vi "MainKinetics.vi"() -> ()   [LabVIEW 2017]
uses:
  <vilib>/Utility/miscctls.llb/LVRowAndColumnTypeDef.ctl
  <vilib>/Utility/sysdir.llb/System Directory Type.ctl
  <vilib>/Utility/config.llb/Read Key (String).vi
  <vilib>/Utility/config.llb/Write Key (String).vi
  <vilib>/Utility/cursorutil.llb/Set Cursor (Icon Pict).vi
  PCAN_Driver/ControlCAN.lvlib
  <vilib>/Utility/config.llb/NI_LVConfig.lvlib
panel:
  out "CurrentSens":bool
  out "CurrentOut":dbl
  out "Current":string
  out "VISA Current":refnum<visa-resource-name>
  out "Offset":dbl
  out "Analogtest":bool=TRUE
  out "TestinExecution":string
  out "FullSpeed2 Current":dbl
  out "FullSpeed1 Current":dbl
  out "String":string
  out "ParamVersion":string
  out "DSP Board S/N":string
  out "POWER Board S/N":string caption="DRIVER Board S/N"
  in  "EventTimeout":i32=100
  out "SpeedLimit":dbl[](array[numeric])
  out "TestArray":string[](array[string])
  out "Motor Speed RPM Serial":dbl
  out "DAQmx Device Name":tag
  out "PN":string
  out "FileName":string
  out "VenableSpeed":u16
  out "TesterVersion":string
  out "ClosePanel":bool=TRUE
  out "UUT SN Report":string
  out "Automation":bool
  out "Test Failed":bool
  out "VisualInspectionResult":bool
  out "MotorTempResult":bool
  out "VenableDirectionResult":bool
  out "VenableResult":bool
  out "ComTestResult":bool=TRUE
  out "UUT SoftwareVer":string
  out "Next SN":i32
  in  "SetSN":bool
  out "Current SN":i32
  out "FullSpeed2 Speed":dbl
  out "FullSpeed2 Current":dbl
  out "FullSpeed1 Current":dbl
  out "FullSpeed1 Speed":dbl
  out "UUT":u8
  out "CAN Status":bool
  out "Array":u64[][](array[numeric]) format="%016x"
  out "Motor Phase Current RMS":dbl
  out "Ambient Temperature":dbl
  out "Speed error":bool
  out "Commutation err":bool
  out "Under voltage/Over voltage":bool
  out "Derated drive temp":bool
  out "Motor Over temperature":bool
  out "Motor Sensor temp Fauilre":bool
  out "Drive Over temperature":bool
  out "Drive Sensor temp Failure":bool
  out "Ambient Over temp":bool
  out "Ambient Sensor temp":bool
  out "DC Voltage":dbl
  out "DC Current":dbl
  out "Power transistor Heat sink Temp.":dbl
  out "Motor Stator Temp.":dbl
  out "Motor Speed RPM":dbl
  out "ECS State":u16
  out "UUT":string="EBAY"
  in  "Logger Path":path
  in  "Report":bool
  in  "Start":bool
  in  "ATR":string[][](table)=[["Test Communication", "-", "-", "-", "-", ""], ["Set S/N", "-", "-", "-", "-", ""], ["Set Board Number", "-", "-", "-", "-", ""], [" ", "", "", "", "", ""], ["Test Communication", "-", "-", "-", "-", ""], ["Get S/N", "-", "-", "-", "", ""], ["Get Board Number", "-", "-", "-", "", ""], ["Get FW", "-", "-", "-", "", ""], ["Enable Motor", "", "", "", "", ""], ["Small position command", "", "", "", "", ""], ["Measure delta", "", "", "", "", ""], ["Velocity command", "", "", "", "", ""]]
  in  "Settings":bool
  in  "Refresh Button":bool
  out "Serial Status":bool
  in  "VISA Kinetics":refnum<visa-resource-name>="COM6"
  in  "Serial Com":bool
  in  "Help Button":bool
  out "Pannel User Message":string
  in  "Stop Button":bool
  # "Kinetics"
  # "REDLER TECHNOLOGIES LTD"
  # "ver 1.2p"
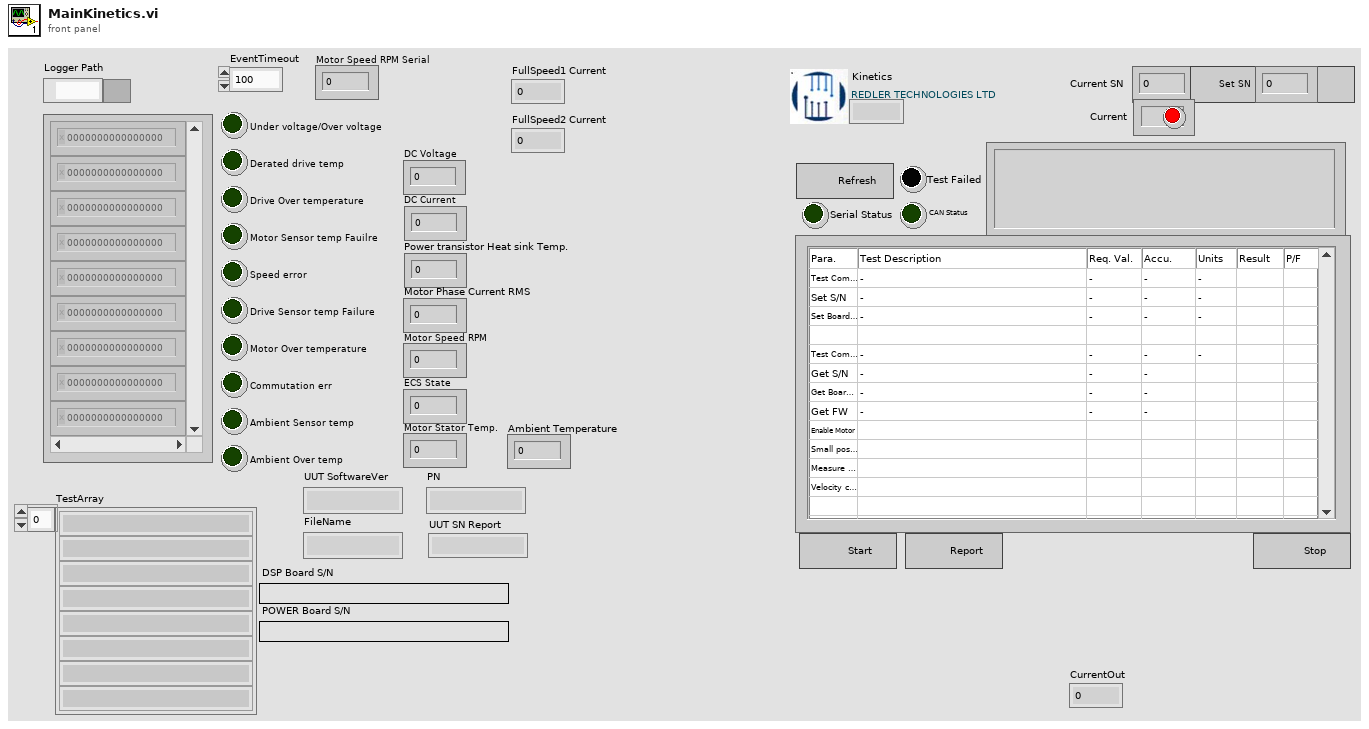
[diagram p1: front panel]
types:
  T1 = cluster{"VISA":refnum<visa-resource-name>, "TestArray":string[]}
  T2 = cluster{"ID":u32, "MSGTYPE":u8, "LEN":u8, "aDATA":u8[]}[]
  T3 = enum16{"Erase ATR Table", "Stop", "MainProgram", "Initialize"}
  T4 = typedef "NI_LVConfig.lvlib/Config Data RefNum.ctl" = refnum<k1>
  T5 = enum16{"Init", "0 ohm", "6 ohm", "13.2 ohm", "15 ohm", "25.9 ohm", "33 ohm", "Down", "Up", "Venable", "Firmware", "PowerSuply"}
  T6 = enum16{"Wait", "Exit", "VC=0", "ReadVC", "VC=1000"}
  T7 = enum16{"Stop", "Result", "FullSpeed2", "MD[1]=1", "FullSpeed1", "MD[1]=0"}
  T8 = enum16{"K15", "K16", "K17", "Venable", "Firmeware", "Fan", "Power", "120C", "110C", "100C", "90C", "80C", "70C", "60C", "50C", "40C", "30C", "25C", "20C", "10C", "0C"}
  T9 = enum8{"Term1", "Term2", "Current", "Fan", "TempCPU"}
  T10 = enum16{"Exit", "AI0/3", "AO0", "Wait", "Read", "Init"}
  T11 = enum16{"Exit", "Wait", "ReadCurrent", "ReadTemp", "Init"}
  T12 = enum16{"Init", "0 ohm", "6 ohm", "13.2 ohm", "15 ohm", "25.9 ohm", "33 ohm", "Down", "Up", "Venable", "Firmware", "PowerSuply"}[]
  T13 = enum8{"Enabled", "Disabled", "Disabled and Grayed Out"}
  T14 = typedef "LVRowAndColumnTypeDef.ctl" = cluster{"Row":i32, "Column":i32}
  T15 = enum32{"Invalid", "Standard", "Closed", "Hidden", "Minimized", "Maximized"}
  T16 = cluster{"ID":u32, "MSGTYPE":u8, "LEN":u8, "aDATA":u8[]}
  T17 = enum16{"open", "replace", "create", "open or create", "replace or create", "replace or create with confirmation"}
  T18 = typedef "ControlCAN.lvlib/DevType.ctl" = u32
  T19 = typedef "ControlCAN.lvlib/CAN Channel.ctl" = u32
  T20 = typedef "ControlCAN.lvlib/VCI_INIT_CONFIG.ctl" = cluster{"AccCode":u32, "AccMask":u32, "InitFlag":T21, "Fliter":T22, "Timing0":u8, "Timing1":u8, "Mode":T23}
  T21 = typedef "ControlCAN.lvlib/InitFlag.ctl" = u32
  T22 = typedef "ControlCAN.lvlib/Fliter.ctl" = u8
  T23 = typedef "ControlCAN.lvlib/Mode.ctl" = u8
  T24 = cluster{"DevType":T18, "DevIndex":u32, "CanIndex":T19, "VCI_INIT_CONFIG":T20}
  T25 = typedef "ControlCAN.lvlib/VCI_CAN_OBJ.ctl" = cluster{"ID":u32, "TimeStamp":u32, "TimeFlag":u8, "SendType":u8, "RemoteFlag":u8, "ExternFlag":u8, "DataLen":u8, "Data":u8[], "Reserved":u8[]}
  T26 = cluster{"Type":enum16{"接收", "发送"}, "Channel":T19, "Time":timestamp, "VCI_CAN_OBJ":T25}[]
  T27 = cluster{"Type":enum16{"接收", "发送"}, "Channel":T19, "Time":timestamp, "VCI_CAN_OBJ":T25}
  T28 = typedef "LVPoint32TypeDef.ctl" = cluster{"Horizontal":i32, "Vertical":i32}
  T29 = typedef "System Directory Type.ctl" = i32
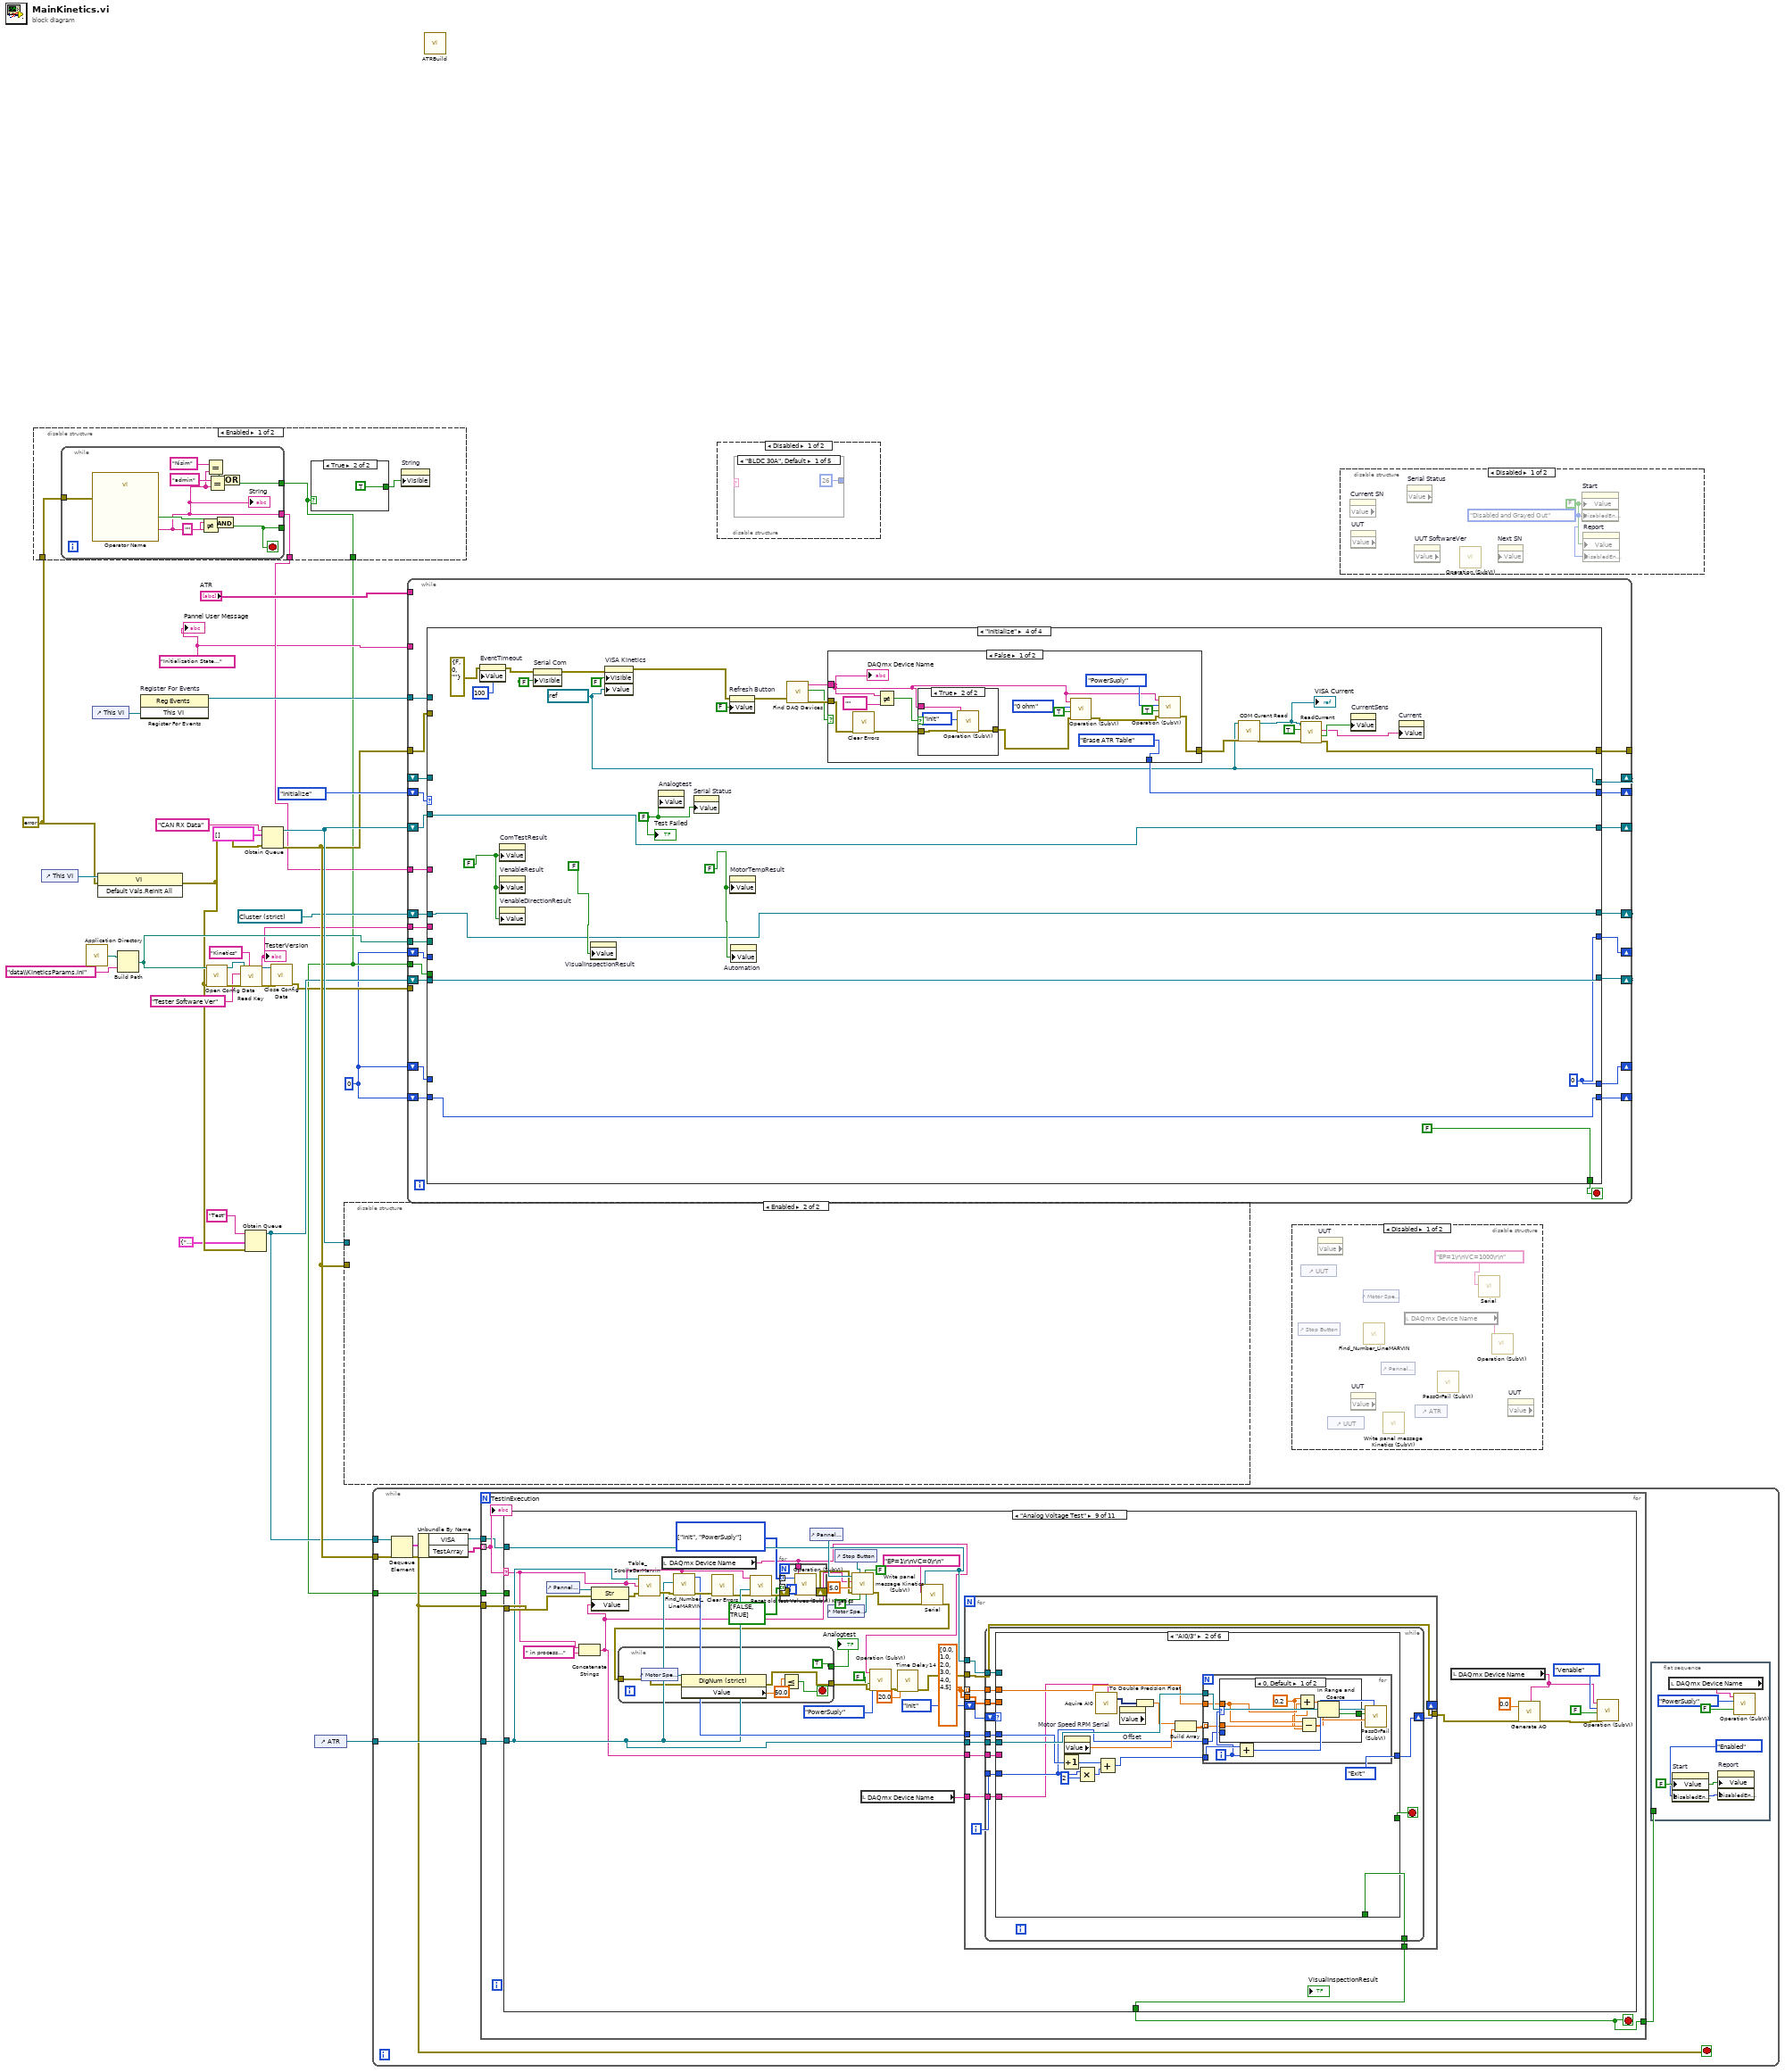
[diagram p0: block diagram]
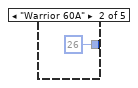
[diagram p2: hidden frame]
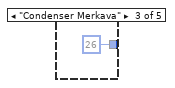
[diagram p3: hidden frame]
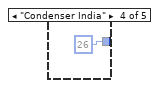
[diagram p4: hidden frame]
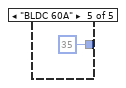
[diagram p5: hidden frame]
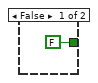
[diagram p7: hidden frame]
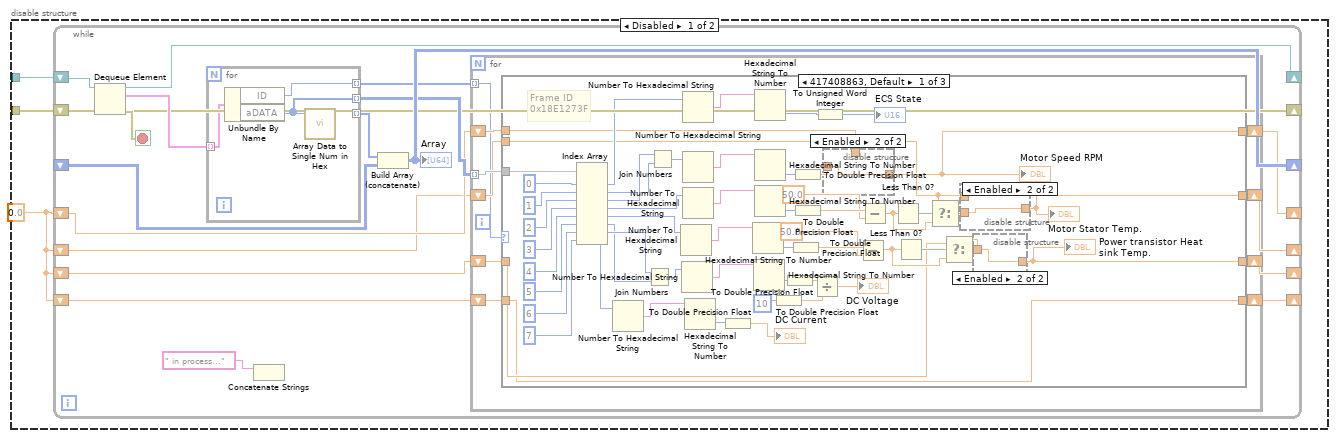
[diagram p9: hidden frame]
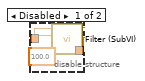
[diagram p10: hidden frame]
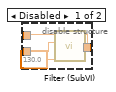
[diagram p11: hidden frame]
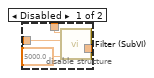
[diagram p12: hidden frame]
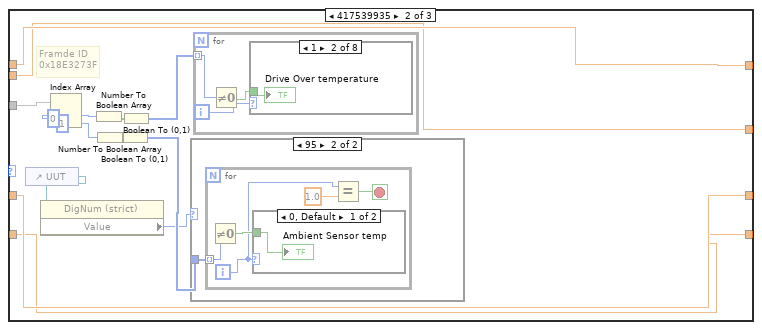
[diagram p13: hidden frame]
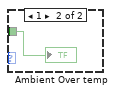
[diagram p15: hidden frame]
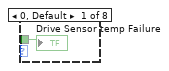
[diagram p16: hidden frame]
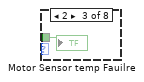
[diagram p17: hidden frame]
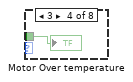
[diagram p18: hidden frame]
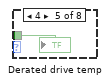
[diagram p19: hidden frame]
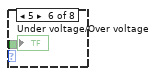
[diagram p20: hidden frame]
diagram:
  w17 = "Initialization State..."
  w2 = 0
  w5 = errorcluster {"status"=FALSE, "code"=0, "source"=""} ("error in (no error)")
  n1 = disable-structure shown="Enabled" {
    disable-tunnel: [w35 _] -> w18
    disable-tunnel: w5 -> [w33 _]
    disable-tunnel: [w32 _] -> w3
    frame Enabled {
      n2 = while {
        tunnel: [w45] -> _
        tunnel: [w38] -> w35
        tunnel: [w42] -> w32
        tunnel: w33 -> [w39]
        stop <- w45 stop-if-true
        n3 = call "Operator Name"("error in (no error)"=w39) -> ("Operator Name"=w38:string, "OK"=w46:bool)  [unwired: 16 in, 1 out]
        "String" <- w38
        n4 = Not Equal?(x=w38, y="") -> (x != y?=w47:bool)
        n5 = Equal?(x="Nisim", y=w38) -> (x = y?=w40:bool)
        n6 = Equal?(x="admin", y=w38) -> (x = y?=w43:bool)
        n7 = And(x=w46, y=w47) -> (x .and. y?=w45:bool)
        n8 = Or(x=w40, y=w43) -> (x .or. y?=w42:bool)
      }
      n9 = case shown="True" w32 {
        tunnel: [FALSE TRUE] -> w34
        frame False {
        }
        frame True {
        }
      }
      n10 = property on="String" class="Str"("Visible"=w34) -> ()  [unwired: 2 in, 2 out]
    }
    frame Disabled {
    }
  }
  n11 = control-ref of="This VI"() -> (w6:refnum<vi>)
  n12 = call <vilib>:"Application Directory.vi"() -> ("Application Directory"=w22:path)
  n13 = control-ref of="This VI"() -> (w20:refnum<vi>)
  n14 = invoke class="VI" method="Default Vals.Reinit All"(reference=w6, error in=w5) -> (error out=w4:errorcluster)  [unwired: 1 in, 2 out]
  n15 = Build Path(base path=w22, name or relative path="data\\KineticsParams.ini") -> (appended path=w9:path)
  n16 = register-events "Register For Events"(w20) -> (reference out=w19:refnum<event-registration>)  [unwired: 2 in, 1 out]
  n17 = call <vilib>:"Open Config Data.vi"("error in (no error)"=w4, "configuration file path"=w9) -> ("error out"=w15:errorcluster, "refnum"=w14:T4)  [unwired: 1 in, 7 out]
  n18 = call-poly <vilib>:"Read Key.vi"("section"="Kinetics", "error in (no error)"=w15, "key"="Tester Software Ver", "refnum"=w14) -> ("error out"=w12:errorcluster, "value"=w7:string, "refnum out"=w11:T4)  [unwired: 2 in, 3 out]
  "TesterVersion" <- w7
  n19 = Obtain Queue(name (unnamed)="Test", element data type=T1 {"VISA"="COM1", "TestArray"=[]}, error in (no error)=w4) -> (queue out=w25:refnum<queue>)  [unwired: 2 in, 2 out]
  n20 = Obtain Queue(name (unnamed)="CAN RX Data", element data type=T2 [], error in (no error)=w4) -> (queue out=w28:refnum<queue>, error out=w26:errorcluster)  [unwired: 2 in, 1 out]
  n21 = call <vilib>:"Close Config Data.vi"("error in (no error)"=w12, "refnum"=w11) -> ("error out"=w10:errorcluster)  [unwired: 8 in, 1 out]
  n22 = control-ref of="ATR"() -> (w16:refnum<vi>)
  n23 = disable-structure shown="Enabled" {
    disable-tunnel: w28 -> [w51 _]
    disable-tunnel: w26 -> [w50 _]
    frame Disabled {
      w49 = 0.0
      n24 = while {
        shift-right: [w68] -> _
        shift-left: w51 -> [w70]
        shift-right: [w66] -> _
        shift-left: _ -> [w67]
        shift-right: [w62] -> _
        shift-left: w50 -> [w62]
        shift-right: [w60] -> _
        shift-left: w49 -> [w61]
        shift-right: [w59] -> _
        shift-left: w49 -> [w58]
        shift-right: [w57] -> _
        shift-left: w49 -> [w56]
        shift-right: [w55] -> _
        shift-left: w49 -> [w54]
        stop <- w69 stop-if-true
        n25 = Dequeue Element(queue=w70, error in (no error)=w62) -> (queue out=w68:refnum<queue>, element=w63:T2, error out=w69:errorcluster)  [unwired: 1 in, 1 out]
        n26 = for {
          tunnel: [w216] -> w65 mode=indexing
          tunnel: w63 -> [w215] mode=indexing
          tunnel: [w214] -> w64 mode=indexing
          tunnel: [w213] -> w53 mode=indexing
          n27 = Unbundle By Name(w215) -> ("ID"=w213:u32, "aDATA"=w214:u8[])
          n28 = call "Array Data to Single Num in Hex.vi"("aDATA"=w214) -> ("Numeric"=w216:u64)  [unwired: 10 in]
        }
        n29 = Concatenate Strings(" in process..." ("Strin")) -> ()  [unwired: 1 in, 1 out]
        n30 = Build Array (concatenate)(w65, w67) -> (w66:u64[][])
        "Array" <- w66
        n31 = for {
          tunnel: w64 -> [w80] mode=indexing
          shift-right: [w78] -> w60
          shift-left: w61 -> [w79]
          shift-right: [w77] -> w59
          shift-left: w58 -> [w76]
          shift-right: [w75] -> w57
          shift-left: w56 -> [w74]
          shift-right: [w73] -> w55
          shift-left: w54 -> [w72]
          tunnel: w53 -> [w71] mode=indexing
          n32 = case shown="417408863, Default" w71 {
            tunnel: w80 -> [w117 w165 w203]
            tunnel: w79 -> [w91 w154 w192]
            tunnel: [w90 w154 w192] -> w78
            tunnel: [w87 w153 w191] -> w77
            tunnel: w76 -> [w86 w153 w191]
            tunnel: [w83 w152 w190] -> w75
            tunnel: w74 -> [w82 w152 w190]
            tunnel: [w81 w151 w186] -> w73
            tunnel: w72 -> [w81 w151 w185]
            frame 417408863, Default {
              # "Frame ID\n0x18E1273F"
              n33 = Index Array(array=w117, index #1=0 ("index"), index #2=1 ("index"), index #3=2 ("index"), index #4=3 ("index"), index #5=4 ("index"), index #6=5 ("index"), index #7=6 ("index"), index #8=7 ("index")) -> (element #1=w101:u8, element #2=w103:u8, element #3=w104:u8, element #4=w108:u8, element #5=w111:u8, element #6=w115:u8, element #7=w116:u8, element #8=w114:u8)
              n34 = Number To Hexadecimal String(2:w114) -> (0:w128:string)  [unwired: 1 in]
              n35 = Join Numbers(hi=w116, lo=w115) -> ((hi.lo)=w135:u16)
              n36 = Join Numbers(hi=w104, lo=w103) -> ((hi.lo)=w105:u16)
              n37 = Number To Hexadecimal String(2:w111) -> (0:w112:string)  [unwired: 1 in]
              n38 = Number To Hexadecimal String(2:w135) -> (0:w134:string)  [unwired: 1 in]
              n39 = Number To Hexadecimal String(2:w101) -> (0:w102:string)  [unwired: 1 in]
              n40 = Number To Hexadecimal String(2:w105) -> (0:w106:string)  [unwired: 1 in]
              n41 = Number To Hexadecimal String(2:w108) -> (0:w109:string)  [unwired: 1 in]
              n42 = Hexadecimal String To Number(string=w128) -> (number=w127:u32)  [unwired: 2 in, 1 out]
              n43 = To Double Precision Float(number=w127) -> (double precision float=→"DC Current":dbl)
              n44 = Hexadecimal String To Number(string=w112) -> (number=w113:u32)  [unwired: 2 in, 1 out]
              n45 = Hexadecimal String To Number(string=w134) -> (number=w133:u32)  [unwired: 2 in, 1 out]
              n46 = Hexadecimal String To Number(string=w102) -> (number=w99:u32)  [unwired: 2 in, 1 out]
              n47 = Hexadecimal String To Number(string=w106) -> (number=w107:u32)  [unwired: 2 in, 1 out]
              n48 = Hexadecimal String To Number(string=w109) -> (number=w110:u32)  [unwired: 2 in, 1 out]
              n49 = To Double Precision Float(number=u32 10 ("y")) -> (double precision float=w131:dbl)
              n50 = To Double Precision Float(number=w133) -> (double precision float=w130:dbl)
              n51 = To Double Precision Float(number=w113) -> (double precision float=w96:dbl)
              n52 = To Double Precision Float(number=w107) -> (double precision float=w92:dbl)
              n53 = To Double Precision Float(number=w110) -> (double precision float=w98:dbl)
              n54 = Divide(x=w130, y=w131) -> (x/y=→"DC Voltage":dbl)
              n55 = To Unsigned Word Integer(number=w99) -> (unsigned 16bit integer=→"ECS State":u16)
              n56 = disable-structure shown="Enabled" {
                disable-tunnel: w92 -> [w149 w150]
                disable-tunnel: w91 -> [w148 _]
                disable-tunnel: [w146 w150] -> w90
                frame Disabled {
                  n57 = call "Filter (SubVI).vi"("Delta"=5000.0, "NewVal"=w149, "OldVal"=w148) -> ("Val"=w146:dbl)  [unwired: 8 in]
                }
                frame Enabled {
                }
              }
              "Motor Speed RPM" <- w90
              n58 = Subtract(x=w96, y=50.0 ("x")) -> (x-y=w85:dbl)
              n59 = Subtract(x=w98, y=50.0 ("x")) -> (x-y=w88:dbl)
              n60 = Less Than 0?(x=w88) -> (x < 0?=w94:bool)
              n61 = Less Than 0?(x=w85) -> (x < 0?=w93:bool)
              n62 = Select(t=w86, s=w94, f=w88) -> (s? t:f=w89:dbl)
              n63 = Select(t=w82, s=w93, f=w85) -> (s? t:f=w84:dbl)
              n64 = disable-structure shown="Enabled" {
                disable-tunnel: w89 -> [w144 w145]
                disable-tunnel: [w143 w145] -> w87
                disable-tunnel: w86 -> [w142 _]
                frame Disabled {
                  n65 = call "Filter (SubVI).vi"("Delta"=130.0, "NewVal"=w144, "OldVal"=w142) -> ("Val"=w143:dbl)  [unwired: 8 in]
                }
                frame Enabled {
                }
              }
              "Motor Stator Temp." <- w87
              n66 = disable-structure shown="Enabled" {
                disable-tunnel: w84 -> [w139 w140]
                disable-tunnel: [w137 w140] -> w83
                disable-tunnel: w82 -> [w136 _]
                frame Disabled {
                  n67 = call "Filter (SubVI).vi"("Delta"=100.0, "NewVal"=w139, "OldVal"=w136) -> ("Val"=w137:dbl)  [unwired: 8 in]
                }
                frame Enabled {
                }
              }
              "Power transistor Heat sink Temp." <- w83
            }
            frame 417539935 {
              # "Framde ID\n0x18E3273F"
              n68 = control-ref of="UUT"() -> (w155:refnum<vi>)
              n69 = property on="Property Node" class="DigNum (strict)"(reference=w155) -> ("Value"=w156:u8)  [unwired: 1 in, 2 out]
              n70 = Index Array(array=w165, index #1=0 ("index"), index #2=1 ("index")) -> (element #1=w163:u8, element #2=w158:u8)
              n71 = Number To Boolean Array(number=w163) -> (Boolean array=w162:bool[])
              n72 = Number To Boolean Array(number=w158) -> (Boolean array=w160:bool[])
              n73 = Boolean To (0,1)(Boolean=w160) -> (0, 1=w157:i16[])
              n74 = Boolean To (0,1)(Boolean=w162) -> (0, 1=w161:i16[])
              n75 = case shown="95" w156 {
                tunnel: w157 -> [_ w166]
                frame 0, Default {
                }
                frame 95 {
                  n76 = for {
                    tunnel: w166 -> [w171] mode=indexing
                    i -> [w167]
                    stop <- w169 stop-if-true
                    n77 = Not Equal To 0?(x=w171) -> (x != 0?=w170:bool)
                    n78 = case shown="0, Default" w167 {
                      tunnel: w170 -> [w172 w173]
                      frame 0, Default {
                        "Ambient Sensor temp" <- w172
                      }
                      frame 1 {
                        "Ambient Over temp" <- w173
                      }
                    }
                    n79 = Equal?(x=w167, y=1.0) -> (x = y?=w169:bool)
                  }
                }
              }
              n80 = for {
                tunnel: w161 -> [w175] mode=indexing
                i -> [w176]
                n81 = Not Equal To 0?(x=w175) -> (x != 0?=w174:bool)
                n82 = case shown="1" w176 {
                  tunnel: w174 -> [w177 w178 w179 w180 w181 w182 w183 w184]
                  frame 0, Default {
                    "Drive Sensor temp Failure" <- w177
                  }
                  frame 1 {
                    "Drive Over temperature" <- w178
                  }
                  frame 2 {
                    "Motor Sensor temp Fauilre" <- w179
                  }
                  frame 3 {
                    "Motor Over temperature" <- w180
                  }
                  frame 4 {
                    "Derated drive temp" <- w181
                  }
                  frame 5 {
                    "Under voltage/Over voltage" <- w182
                  }
                  frame 6 {
                    "Commutation err" <- w183
                  }
                  frame 7 {
                    "Speed error" <- w184
                  }
                }
              }
            }
            frame 417474399 {
              # "Frame ID\n0x18E2273F"
              n83 = Index Array(array=w203, index #1=0 ("index"), index #2=1 ("index")) -> (element #1=w200:u8, element #2=w197:u8)
              n84 = disable-structure shown="Enabled" {
                disable-tunnel: [w211 w212] -> w201
                disable-tunnel: w200 -> [w210 w212]
                frame Disabled {
                  n85 = Number To Hexadecimal String(2:w210) -> (0:w209:string)  [unwired: 1 in]
                  n86 = Hexadecimal String To Number(string=w209) -> (number=w211:u32)  [unwired: 2 in, 1 out]
                }
                frame Enabled {
                }
              }
              n87 = Number To Hexadecimal String(2:w197) -> (0:w195:string)  [unwired: 1 in]
              n88 = Hexadecimal String To Number(string=w195) -> (number=w196:u32)  [unwired: 2 in, 1 out]
              n89 = To Double Precision Float(number=w196) -> (double precision float=w194:dbl)
              n90 = To Double Precision Float(number=w201) -> (double precision float=→"Motor Phase Current RMS":dbl)
              n91 = Subtract(x=w194, y=50.0) -> (x-y=w188:dbl)
              n92 = Less Than 0?(x=w188) -> (x < 0?=w189:bool)
              n93 = Select(t=w185, s=w189, f=w188) -> (s? t:f=w187:dbl)
              n94 = disable-structure shown="Disabled" {
                disable-tunnel: w187 -> [w207 w208]
                disable-tunnel: [w205 w208] -> w186
                disable-tunnel: w185 -> [w204 _]
                frame Disabled {
                  n95 = call "Filter (SubVI).vi"("Delta"=65.0, "NewVal"=w207, "OldVal"=w204) -> ("Val"=w205:dbl)  [unwired: 8 in]
                }
                frame Enabled {
                }
              }
              "Ambient Temperature" <- w186
            }
          }
        }
      }
    }
    frame Enabled {
    }
  }
  n96 = while {
    tunnel: w16 -> [w225]
    tunnel: w26 -> [w223]
    tunnel: w25 -> [w224]
    tunnel: w3 -> [w218]
    stop <- w220 stop-if-true
    n97 = Dequeue Element(queue=w224, error in (no error)=w223) -> (element=w222:T1, error out=w220:errorcluster)  [unwired: 1 in, 2 out]
    n98 = Unbundle By Name(w222) -> ("VISA"=w221:refnum<visa-resource-name>, "TestArray"=w217:string[])
    n99 = for {
      tunnel: w217 -> [w235] mode=indexing
      tunnel: w221 -> [w233]
      tunnel: w225 -> [w232]
      tunnel: w220 -> [w236]
      tunnel: [w231] -> w219
      tunnel: w218 -> [w234]
      stop <- w231 stop-if-true
      n100 = case shown="\"Analog Voltage Test\"" w235 {
        selector: w235 -> [_ w254 w671 w1132 w1271 w1418 w1503 w1587 w1678 w1839 w1969]
        tunnel: w232 -> [_ w247 _ _ w1265 w1412 w1497 w1581 w1679 w1847 w1967]
        tunnel: w236 -> [_ w257 _ _ w1278 w1417 w1502 w1586 w1680 w1854 w1971]
        tunnel: w234 -> [_ _ _ _ _ _ _ _ _ _ _]
        tunnel: w233 -> [_ w250 w670 w1131 w1268 w1406 w1494 w1572 w1656 w1840 w1968]
        tunnel: [TRUE ("Stopped") w242 w669 w1121 w1261 w1401 w1487 w1574 w1670 w1838 FALSE ("Stopped")] -> w231
        frame "", Default {
        }
        frame "Comm. & Motor Test" {
          n101 = control-ref of="Pannel User Message"() -> (w258:refnum<vi>)
          n102 = Concatenate Strings(w254, " in process..." ("string")) -> (w249:string)
          n103 = property class="Str"(reference=w258, error in=w257, "Value"=w249) -> (error out=w256:errorcluster)  [unwired: 1 out]
          n104 = call "Table_ScrollaBarMarvin.vi"("error in"=w256, "Line to focus"=w254, "reference in"=w247) -> ("error out"=w253:errorcluster)  [unwired: 2 out]
          n105 = call "Find_Number_LineMARVIN.vi"("Test Paragraph"=w254, "error in"=w253, "TableIn"=w247) -> ("error out"=w259:errorcluster, "Line number"=w238:i32)  [unwired: 2 in, 2 out]
          n106 = property on="UUT" class="Str"() -> ("Value"=w246:string)  [unwired: 2 in, 2 out]
          n107 = Concatenate Strings("- Set the FIREWERE switch to OFF position." ("Screen Line"), "- Set the VENABLE switch to ON position." ("Screen Line")) -> (w243:string)
          n108 = call <vilib>:"Clear Errors.vi"("error in (no error)"=w259) -> ("error out"=w252:errorcluster)  [unwired: 5 in, 1 out]
          n109 = Add(x=3, y=w238) -> (x+y=w248:i32)
          n110 = call "Reset old test Values (SubVI) Kinetics.vi"("error in"=w252, "Atr in"=w247, "Test Paragraph"=w254) -> ("error out"=w241:errorcluster)  [unwired: 6 in, 2 out]
          n111 = case shown="\"Condenser India\", \"Condenser Merkava\"" w246 {
            tunnel: w243 -> [_ w668]
            tunnel: w241 -> [w666 w667]
            tunnel: [w666 w667] -> w240
            frame "False", Default {
            }
            frame "Condenser India", "Condenser Merkava" {
              n112 = One Button Dialog(message=w668) -> ()  [unwired: 1 in, 1 out]
            }
          }
          n113 = for {
            N: 2 -> [_]
            tunnel: w250 -> [w267]
            tunnel: w249 -> [w266]
            tunnel: w248 -> [w265]
            tunnel: w247 -> [w264]
            tunnel: [w263] -> w242
            tunnel: w240 -> [w262]
            tunnel: w238 -> [w260]
            i -> [w261]
            n114 = case shown="1" w261 {
              tunnel: w267 -> [w285 w376]
              tunnel: w266 -> [w284 w375]
              tunnel: w265 -> [w282 _]
              tunnel: w264 -> [w275 w373]
              tunnel: [w280 w377] -> w263
              tunnel: w262 -> [w271 _]
              tunnel: w260 -> [w277 _]
              frame 0, Default {
                n115 = Increment(x=w277) -> (x+1=w270:i32)
                n116 = property on="Serial Status" class="Bool (strict)"() -> ("Value"=w279:bool)  [unwired: 2 in, 2 out]
                n117 = property on="UUT SoftwareVer" class="Str"() -> ("Value"=w268:string)  [unwired: 2 in, 2 out]
                n118 = call "PassOrFail (SubVI).vi"("String Res"=w268, "index (row)"=w270, "error in (no error)"=w271, "Data in"=-3.0, "Pass?Fail"=w279, "Table in"=w275) -> ("error out"=w273:errorcluster)  [unwired: 5 in]
                n119 = Increment(x=w270) -> (x+1=w269:i32)
                n120 = property on="CAN Status" class="Bool (strict)"() -> ("Value"=w274:bool)  [unwired: 2 in, 2 out]
                n121 = call "PassOrFail (SubVI).vi"("String Res"=w268, "index (row)"=w269, "error in (no error)"=w273, "Data in"=-3.0, "Pass?Fail"=w274, "Table in"=w275) -> ("error out"=w272:errorcluster)  [unwired: 5 in]
                n122 = while {
                  shift-right: [w296] -> _
                  shift-left: T6."VC=1000" -> [w299]
                  tunnel: w272 -> [w298]
                  tunnel: w285 -> [w297]
                  tunnel: w284 -> [w295]
                  shift-right: [w292] -> w281
                  shift-left: bool[] [FALSE, FALSE] -> [w293]
                  tunnel: w282 -> [w291]
                  tunnel: w275 -> [w290]
                  tunnel: [w288] -> w280
                  i -> [w294]
                  stop <- w289 stop-if-true
                  n123 = case shown="\"VC=0\"" w299 {
                    tunnel: w298 -> [_ w322 _ w353 _]
                    tunnel: w297 -> [w302 w320 w329 w357 _]
                    tunnel: [T6."Exit" T6."Wait" w326 T6."Wait" T6."ReadVC"] -> w296
                    tunnel: w295 -> [_ _ _ _ w365]
                    tunnel: [TRUE FALSE FALSE FALSE FALSE] -> w289
                    tunnel: w294 -> [_ _ w327 _ w360]
                    tunnel: w293 -> [w301 w317 w325 w355 w362]
                    tunnel: [w301 w317 w324 w355 w362] -> w292
                    tunnel: w291 -> [w310 _ _ _ _]
                    tunnel: w290 -> [w312 _ _ _ _]
                    tunnel: [_ _ _ _ w359] -> w288
                    frame "Exit", Default {
                      n124 = And Array Elements(Boolean array=w301) -> (logical AND=w305:bool)
                      n125 = local read "DAQmx Device Name"() -> (w309:tag)
                      n126 = Select(t="OK", s=w305, f="Failed") -> (s? t:f=w311:string)
                      n127 = call "PassOrFail (SubVI).vi"("String Res"=w311, "index (row)"=w310, "Data in"=-3.0, "Pass?Fail"=w305, "Table in"=w312) -> ("error out"=w300:errorcluster)  [unwired: 6 in]
                      n128 = call "Serial.vi"("error in (no error)"=w300, "write buffer"="EP=1\r\nVC=0\r\n", "VISA resource name"=w302) -> ("error out"=w303:errorcluster)  [unwired: 7 in, 1 out]
                      n129 = call "Operation (SubVI).vi"("error in (no error)"=w303, "On/Off"=FALSE, "Operation"=T5."Venable", "DAQmx Device Name"=w309) -> ()  [unwired: 7 in, 1 out]
                    }
                    frame "VC=0" {
                      n130 = call "Serial.vi"("error in (no error)"=w322, "write buffer"="EP=1\r\nVC=0\r\n", "VISA resource name"=w320) -> ()  [unwired: 7 in, 2 out]
                    }
                    frame "ReadVC" {
                      n131 = call "Serial.vi"("write buffer"="VC\r\n", "VISA resource name"=w329) -> ("read buffer"=w328:string)  [unwired: 8 in, 1 out]
                      n132 = case shown="5, Default" w327 {
                        tunnel: w328 -> [w338 w344]
                        tunnel: [T6."VC=0" T6."Exit"] -> w326
                        tunnel: w325 -> [w333 w343]
                        tunnel: [w331 w340] -> w324
                        frame 2 {
                          n133 = Decimal String To Number(string=w338) -> (number=w337:i32)  [unwired: 2 in, 1 out]
                          n134 = In Range and Coerce(upper limit=1100, x=w337, lower limit=900) -> (In Range?=w332:bool)  [unwired: 1 out]
                          n135 = Replace Array Subset(array=w333, new element=w332, index=0) -> (w331:bool[])
                        }
                        frame 5, Default {
                          n136 = Decimal String To Number(string=w344) -> (number=w347:i32)  [unwired: 2 in, 1 out]
                          n137 = In Range and Coerce(upper limit=100, x=w347, lower limit=0) -> (In Range?=w341:bool)  [unwired: 1 out]
                          n138 = Replace Array Subset(array=w343, new element=w341, index=1) -> (w340:bool[])
                        }
                      }
                    }
                    frame "VC=1000" {
                      n139 = local read "DAQmx Device Name"() -> (w354:tag)
                      n140 = call "Operation (SubVI).vi"("error in (no error)"=w353, "On/Off"=TRUE, "Operation"=T5."Venable", "DAQmx Device Name"=w354) -> ("error out"=w352:errorcluster)  [unwired: 7 in]
                      n141 = call "Serial.vi"("error in (no error)"=w352, "write buffer"="EP=1\r\nVC=1000\r\n", "VISA resource name"=w357) -> ()  [unwired: 7 in, 2 out]
                    }
                    frame "Wait" {
                      n142 = case shown="4" w360 {
                        tunnel: [25.0 ("Time to wait") 15.0 ("Time to wait")] -> w366
                        frame 4 {
                        }
                        frame 1, Default {
                        }
                      }
                      n143 = control-ref of="Motor Speed RPM Serial"() -> (w370:refnum<vi>)
                      n144 = control-ref of="Pannel User Message"() -> (w369:refnum<vi>)
                      n145 = control-ref of="Stop Button"() -> (w364:refnum<vi>)
                      n146 = call "Write panel message Kinetics (SubVI).vi"(4:"rpm"=w370, 5:"rpm"=TRUE ("rpm"), "PrintTime"=TRUE, "Stop"=w364, "Time to wait"=w366, "Strin"=w365, "String in"=w369) -> ("Stopped"=w359:bool)  [unwired: 3 in, 1 out]
                    }
                  }
                }
                n147 = And Array Elements(Boolean array=w281) -> (logical AND=→"ComTestResult":bool)
              }
              frame 1 {
                n148 = case shown="True" TRUE {
                  tunnel: [_ w399] -> w377
                  tunnel: w376 -> [w378 w398]
                  tunnel: w375 -> [_ w396]
                  tunnel: w373 -> [w384 _]
                  frame False {
                    n149 = Two Button Dialog(message="Is the motor run in he right direction?", 1:"No" ("F button name (\"Cancel\")"), 2:"Yes" ("T button name (\"OK\")")) -> (T button?=w380:bool)
                    n150 = call "Find_Number_LineMARVIN.vi"("Test Paragraph"="Motor Direction", "TableIn"=w384) -> ("Line number"=w395:i32)  [unwired: 3 in, 3 out]
                    n151 = Select(t="OK", s=w380, f="Failed") -> (s? t:f=w394:string)
                    n152 = call "PassOrFail (SubVI).vi"("String Res"=w394, "index (row)"=w395, "Data in"=-3.0, "Pass?Fail"=w380, "Table in"=w384) -> ("error out"=w392:errorcluster)  [unwired: 6 in]
                    n153 = call "Serial.vi"("error in (no error)"=w392, "write buffer"="EP=1\r\nVC=0\r\n", "VISA resource name"=w378) -> ("error out"=w393:errorcluster)  [unwired: 7 in, 1 out]
                    n154 = local read "DAQmx Device Name"() -> (w379:tag)
                    n155 = call "Operation (SubVI).vi"("error in (no error)"=w393, "On/Off"=FALSE, "Operation"=T5."Venable", "DAQmx Device Name"=w379) -> ()  [unwired: 7 in, 1 out]
                  }
                  frame True {
                    n156 = property on="UUT" class="Str"() -> ("Value"=w401:string)  [unwired: 2 in, 2 out]
                    n157 = case shown="\"BLDC 60A\"" w401 {
                      tunnel: [26 26 26 26 40] -> w402
                      tunnel: [_ _ _ _ 56] -> w403
                      tunnel: [_ _ _ _ "10800"] -> w397
                      frame "BLDC 30A", Default {
                      }
                      frame "Warrior 60A" {
                      }
                      frame "Condenser Merkava" {
                      }
                      frame "Condenser India" {
                      }
                      frame "BLDC 60A" {
                      }
                    }
                    n158 = local read "DAQmx Device Name"() -> (w407:tag)
                    n159 = control-ref of="Stop Button"() -> (w404:refnum<vi>)
                    n160 = control-ref of="ATR"() -> (w408:refnum<vi>)
                    n161 = control-ref of="Pannel User Message"() -> (w405:refnum<vi>)
                    n162 = control-ref of="Motor Speed RPM Serial"() -> (w406:refnum<vi>)
                    n163 = while {
                      shift-right: [w421] -> _
                      shift-left: T7."MD[1]=0" -> [w422]
                      tunnel: w404 -> [w420]
                      tunnel: w405 -> [w419]
                      tunnel: w406 -> [w418]
                      tunnel: w407 -> [w417]
                      tunnel: w402 -> [w416]
                      tunnel: w403 -> [w415]
                      tunnel: w408 -> [w414]
                      tunnel: [w409] -> w399
                      tunnel: w398 -> [w412]
                      tunnel: w397 -> [w411]
                      tunnel: w396 -> [w410]
                      stop <- w413 stop-if-true
                      n164 = case shown="\"FullSpeed2\"" w422 {
                        tunnel: [T7."Stop" T7."Stop" w488 w561 w585 w658] -> w421
                        tunnel: [TRUE w438 FALSE FALSE FALSE FALSE] -> w413
                        tunnel: w420 -> [_ w428 w473 w538 w571 w635]
                        tunnel: w419 -> [_ w427 w474 w539 w572 w636]
                        tunnel: w418 -> [_ w426 w475 w533 w574 w630]
                        tunnel: w417 -> [_ w430 w478 w525 _ w622]
                        tunnel: w416 -> [_ _ _ _ w573 _]
                        tunnel: w415 -> [_ _ w472 _ _ _]
                        tunnel: w414 -> [_ w440 _ _ _ _]
                        tunnel: w412 -> [_ w433 w468 w520 w569 w627]
                        tunnel: w411 -> [_ _ w467 _ w566 _]
                        tunnel: w410 -> [_ _ w465 w530 w564 w626]
                        tunnel: [_ _ w464 w521 w563 w617] -> w409
                        frame "Stop", Default {
                        }
                        frame "Result" {
                          n165 = property on="FullSpeed2 Current" class="DigNum (strict)"() -> ("Value"=w445:dbl)  [unwired: 2 in, 2 out]
                          n166 = property on="FullSpeed1 Current" class="DigNum (strict)"() -> ("Value"=w444:dbl)  [unwired: 2 in, 2 out]
                          n167 = Subtract(x=w445, y=w444) -> (x-y=w452:dbl)
                          n168 = call "Find_Number_LineMARVIN.vi"("Test Paragraph"="Motor Direction", "TableIn"=w440) -> ("Line number"=w449:i32)  [unwired: 3 in, 3 out]
                          n169 = Absolute Value(x=w452) -> (abs(x)=w447:dbl)
                          n170 = Greater Or Equal?(x=w447, y=u32 5) -> (x >= y?=w439:bool)
                          n171 = Select(t="OK", s=w439, f="Failed") -> (s? t:f=w441:string)
                          n172 = call "PassOrFail (SubVI).vi"("String Res"=w441, "index (row)"=w449, "Data in"=-3.0, "Pass?Fail"=w439, "Table in"=w440) -> ("error out"=w432:errorcluster)  [unwired: 6 in]
                          n173 = call "Serial.vi"("error in (no error)"=w432, "write buffer"="EP=1\r\nVC=0\r\n", "VISA resource name"=w433) -> ("error out"=w437:errorcluster)  [unwired: 7 in, 1 out]
                          n174 = call "Operation (SubVI).vi"("error in (no error)"=w437, "On/Off"=FALSE, "Operation"=T5."Venable", "DAQmx Device Name"=w430) -> ("error out"=w429:errorcluster)  [unwired: 7 in]
                          n175 = while {
                            tunnel: w429 -> [w460]
                            tunnel: w428 -> [w459]
                            tunnel: w427 -> [w458]
                            tunnel: w426 -> [w456]
                            tunnel: "Please wait untill RPM = 0." -> [w457]
                            stop <- w453 stop-if-true
                            n176 = property class="DigNum (strict)"(reference=w456) -> ("Value"=w455:dbl)  [unwired: 1 in, 2 out]
                            n177 = call "Write panel message Kinetics (SubVI).vi"(4:"rpm"=w456, 5:"rpm"=TRUE ("rpm"), "PrintTime"=FALSE, "Stop"=w459, "error in (no error)"=w460, "Time to wait"=0.2, "Strin"=w457, "String in"=w458) -> ()  [unwired: 2 in, 2 out]
                            n178 = Less Or Equal?(x=w455, y=50.0) -> (x <= y?=w453:bool)
                          }
                          n179 = Not(x=TRUE) -> (.not. x?=w438:bool)
                        }
                        frame "FullSpeed2" {
                          n180 = Search and Replace String(input string="EP=1\r\nVC=0\r\n" ("write buffer"), search string="0", replace string=w467) -> (result string=w471:string)  [unwired: 5 in, 3 out]
                          n181 = call "Serial.vi"("write buffer"=w471, "VISA resource name"=w468) -> ("error out"=w466:errorcluster)  [unwired: 8 in, 1 out]
                          n182 = Concatenate Strings(w465, "\nFull speed operation " ("string")) -> (w482:string)
                          n183 = call "Write panel message Kinetics (SubVI).vi"(4:"rpm"=w475, 5:"rpm"=TRUE ("rpm"), "PrintTime"=TRUE, "Stop"=w473, "error in (no error)"=w466, "Time to wait"=45.0, "Strin"=w482, "String in"=w474) -> ("error out"=w485:errorcluster, "Stopped"=w477:bool)  [unwired: 2 in]
                          n184 = flat-sequence {
                            tunnel: w485 -> [w492]
                            tunnel: [w492] -> w484
                            tunnel: [w491] -> w483
                            frame #0 {
                              n185 = call <vilib>:"High Resolution Relative Seconds.vi"() -> ("relative seconds"=w491:dbl)
                            }
                          }
                          n186 = while {
                            tunnel: w484 -> [_]
                            tunnel: [w514] -> _
                            tunnel: w472 -> [w518]
                            tunnel: w483 -> [w516]
                            tunnel: w482 -> [w512]
                            tunnel: w475 -> [w505]
                            tunnel: w478 -> [_]
                            tunnel: w477 -> [w509]
                            tunnel: [w497] -> w476
                            tunnel: w474 -> [w508]
                            tunnel: w473 -> [w507]
                            tunnel: [w500] -> w464
                            stop <- w519 stop-if-true
                            n187 = call <vilib>:"High Resolution Relative Seconds.vi"() -> ("relative seconds"=w517:dbl)
                            n188 = local read "CurrentOut"() -> (w499:dbl)
                            n189 = property class="DigNum (strict)"(reference=w505) -> ("Value"=w504:dbl)  [unwired: 1 in, 2 out]
                            n190 = Subtract(x=w517, y=w516) -> (x-y=w495:dbl)
                            n191 = Greater Or Equal?(x=w495, y=60.0) -> (x >= y?=w496:bool)
                            n192 = To Double Precision Float(number=w499) -> (double precision float=w498:dbl)
                            "FullSpeed2 Current" <- w498
                            n193 = Greater Or Equal?(x=w498, y=w518) -> (x >= y?=w506:bool)
                            n194 = Greater Or Equal?(x=w495, y=15.0) -> (x >= y?=w493:bool)
                            n195 = Greater Or Equal?(x=w504, y=10600.0) -> (x >= y?=w501:bool)
                            n196 = And(x=w506, y=w501) -> (x .and. y?=w502:bool)
                            n197 = call "Write panel message Kinetics (SubVI).vi"(4:"rpm"=w505, 5:"rpm"=TRUE ("rpm"), "PrintTime"=FALSE, "Stop"=w507, "Time to wait"=0.2, "Strin"=w512, "String in"=w508) -> ("error out"=w514:errorcluster, "Stopped"=w500:bool)  [unwired: 3 in]
                            n198 = Compound Arithmetic op=OR(w493, w500, w496) -> (w497:bool)
                            n199 = call "Display Message to User4"("Enable"=w493) -> ()  [unwired: 9 in, 2 out]
                            n200 = Compound Arithmetic op=OR(w493, w500, w509, w496, w502) -> (w519:bool)
                          }
                          n201 = Select(t=T7."Stop", s=w476, f=T7."Result") -> (s? t:f=w488:T7)
                        }
                        frame "MD[1]=1" {
                          n202 = call "Operation (SubVI).vi"("On/Off"=FALSE, "Operation"=T5."Venable", "DAQmx Device Name"=w525) -> ("error out"=w548:errorcluster)  [unwired: 8 in]
                          n203 = Concatenate Strings(w530, "\nSet Parameters MD[1]=1" ("Strin")) -> (w540:string)
                          n204 = call "Write panel message Kinetics (SubVI).vi"(4:"rpm"=w533, 5:"rpm"=FALSE ("rpm"), "PrintTime"=FALSE, "Stop"=w538, "error in (no error)"=w548, "Time to wait"=30.0, "Strin"=w540, "String in"=w539) -> ("error out"=w547:errorcluster, "Stopped"=w522:bool)  [unwired: 2 in]
                          n205 = call "Serial.vi"("error in (no error)"=w547, "write buffer"="EP=1\r\nVC=0\r\nMD[1]=1\r\n", "VISA resource name"=w520) -> ("error out"=w544:errorcluster)  [unwired: 7 in, 1 out]
                          n206 = call "Operation (SubVI).vi"("error in (no error)"=w544, "On/Off"=FALSE, "Operation"=T5."PowerSuply", "DAQmx Device Name"=w525) -> ("error out"=w543:errorcluster)  [unwired: 7 in]
                          n207 = call "Write panel message Kinetics (SubVI).vi"(4:"rpm"=w533, 5:"rpm"=FALSE ("rpm"), "PrintTime"=TRUE, "Stop"=w538, "error in (no error)"=w543, "Time to wait"=25.0, "Strin"=w540, "String in"=w539) -> ("error out"=w526:errorcluster, "Stopped"=w523:bool)  [unwired: 2 in]
                          n208 = call "Operation (SubVI).vi"("error in (no error)"=w526, "On/Off"=TRUE, "Operation"=T5."PowerSuply", "DAQmx Device Name"=w525) -> ("error out"=w527:errorcluster)  [unwired: 7 in]
                          n209 = call "Operation (SubVI).vi"("error in (no error)"=w527, "On/Off"=TRUE, "Operation"=T5."Venable", "DAQmx Device Name"=w525) -> ("error out"=w535:errorcluster)  [unwired: 7 in]
                          n210 = call "Write panel message Kinetics (SubVI).vi"(4:"rpm"=w533, 5:"rpm"=FALSE ("rpm"), "PrintTime"=TRUE, "Stop"=w538, "error in (no error)"=w535, "Time to wait"=3.0, "Strin"=w540, "String in"=w539) -> ("Stopped"=w524:bool)  [unwired: 2 in, 1 out]
                          n211 = Compound Arithmetic op=OR(w524, w523, w522) -> (w521:bool)
                          n212 = Compound Arithmetic op=OR(w524, w523, w522) -> (w532:bool)
                          n213 = Select(t=T7."Stop", s=w532, f=T7."FullSpeed2") -> (s? t:f=w561:T7)
                        }
                        frame "FullSpeed1" {
                          n214 = Search and Replace String(input string="EP=1\r\nVC=0\r\n" ("write buffer"), search string="0", replace string=w566) -> (result string=w565:string)  [unwired: 5 in, 3 out]
                          n215 = call "Serial.vi"("write buffer"=w565, "VISA resource name"=w569) -> ("error out"=w570:errorcluster)  [unwired: 8 in, 1 out]
                          n216 = Concatenate Strings(w564, "\nFull speed operation " ("string")) -> (w579:string)
                          n217 = call "Write panel message Kinetics (SubVI).vi"(4:"rpm"=w574, 5:"rpm"=TRUE ("rpm"), "PrintTime"=TRUE, "Stop"=w571, "error in (no error)"=w570, "Time to wait"=45.0, "Strin"=w579, "String in"=w572) -> ("error out"=w582:errorcluster, "Stopped"=w575:bool)  [unwired: 2 in]
                          n218 = flat-sequence {
                            tunnel: w582 -> [w589]
                            tunnel: [w589] -> w581
                            tunnel: [w588] -> w580
                            frame #0 {
                              n219 = call <vilib>:"High Resolution Relative Seconds.vi"() -> ("relative seconds"=w588:dbl)
                            }
                          }
                          n220 = while {
                            tunnel: w581 -> [_]
                            tunnel: [w611] -> _
                            tunnel: w573 -> [w615]
                            tunnel: w580 -> [w613]
                            tunnel: w579 -> [w609]
                            tunnel: w574 -> [w600]
                            tunnel: w575 -> [w605]
                            tunnel: [w594] -> w562
                            tunnel: w572 -> [w604]
                            tunnel: w571 -> [w603]
                            tunnel: [w596] -> w563
                            stop <- w616 stop-if-true
                            n221 = call <vilib>:"High Resolution Relative Seconds.vi"() -> ("relative seconds"=w614:dbl)
                            n222 = local read "CurrentOut"() -> (w595:dbl)
                            n223 = property class="DigNum (strict)"(reference=w600) -> ("Value"=w599:dbl)  [unwired: 1 in, 2 out]
                            n224 = Subtract(x=w614, y=w613) -> (x-y=w592:dbl)
                            n225 = Greater Or Equal?(x=w592, y=60.0) -> (x >= y?=w593:bool)
                            n226 = To Double Precision Float(number=w595) -> (double precision float=→"FullSpeed1 Current":dbl)
                            n227 = Greater Or Equal?(x=w595, y=w615) -> (x >= y?=w602:bool)
                            n228 = Greater Or Equal?(x=w592, y=15.0) -> (x >= y?=w590:bool)
                            n229 = Greater Or Equal?(x=w599, y=10600.0) -> (x >= y?=w597:bool)
                            n230 = And(x=w597, y=w602) -> (x .and. y?=w601:bool)
                            n231 = call "Write panel message Kinetics (SubVI).vi"(4:"rpm"=w600, 5:"rpm"=TRUE ("rpm"), "PrintTime"=FALSE, "Stop"=w603, "Time to wait"=0.2, "Strin"=w609, "String in"=w604) -> ("error out"=w611:errorcluster, "Stopped"=w596:bool)  [unwired: 3 in]
                            n232 = call "Display Message to User6"("Enable"=w590) -> ()  [unwired: 9 in, 2 out]
                            n233 = Compound Arithmetic op=OR(w590, w596, w593) -> (w594:bool)
                            n234 = Compound Arithmetic op=OR(w590, w596, w605, w593, w601) -> (w616:bool)
                          }
                          n235 = Select(t=T7."Stop", s=w562, f=T7."MD[1]=1") -> (s? t:f=w585:T7)
                        }
                        frame "MD[1]=0" {
                          n236 = call "Operation (SubVI).vi"("On/Off"=FALSE, "Operation"=T5."Venable", "DAQmx Device Name"=w622) -> ("error out"=w645:errorcluster)  [unwired: 8 in]
                          n237 = Concatenate Strings(w626, "\nSet Parameters MD[1]=0" ("Strin")) -> (w637:string)
                          n238 = call "Write panel message Kinetics (SubVI).vi"(4:"rpm"=w630, 5:"rpm"=FALSE ("rpm"), "PrintTime"=FALSE, "Stop"=w635, "error in (no error)"=w645, "Time to wait"=0.2, "Strin"=w637, "String in"=w636) -> ("error out"=w644:errorcluster, "Stopped"=w618:bool)  [unwired: 2 in]
                          n239 = call "Serial.vi"("error in (no error)"=w644, "write buffer"="EP=1\r\nVC=0\r\nMD[1]=0\r\n", "VISA resource name"=w627) -> ("error out"=w641:errorcluster)  [unwired: 7 in, 1 out]
                          n240 = call "Operation (SubVI).vi"("error in (no error)"=w641, "On/Off"=FALSE, "Operation"=T5."PowerSuply", "DAQmx Device Name"=w622) -> ("error out"=w640:errorcluster)  [unwired: 7 in]
                          n241 = call "Write panel message Kinetics (SubVI).vi"(4:"rpm"=w630, 5:"rpm"=FALSE ("rpm"), "PrintTime"=TRUE, "Stop"=w635, "error in (no error)"=w640, "Time to wait"=25.0, "Strin"=w637, "String in"=w636) -> ("error out"=w625:errorcluster, "Stopped"=w619:bool)  [unwired: 2 in]
                          n242 = call "Operation (SubVI).vi"("error in (no error)"=w625, "On/Off"=TRUE, "Operation"=T5."PowerSuply", "DAQmx Device Name"=w622) -> ("error out"=w624:errorcluster)  [unwired: 7 in]
                          n243 = call "Operation (SubVI).vi"("error in (no error)"=w624, "On/Off"=TRUE, "Operation"=T5."Venable", "DAQmx Device Name"=w622) -> ("error out"=w632:errorcluster)  [unwired: 7 in]
                          n244 = call "Write panel message Kinetics (SubVI).vi"(4:"rpm"=w630, 5:"rpm"=FALSE ("rpm"), "PrintTime"=TRUE, "Stop"=w635, "error in (no error)"=w632, "Time to wait"=3.0, "Strin"=w637, "String in"=w636) -> ("Stopped"=w620:bool)  [unwired: 2 in, 1 out]
                          n245 = Compound Arithmetic op=OR(w620, w619, w618) -> (w617:bool)
                          n246 = Compound Arithmetic op=OR(w620, w619, w618) -> (w629:bool)
                          n247 = Select(t=T7."Stop", s=w629, f=T7."FullSpeed1") -> (s? t:f=w658:T7)
                        }
                      }
                    }
                  }
                }
              }
            }
          }
        }
        frame "Venable Test" {
          n248 = control-ref of="Stop Button"() -> (w675:refnum<vi>)
          n249 = control-ref of="ATR"() -> (w676:refnum<vi>)
          n250 = control-ref of="Pannel User Message"() -> (w677:refnum<vi>)
          n251 = control-ref of="Motor Speed RPM Serial"() -> (w678:refnum<vi>)
          n252 = control-ref of="UUT"() -> (w679:refnum<vi>)
          n253 = Concatenate Strings(w671, " in process..." ("Strin")) -> (w672:string)
          n254 = while {
            shift-right: [w686] -> _
            shift-left: enum16{"Stop", "Direction", "Venable", "Start"}."Start" -> [w691]
            tunnel: w675 -> [w690]
            tunnel: w676 -> [w689]
            tunnel: w677 -> [w688]
            tunnel: w678 -> [w687]
            tunnel: w679 -> [w684]
            tunnel: w672 -> [w685]
            tunnel: w671 -> [w683]
            tunnel: w670 -> [w682]
            tunnel: [w680] -> w669
            stop <- w681 stop-if-true
            n255 = case shown="\"Start\"" w691 {
              tunnel: w690 -> [_ w721 w970 w1018]
              tunnel: w689 -> [_ w717 w968 w1011]
              tunnel: w688 -> [_ w720 w971 w1024]
              tunnel: w687 -> [_ w719 w972 _]
              tunnel: w684 -> [w692 w713 w973 _]
              tunnel: [w694 FALSE FALSE FALSE] -> w681
              tunnel: [w693 w716 w969 w1022] -> w686
              tunnel: w685 -> [_ w718 w967 w1017]
              tunnel: w683 -> [_ _ _ w1010]
              tunnel: w682 -> [_ _ _ w1013]
              tunnel: [_ _ _ w1005] -> w680
              frame "Stop", Default {
                n256 = disable-structure shown="Enabled" {
                  disable-tunnel: [w697 TRUE] -> w694
                  disable-tunnel: [w696 enum16{"Stop", "Direction", "Venable", "Start"}."Stop"] -> w693
                  disable-tunnel: w692 -> [w695 _]
                  frame Disabled {
                    n257 = flat-sequence {
                      tunnel: w695 -> [_]
                      tunnel: [TRUE] -> w697
                      tunnel: [enum16{"Stop", "Direction", "Venable", "Start"}."Stop"] -> w696
                      frame #0 {
                        (unwired) u16 0 ("Motor Speed RPM")
                        (unwired) TRUE ("Remote")
                        n258 = property on="VISA Kinetics" class="VISAName"() -> (error out=w701:errorcluster, "Value"=w702:refnum<visa-resource-name>)  [unwired: 2 in, 1 out]
                        n259 = call "Serial.vi"("error in (no error)"=w701, "Clear Log"=FALSE, "write buffer"="EP=1\r\nMD[1]=1\r\n", "VISA resource name"=w702) -> ("error out"=w698:errorcluster)  [unwired: 6 in, 1 out]
                        n260 = call "CANSendMessage.vi"("error in (no error)"=w698) -> ("error out"=w707:errorcluster)  [unwired: 10 in]
                        n261 = call "TesterOption (SubVI).vi"("2 Options"=FALSE, "error in (no error)"=w707, "On/Off"=FALSE, "Tester Option"=T8."Venable") -> ("error out"=w703:errorcluster)  [unwired: 6 in, 1 out]
                        n262 = call "Time Delay9"("error in (no error)"=w703) -> ()  [unwired: 10 in, 1 out]
                      }
                      frame #1 {
                      }
                    }
                  }
                  frame Enabled {
                  }
                }
              }
              frame "Direction" {
                n263 = property on="UUT" class="DigNum (strict)"() -> ("Value"=w712:u8)  [unwired: 2 in, 2 out]
                n264 = while {
                  shift-right: [w732] -> w715
                  shift-left: T7."MD[1]=0" -> [w733]
                  tunnel: w713 -> [w730]
                  tunnel: w721 -> [w729]
                  tunnel: w720 -> [w728]
                  tunnel: w719 -> [w727]
                  tunnel: w718 -> [w726]
                  tunnel: w717 -> [w725]
                  tunnel: w712 -> [w724]
                  stop <- w731 stop-if-true
                  n265 = case shown="\"FullSpeed2\"" w733 {
                    tunnel: [T7."Stop" w757 w794 w864 w892 w962] -> w732
                    tunnel: [TRUE FALSE FALSE FALSE FALSE FALSE] -> w731
                    tunnel: w730 -> [_ _ _ _ _ _]
                    tunnel: w729 -> [_ w744 w771 w834 w872 w930]
                    tunnel: w728 -> [_ _ w770 w843 w871 w940]
                    tunnel: w727 -> [_ _ w787 w832 w886 w936]
                    tunnel: w726 -> [_ _ w782 w851 w884 w948]
                    tunnel: w725 -> [_ w748 _ _ _ _]
                    tunnel: w724 -> [_ w736 w768 _ w866 _]
                    frame "Stop", Default {
                    }
                    frame "Result" {
                      n266 = property on="FullSpeed1 Current" class="DigNum (strict)"() -> ("Value"=w752:dbl)  [unwired: 2 in, 2 out]
                      n267 = property on="FullSpeed2 Current" class="DigNum (strict)"() -> ("Value"=w753:dbl)  [unwired: 2 in, 2 out]
                      n268 = property on="FullSpeed2 Speed" class="DigNum (strict)"() -> ("Value"=w755:dbl)  [unwired: 2 in, 2 out]
                      n269 = property on="FullSpeed1 Speed" class="DigNum (strict)"() -> ("Value"=w754:dbl)  [unwired: 2 in, 2 out]
                      n270 = Subtract(x=w753, y=w752) -> (x-y=w751:dbl)
                      n271 = Absolute Value(x=w751) -> (abs(x)=w740:dbl)
                      n272 = Greater Or Equal?(x=w740, y=u32 5) -> (x >= y?=w746:bool)
                      n273 = Equal?(x=w736, y=u8 95) -> (x = y?=w738:bool)
                      n274 = case shown="True" w738 {
                        tunnel: w755 -> [_ w766]
                        tunnel: w754 -> [_ w765]
                        tunnel: [TRUE w762] -> w747
                        frame False {
                        }
                        frame True {
                          n275 = Subtract(x=w766, y=w765) -> (x-y=w767:dbl)
                          n276 = Absolute Value(x=w767) -> (abs(x)=w764:dbl)
                          n277 = Greater Or Equal?(x=w764, y=500.0) -> (x >= y?=w762:bool)
                        }
                      }
                      n278 = call "Find_Number_LineMARVIN.vi"("Test Paragraph"="Motor Rotation Direction", "TableIn"=w748) -> ("Line number"=w745:i32)  [unwired: 3 in, 3 out]
                      n279 = And(x=w747, y=w746) -> (x .and. y?=w737:bool)
                      "VenableDirectionResult" <- w737
                      n280 = call "PassOrFail (SubVI).vi"("String Res"="", "index (row)"=w745, "Data in"=-3.0, "Pass?Fail"=w737, "Table in"=w748) -> ("error out"=w743:errorcluster)  [unwired: 6 in]
                      n281 = property class="Bool (strict)"(reference=w744, error in=w743) -> ("Value"=w760:bool)  [unwired: 2 out]
                      n282 = Select(t=T7."Stop", s=w760, f=T7."Stop") -> (s? t:f=w757:T7)
                    }
                    frame "FullSpeed2" {
                      (unwired) TRUE ("Remote")
                      n283 = Concatenate Strings(w782, "\nFull speed operation " ("string")) -> (w769:string)
                      n284 = call "CANSendMessage.vi"() -> ("error out"=w789:errorcluster)  [unwired: 11 in]
                      n285 = call "Write panel message Kinetics (SubVI).vi"(4:"rpm"=w787, 5:"rpm"=TRUE ("rpm"), "PrintTime"=FALSE, "Stop"=w771, "error in (no error)"=w789, "Time to wait"=0.2, "Strin"=w769, "String in"=w770) -> ("error out"=w774:errorcluster)  [unwired: 2 in, 1 out]
                      n286 = Equal?(x=w768, y=u8 95) -> (x = y?=w777:bool)
                      n287 = Select(t=u16 15100, s=w777, f=u16 12100 ("y")) -> ()  [unwired: 1 out]
                      n288 = flat-sequence {
                        tunnel: w774 -> [w799]
                        tunnel: [w799] -> w773
                        tunnel: [w798] -> w772
                        frame #0 {
                          n289 = call <vilib>:"High Resolution Relative Seconds.vi"() -> ("relative seconds"=w798:dbl)
                        }
                      }
                      n290 = Select(t=14500.0, s=w777, f=11500.0) -> (s? t:f=w776:dbl)
                      n291 = Select(t=47.0, s=w777, f=24.0) -> (s? t:f=w775:dbl)
                      n292 = while {
                        tunnel: w787 -> [w801]
                        tunnel: w773 -> [w825]
                        tunnel: [w808] -> w784
                        tunnel: w776 -> [w821]
                        tunnel: w775 -> [w820]
                        tunnel: w772 -> [w816]
                        tunnel: w771 -> [w806]
                        tunnel: w770 -> [w807]
                        tunnel: w769 -> [w804]
                        stop <- w818 stop-if-true
                        n293 = call <vilib>:"High Resolution Relative Seconds.vi"() -> ("relative seconds"=w817:dbl)
                        n294 = Subtract(x=w817, y=w816) -> (x-y=w815:dbl)
                        n295 = property class="DigNum (strict)"(reference=w801, error in=w825) -> ("Value"=w822:dbl)  [unwired: 2 out]
                        "FullSpeed2 Speed" <- w822
                        n296 = Greater Or Equal?(x=w815, y=120.0) -> (x >= y?=w813:bool)
                        n297 = Greater Or Equal?(x=w822, y=w821) -> (x >= y?=w812:bool)
                        n298 = property class="Bool (strict)"(reference=w806) -> ("Value"=w811:bool)  [unwired: 1 in, 2 out]
                        n299 = call "GetADCTester (SubVI).vi"("GetADCTester"=T9."Current", "TimeToGet"=5) -> ("error out"=w823:errorcluster, "ADCValOutput Single"=w819:dbl)  [unwired: 7 in, 1 out]
                        "FullSpeed2 Current" <- w819
                        n300 = Greater Or Equal?(x=w819, y=w820) -> (x >= y?=w809:bool)
                        n301 = And(x=w812, y=w809) -> (x .and. y?=w810:bool)
                        n302 = Compound Arithmetic op=OR(w811, w813, w810) -> (w818:bool)
                        n303 = call "Write panel message Kinetics (SubVI).vi"(4:"rpm"=w801, 5:"rpm"=TRUE ("rpm"), "PrintTime"=FALSE, "Stop"=w806, "error in (no error)"=w823, "Time to wait"=0.2, "Strin"=w804, "String in"=w807) -> ("error out"=w808:errorcluster)  [unwired: 2 in, 1 out]
                      }
                      n304 = property class="Bool (strict)"(reference=w771, error in=w784) -> ("Value"=w797:bool)  [unwired: 2 out]
                      n305 = Select(t=T7."Stop", s=w797, f=T7."Result") -> (s? t:f=w794:T7)
                    }
                    frame "MD[1]=1" {
                      (unwired) TRUE ("Remote")
                      (unwired) u16 0 ("Motor Speed RPM")
                      n306 = Concatenate Strings(w851, "\nSet Parameters MD[1]=1" ("Strin")) -> (w842:string)
                      n307 = call "TesterOption (SubVI).vi"("2 Options"=FALSE, "On/Off"=FALSE, "Tester Option"=T8."Venable") -> ("error out"=w856:errorcluster, "VISA Refnum out"=w847:refnum<visa-resource-name>)  [unwired: 7 in]
                      n308 = call "CANSendMessage.vi"("error in (no error)"=w856) -> ("error out"=w858:errorcluster)  [unwired: 10 in]
                      n309 = call "Write panel message Kinetics (SubVI).vi"(4:"rpm"=w832, 5:"rpm"=FALSE ("rpm"), "PrintTime"=TRUE, "Stop"=w834, "error in (no error)"=w858, "Time to wait"=20.0, "Strin"=w842, "String in"=w843) -> ("error out"=w831:errorcluster)  [unwired: 2 in, 1 out]
                      n310 = property on="VISA Kinetics" class="VISAName"(error in=w831) -> (error out=w857:errorcluster, "Value"=w860:refnum<visa-resource-name>)  [unwired: 1 in, 1 out]
                      n311 = call "Serial.vi"("error in (no error)"=w857, "Clear Log"=FALSE, "write buffer"="EP=1\r\nMD[1]=1\r\n", "VISA resource name"=w860) -> ("error out"=w846:errorcluster)  [unwired: 6 in, 1 out]
                      n312 = call "TesterOption (SubVI).vi"("2 Options"=FALSE, "error in (no error)"=w846, "On/Off"=FALSE, "Tester Option"=T8."Power", "VISA Refnum in"=w847) -> ("error out"=w844:errorcluster, "VISA Refnum out"=w835:refnum<visa-resource-name>)  [unwired: 5 in]
                      n313 = call "Write panel message Kinetics (SubVI).vi"(4:"rpm"=w832, 5:"rpm"=FALSE ("rpm"), "PrintTime"=TRUE, "Stop"=w834, "error in (no error)"=w844, "Time to wait"=25.0, "Strin"=w842, "String in"=w843) -> ("error out"=w836:errorcluster)  [unwired: 2 in, 1 out]
                      n314 = call "TesterOption (SubVI).vi"("2 Options"=FALSE, "error in (no error)"=w836, "On/Off"=TRUE, "Tester Option"=T8."Venable", "VISA Refnum in"=w835) -> ("error out"=w833:errorcluster)  [unwired: 5 in, 1 out]
                      n315 = call "Time Delay8"("error in (no error)"=w833) -> ("error out"=w829:errorcluster)  [unwired: 10 in]
                      n316 = property class="Bool (strict)"(reference=w834, error in=w829) -> ("Value"=w865:bool)  [unwired: 2 out]
                      n317 = Select(t=T7."Stop", s=w865, f=T7."FullSpeed2") -> (s? t:f=w864:T7)
                    }
                    frame "FullSpeed1" {
                      (unwired) TRUE ("Remote")
                      n318 = call "CANSendMessage.vi"() -> ("error out"=w887:errorcluster)  [unwired: 11 in]
                      n319 = Concatenate Strings(w884, "\nFull speed operation " ("string")) -> (w870:string)
                      n320 = call "Write panel message Kinetics (SubVI).vi"(4:"rpm"=w886, 5:"rpm"=TRUE ("rpm"), "PrintTime"=FALSE, "Stop"=w872, "error in (no error)"=w887, "Time to wait"=0.2, "Strin"=w870, "String in"=w871) -> ("error out"=w875:errorcluster)  [unwired: 2 in, 1 out]
                      n321 = Equal?(x=w866, y=u8 95) -> (x = y?=w882:bool)
                      n322 = flat-sequence {
                        tunnel: w875 -> [w897]
                        tunnel: [w897] -> w874
                        tunnel: [w896] -> w873
                        frame #0 {
                          n323 = call <vilib>:"High Resolution Relative Seconds.vi"() -> ("relative seconds"=w896:dbl)
                        }
                      }
                      n324 = Select(t=u16 15100, s=w882, f=u16 12100 ("y")) -> ()  [unwired: 1 out]
                      n325 = Select(t=13700.0, s=w882, f=11500.0) -> (s? t:f=w877:dbl)
                      n326 = Select(t=56.0, s=w882, f=33.0) -> (s? t:f=w876:dbl)
                      n327 = while {
                        tunnel: w886 -> [w899]
                        tunnel: w874 -> [w923]
                        tunnel: [w906] -> w885
                        tunnel: w877 -> [w918]
                        tunnel: w876 -> [w915]
                        tunnel: w873 -> [w913]
                        tunnel: w872 -> [w904]
                        tunnel: w871 -> [w905]
                        tunnel: w870 -> [w902]
                        stop <- w920 stop-if-true
                        n328 = property class="DigNum (strict)"(reference=w899, error in=w923) -> ("Value"=w919:dbl)  [unwired: 2 out]
                        "FullSpeed1 Speed" <- w919
                        n329 = call <vilib>:"High Resolution Relative Seconds.vi"() -> ("relative seconds"=w914:dbl)
                        n330 = Subtract(x=w914, y=w913) -> (x-y=w912:dbl)
                        n331 = Greater Or Equal?(x=w912, y=120.0) -> (x >= y?=w910:bool)
                        n332 = Greater Or Equal?(x=w919, y=w918) -> (x >= y?=w917:bool)
                        n333 = call "GetADCTester (SubVI).vi"("GetADCTester"=T9."Current", "TimeToGet"=5) -> ("error out"=w921:errorcluster, "ADCValOutput Single"=w916:dbl)  [unwired: 7 in, 1 out]
                        "FullSpeed1 Current" <- w916
                        n334 = Greater Or Equal?(x=w916, y=w915) -> (x >= y?=w907:bool)
                        n335 = And(x=w907, y=w917) -> (x .and. y?=w908:bool)
                        n336 = property class="Bool (strict)"(reference=w904) -> ("Value"=w909:bool)  [unwired: 1 in, 2 out]
                        n337 = call "Write panel message Kinetics (SubVI).vi"(4:"rpm"=w899, 5:"rpm"=TRUE ("rpm"), "PrintTime"=FALSE, "Stop"=w904, "error in (no error)"=w921, "Time to wait"=0.2, "Strin"=w902, "String in"=w905) -> ("error out"=w906:errorcluster)  [unwired: 2 in, 1 out]
                        n338 = Compound Arithmetic op=OR(w909, w908, w910) -> (w920:bool)
                      }
                      n339 = property class="Bool (strict)"(reference=w872, error in=w885) -> ("Value"=w895:bool)  [unwired: 2 out]
                      n340 = Select(t=T7."Stop", s=w895, f=T7."MD[1]=1") -> (s? t:f=w892:T7)
                    }
                    frame "MD[1]=0" {
                      (unwired) TRUE ("Remote")
                      (unwired) u16 0 ("Motor Speed RPM")
                      n341 = Concatenate Strings(w948, "\nSet Parameters MD[1]=0" ("Strin")) -> (w939:string)
                      n342 = call "TesterOption (SubVI).vi"("2 Options"=FALSE, "On/Off"=FALSE, "Tester Option"=T8."Venable") -> ("error out"=w954:errorcluster, "VISA Refnum out"=w944:refnum<visa-resource-name>)  [unwired: 7 in]
                      n343 = call "CANSendMessage.vi"("error in (no error)"=w954) -> ("error out"=w956:errorcluster)  [unwired: 10 in]
                      n344 = call "Write panel message Kinetics (SubVI).vi"(4:"rpm"=w936, 5:"rpm"=FALSE ("rpm"), "PrintTime"=FALSE, "Stop"=w930, "error in (no error)"=w956, "Time to wait"=0.2, "Strin"=w939, "String in"=w940) -> ("error out"=w951:errorcluster)  [unwired: 2 in, 1 out]
                      n345 = property on="VISA Kinetics" class="VISAName"(error in=w951) -> (error out=w955:errorcluster, "Value"=w958:refnum<visa-resource-name>)  [unwired: 1 in, 1 out]
                      n346 = call "Serial.vi"("error in (no error)"=w955, "Clear Log"=FALSE, "write buffer"="EP=1\r\nMD[1]=0\r\n", "VISA resource name"=w958) -> ("error out"=w943:errorcluster)  [unwired: 6 in, 1 out]
                      n347 = call "TesterOption (SubVI).vi"("2 Options"=FALSE, "error in (no error)"=w943, "On/Off"=FALSE, "Tester Option"=T8."Power", "VISA Refnum in"=w944) -> ("error out"=w941:errorcluster, "VISA Refnum out"=w931:refnum<visa-resource-name>)  [unwired: 5 in]
                      n348 = call "Write panel message Kinetics (SubVI).vi"(4:"rpm"=w936, 5:"rpm"=FALSE ("rpm"), "PrintTime"=TRUE, "Stop"=w930, "error in (no error)"=w941, "Time to wait"=25.0, "Strin"=w939, "String in"=w940) -> ("error out"=w932:errorcluster)  [unwired: 2 in, 1 out]
                      n349 = call "TesterOption (SubVI).vi"("2 Options"=FALSE, "error in (no error)"=w932, "On/Off"=TRUE, "Tester Option"=T8."Venable", "VISA Refnum in"=w931) -> ("error out"=w929:errorcluster)  [unwired: 5 in, 1 out]
                      n350 = call "Time Delay4"("error in (no error)"=w929) -> ("error out"=w925:errorcluster)  [unwired: 10 in]
                      n351 = property class="Bool (strict)"(reference=w930, error in=w925) -> ("Value"=w963:bool)  [unwired: 2 out]
                      n352 = Select(t=T7."Stop", s=w963, f=T7."FullSpeed1") -> (s? t:f=w962:T7)
                    }
                  }
                }
                n353 = flat-sequence {
                  tunnel: [enum16{"Stop", "Direction", "Venable", "Start"}."Stop"] -> w716
                  tunnel: w715 -> [_]
                  frame #0 {
                  }
                }
              }
              frame "Venable" {
                n354 = call "Find_Number_LineMARVIN.vi"("Test Paragraph"="Enable Test", "TableIn"=w968) -> ("Line number"=w974:i32)  [unwired: 3 in, 3 out]
                n355 = Increment(x=w974) -> (x+1=w964:i32)
                n356 = for {
                  tunnel: u16[] [5000, 0, 5000] -> [w999] mode=indexing
                  tunnel: bool[] [TRUE, FALSE, TRUE] -> [w997] mode=indexing
                  tunnel: w964 -> [w1000]
                  tunnel: w973 -> [_]
                  tunnel: w972 -> [w990]
                  tunnel: w971 -> [w993]
                  tunnel: w970 -> [w992]
                  tunnel: w968 -> [w986]
                  tunnel: w967 -> [w984]
                  tunnel: [w983] -> w966 mode=indexing
                  i -> [w1001]
                  (unwired) u16 5000 ("Motor Speed RPM")
                  (unwired) TRUE ("Remote")
                  w1002 = 200.0 ("y")
                  n357 = call "CANSendMessage.vi"() -> ("error out"=w996:errorcluster)  [unwired: 11 in]
                  n358 = Add(x=w1000, y=w1001) -> (x+y=w987:i32)
                  n359 = call "TesterOption (SubVI).vi"("2 Options"=FALSE, "error in (no error)"=w996, "On/Off"=w997, "Tester Option"=T8."Venable") -> ("error out"=w995:errorcluster)  [unwired: 6 in, 1 out]
                  n360 = call "Write panel message Kinetics (SubVI).vi"(4:"rpm"=w990, 5:"rpm"=TRUE ("rpm"), "PrintTime"=TRUE, "Stop"=w992, "error in (no error)"=w995, "Time to wait"=15.0, "Strin"=w984, "String in"=w993) -> ("error out"=w994:errorcluster)  [unwired: 2 in, 1 out]
                  n361 = property class="DigNum (strict)"(reference=w990, error in=w994) -> ("Value"=w985:dbl)  [unwired: 2 out]
                  n362 = Add(x=w999, y=w1002) -> (x+y=w1004:dbl)
                  n363 = Subtract(x=w999, y=w1002) -> (x-y=w1003:dbl)
                  n364 = In Range and Coerce(upper limit=w1004, x=w985, lower limit=w1003) -> (In Range?=w983:bool)  [unwired: 1 out]
                  n365 = call "PassOrFail (SubVI).vi"("index (row)"=w987, "Data in"=w985, "Pass?Fail"=w983, "Table in"=w986) -> ()  [unwired: 7 in, 1 out]
                }
                n366 = property class="Bool (strict)"(reference=w970) -> ("Value"=w981:bool)  [unwired: 1 in, 2 out]
                n367 = And Array Elements(Boolean array=w966) -> (logical AND=→"VenableResult":bool)
                n368 = Select(t=enum16{"Stop", "Direction", "Venable", "Start"}."Stop", s=w981, f=enum16{"Stop", "Direction", "Venable", "Start"}."Direction") -> (s? t:f=w969:enum16{"Stop", "Direction", "Venable", "Start"})
              }
              frame "Start" {
                n369 = property class="Str"(reference=w1024, "Value"=w1017) -> (error out=w1021:errorcluster)  [unwired: 1 in, 1 out]
                n370 = call "Find_Number_LineMARVIN.vi"("Test Paragraph"=w1010, "error in"=w1021, "TableIn"=w1011) -> ("error out"=w1012:errorcluster, "Line number"=w1009:i32)  [unwired: 2 in, 2 out]
                n371 = call "Table_ScrollaBarMarvin.vi"("error in"=w1012, "Line to focus"=w1010, "reference in"=w1011) -> ("error out"=w1025:errorcluster)  [unwired: 2 out]
                n372 = call "Reset old test Values (SubVI) Kinetics.vi"("error in"=w1025, "Atr in"=w1011, "Test Paragraph"=w1010) -> ("error out"=w1006:errorcluster)  [unwired: 6 in, 2 out]
                n373 = Increment(x=w1009) -> (x+1=w1008:i32)
                n374 = while {
                  shift-right: [w1037] -> _
                  shift-left: T6."VC=1000" -> [w1040]
                  tunnel: w1006 -> [w1039]
                  tunnel: w1013 -> [w1038]
                  tunnel: w1010 -> [w1036]
                  shift-right: [w1033] -> w1016
                  shift-left: bool[] [FALSE, FALSE] -> [w1034]
                  tunnel: w1008 -> [w1032]
                  tunnel: w1011 -> [w1031]
                  shift-right: [w1029] -> _
                  shift-left: dbl[] [0.0, 0.0] -> [w1030]
                  tunnel: [w1027] -> w1005
                  i -> [w1035]
                  stop <- w1028 stop-if-true
                  n375 = case shown="\"VC=1000\"" w1040 {
                    tunnel: w1039 -> [_ w1058 _ w1104 _]
                    tunnel: w1038 -> [_ w1057 w1073 w1108 _]
                    tunnel: [T6."Exit" T6."Wait" w1070 T6."Wait" T6."ReadVC"] -> w1037
                    tunnel: w1036 -> [_ _ _ _ w1115]
                    tunnel: [TRUE FALSE FALSE FALSE w1110] -> w1028
                    tunnel: w1035 -> [_ _ w1071 _ _]
                    tunnel: w1034 -> [w1042 w1055 w1069 w1106 w1112]
                    tunnel: [w1042 w1055 w1068 w1106 w1112] -> w1033
                    tunnel: w1032 -> [w1043 _ _ _ _]
                    tunnel: w1031 -> [w1044 _ _ _ _]
                    tunnel: w1030 -> [w1041 w1053 w1066 w1099 w1111]
                    tunnel: [w1041 w1053 w1065 w1099 w1111] -> w1029
                    tunnel: [_ _ _ _ w1110] -> w1027
                    frame "Exit", Default {
                      n376 = for {
                        tunnel: w1044 -> [w1052]
                        tunnel: w1043 -> [w1051]
                        tunnel: w1042 -> [w1050] mode=indexing
                        tunnel: w1041 -> [w1047] mode=indexing
                        i -> [w1048]
                        n377 = Add(x=w1048, y=w1051) -> (x+y=w1049:i32)
                        n378 = call "PassOrFail (SubVI).vi"("index (row)"=w1049, "Data in"=w1047, "Pass?Fail"=w1050, "Table in"=w1052) -> ()  [unwired: 7 in, 1 out]
                      }
                    }
                    frame "VC=0" {
                      n379 = disable-structure shown="Enabled" {
                        disable-tunnel: w1058 -> [w1061 _]
                        disable-tunnel: w1057 -> [w1059 _]
                        frame Disabled {
                          n380 = call "Serial.vi"("error in (no error)"=w1061, "write buffer"="EP=1\r\nVC=0\r\n", "VISA resource name"=w1059) -> ()  [unwired: 7 in, 2 out]
                        }
                        frame Enabled {
                          n381 = local read "DAQmx Device Name"() -> (w1064:tag)
                          n382 = call "Operation (SubVI).vi"("On/Off"=FALSE, "Operation"=T5."Venable", "DAQmx Device Name"=w1064) -> ()  [unwired: 8 in, 1 out]
                        }
                      }
                    }
                    frame "ReadVC" {
                      n383 = call "Serial.vi"("write buffer"="VC\r\n", "VISA resource name"=w1073) -> ("read buffer"=w1072:string)  [unwired: 8 in, 1 out]
                      n384 = case shown="2" w1071 {
                        tunnel: w1072 -> [w1085 w1095]
                        tunnel: [T6."VC=0" T6."Exit"] -> w1070
                        tunnel: w1069 -> [w1081 w1094]
                        tunnel: [w1079 w1091] -> w1068
                        tunnel: w1066 -> [w1078 w1090]
                        tunnel: [w1075 w1087] -> w1065
                        frame 2 {
                          n385 = Decimal String To Number(string=w1085) -> (number=w1076:i32)  [unwired: 2 in, 1 out]
                          n386 = In Range and Coerce(upper limit=1100, x=w1076, lower limit=900) -> (In Range?=w1080:bool)  [unwired: 1 out]
                          n387 = Replace Array Subset(array=w1078, new element=w1076, index=0) -> (w1075:dbl[])
                          n388 = Replace Array Subset(array=w1081, new element=w1080, index=0) -> (w1079:bool[])
                        }
                        frame 5, Default {
                          n389 = Decimal String To Number(string=w1095) -> (number=w1088:i32)  [unwired: 2 in, 1 out]
                          n390 = In Range and Coerce(upper limit=100, x=w1088, lower limit=0) -> (In Range?=w1092:bool)  [unwired: 1 out]
                          n391 = Replace Array Subset(array=w1090, new element=w1088, index=1) -> (w1087:dbl[])
                          n392 = Replace Array Subset(array=w1094, new element=w1092, index=1) -> (w1091:bool[])
                        }
                      }
                    }
                    frame "VC=1000" {
                      n393 = local read "DAQmx Device Name"() -> (w1105:tag)
                      n394 = call "Operation (SubVI).vi"("error in (no error)"=w1104, "On/Off"=TRUE, "Operation"=T5."Venable", "DAQmx Device Name"=w1105) -> ("error out"=w1103:errorcluster)  [unwired: 7 in]
                      n395 = call "Serial.vi"("error in (no error)"=w1103, "write buffer"="EP=1\r\nVC=1000\r\n", "VISA resource name"=w1108) -> ()  [unwired: 7 in, 2 out]
                    }
                    frame "Wait" {
                      n396 = control-ref of="Motor Speed RPM Serial"() -> (w1120:refnum<vi>)
                      n397 = control-ref of="Pannel User Message"() -> (w1119:refnum<vi>)
                      n398 = control-ref of="Stop Button"() -> (w1114:refnum<vi>)
                      n399 = call "Write panel message Kinetics (SubVI).vi"(4:"rpm"=w1120, 5:"rpm"=TRUE ("rpm"), "PrintTime"=TRUE, "Stop"=w1114, "Time to wait"=20.0, "Strin"=w1115, "String in"=w1119) -> ("Stopped"=w1110:bool)  [unwired: 3 in, 1 out]
                    }
                  }
                }
                n400 = And Array Elements(Boolean array=w1016) -> ()  [unwired: 1 out]
                n401 = property class="Bool (strict)"(reference=w1018) -> ("Value"=w1026:bool)  [unwired: 1 in, 2 out]
                n402 = Select(t=enum16{"Stop", "Direction", "Venable", "Start"}."Stop", s=w1026, f=enum16{"Stop", "Direction", "Venable", "Start"}."Stop") -> (s? t:f=w1022:enum16{"Stop", "Direction", "Venable", "Start"})
              }
            }
          }
        }
        frame "Motor Thermistor Test" {
          n403 = Concatenate Strings(w1132, " in process..." ("Strin")) -> (w1133:string)
          n404 = control-ref of="ATR"() -> (w1135:refnum<vi>)
          n405 = control-ref of="Pannel User Message"() -> (w1136:refnum<vi>)
          n406 = property class="Str"(reference=w1136, "Value"=w1133) -> (error out=w1129:errorcluster)  [unwired: 1 in, 1 out]
          n407 = call "Find_Number_LineMARVIN.vi"("Test Paragraph"=w1132, "error in"=w1129, "TableIn"=w1135) -> ("error out"=w1126:errorcluster, "Line number"=w1125:i32)  [unwired: 2 in, 2 out]
          n408 = call "Table_ScrollaBarMarvin.vi"("error in"=w1126, "Line to focus"=w1132, "reference in"=w1135) -> ("error out"=w1130:errorcluster)  [unwired: 2 out]
          n409 = call "Reset old test Values (SubVI) Kinetics.vi"("error in"=w1130, "Atr in"=w1135, "Test Paragraph"=w1132) -> ("error out"=w1122:errorcluster)  [unwired: 6 in, 2 out]
          n410 = Increment(x=w1125) -> (x+1=w1124:i32)
          n411 = while {
            shift-right: [w1147] -> _
            shift-left: T6."VC=1000" -> [w1150]
            tunnel: w1122 -> [w1149]
            tunnel: w1131 -> [w1148]
            tunnel: w1132 -> [w1146]
            shift-right: [w1142] -> _
            shift-left: bool[] [FALSE, FALSE] -> [w1143]
            tunnel: w1124 -> [w1141]
            tunnel: w1135 -> [w1140]
            shift-right: [w1138] -> _
            shift-left: dbl[] [0.0, 0.0] -> [w1139]
            tunnel: [w1137] -> w1121
            i -> [w1144]
            stop <- w1145 stop-if-true
            n412 = case shown="\"Wait\"" w1150 {
              tunnel: w1149 -> [_ w1174 _ w1231 _]
              tunnel: w1148 -> [w1151 w1173 w1190 w1235 _]
              tunnel: [T6."Exit" T6."Wait" w1187 T6."Wait" T6."ReadVC"] -> w1147
              tunnel: w1146 -> [_ _ _ _ w1242]
              tunnel: [TRUE FALSE FALSE FALSE w1237] -> w1145
              tunnel: w1144 -> [_ w1168 w1188 _ _]
              tunnel: w1143 -> [w1157 w1171 w1186 w1233 w1239]
              tunnel: [w1157 w1171 w1185 w1233 w1239] -> w1142
              tunnel: w1141 -> [w1158 _ _ _ _]
              tunnel: w1140 -> [w1159 _ _ _ _]
              tunnel: w1139 -> [w1156 w1169 w1183 w1226 w1238]
              tunnel: [w1156 w1169 w1182 w1226 w1238] -> w1138
              tunnel: [_ _ _ _ w1237] -> w1137
              frame "Exit", Default {
                n413 = for {
                  tunnel: w1159 -> [w1167]
                  tunnel: w1158 -> [w1166]
                  tunnel: w1157 -> [w1165] mode=indexing
                  tunnel: w1156 -> [w1162] mode=indexing
                  i -> [w1163]
                  n414 = Add(x=w1163, y=w1166) -> (x+y=w1164:i32)
                  n415 = call "PassOrFail (SubVI).vi"("index (row)"=w1164, "Data in"=w1162, "Pass?Fail"=w1165, "Table in"=w1167) -> ()  [unwired: 7 in, 1 out]
                }
                n416 = local read "DAQmx Device Name"() -> (w1155:tag)
                n417 = call "Serial.vi"("write buffer"="EP=1\r\nVC=0\r\n", "VISA resource name"=w1151) -> ()  [unwired: 8 in, 2 out]
                n418 = call "Operation (SubVI).vi"("On/Off"=FALSE, "Operation"=T5."Venable", "DAQmx Device Name"=w1155) -> ()  [unwired: 8 in, 1 out]
              }
              frame "VC=0" {
                n419 = disable-structure shown="Enabled" {
                  disable-tunnel: w1174 -> [w1177 _]
                  disable-tunnel: w1173 -> [w1175 _]
                  disable-tunnel: w1168 -> [_ w1178]
                  frame Disabled {
                    n420 = call "Serial.vi"("error in (no error)"=w1177, "write buffer"="EP=1\r\nVC=0\r\n", "VISA resource name"=w1175) -> ()  [unwired: 7 in, 2 out]
                  }
                  frame Enabled {
                    n421 = case shown="6, Default" w1178 {
                      tunnel: ["Connect wires of the thermistor" ("message") "Disconnect wires of the thermistor" ("message")] -> w1179
                      frame 6, Default {
                      }
                      frame 3 {
                      }
                    }
                    n422 = One Button Dialog(message=w1179) -> ()  [unwired: 1 in, 1 out]
                  }
                }
              }
              frame "ReadVC" {
                n423 = call "Serial.vi"("write buffer"="VC\r\n", "VISA resource name"=w1190) -> ("read buffer"=w1189:string)  [unwired: 8 in, 1 out]
                n424 = case shown="2" w1188 {
                  tunnel: w1189 -> [w1201 w1210 w1222]
                  tunnel: [w1195 T6."VC=0" T6."Exit"] -> w1187
                  tunnel: w1186 -> [w1192 w1209 w1221]
                  tunnel: [w1192 w1206 w1218] -> w1185
                  tunnel: w1183 -> [w1193 w1205 w1217]
                  tunnel: [w1193 w1202 w1214] -> w1182
                  frame 2 {
                    n425 = Decimal String To Number(string=w1201) -> (number=w1198:i32)  [unwired: 2 in, 1 out]
                    n426 = In Range and Coerce(upper limit=1100, x=w1198, lower limit=900) -> (In Range?=w1197:bool)  [unwired: 1 out]
                    n427 = Select(t=T6."VC=0", s=w1197, f=T6."Exit") -> (s? t:f=w1195:T6)
                  }
                  frame 5, Default {
                    n428 = Decimal String To Number(string=w1210) -> (number=w1203:i32)  [unwired: 2 in, 1 out]
                    n429 = In Range and Coerce(upper limit=100, x=w1203, lower limit=0) -> (In Range?=w1207:bool)  [unwired: 1 out]
                    n430 = Replace Array Subset(array=w1205, new element=w1203, index=0) -> (w1202:dbl[])
                    n431 = Replace Array Subset(array=w1209, new element=w1207, index=0) -> (w1206:bool[])
                  }
                  frame 8 {
                    n432 = Decimal String To Number(string=w1222) -> (number=w1215:i32)  [unwired: 2 in, 1 out]
                    n433 = In Range and Coerce(upper limit=1100, x=w1215, lower limit=900) -> (In Range?=w1219:bool)  [unwired: 1 out]
                    n434 = Replace Array Subset(array=w1217, new element=w1215, index=1) -> (w1214:dbl[])
                    n435 = Replace Array Subset(array=w1221, new element=w1219, index=1) -> (w1218:bool[])
                  }
                }
              }
              frame "VC=1000" {
                n436 = local read "DAQmx Device Name"() -> (w1232:tag)
                n437 = call "Operation (SubVI).vi"("error in (no error)"=w1231, "On/Off"=TRUE, "Operation"=T5."Venable", "DAQmx Device Name"=w1232) -> ("error out"=w1230:errorcluster)  [unwired: 7 in]
                n438 = call "Serial.vi"("error in (no error)"=w1230, "write buffer"="EP=1\r\nVC=1000\r\n", "VISA resource name"=w1235) -> ()  [unwired: 7 in, 2 out]
              }
              frame "Wait" {
                n439 = control-ref of="Motor Speed RPM Serial"() -> (w1247:refnum<vi>)
                n440 = control-ref of="Pannel User Message"() -> (w1246:refnum<vi>)
                n441 = control-ref of="Stop Button"() -> (w1241:refnum<vi>)
                n442 = call "Write panel message Kinetics (SubVI).vi"(4:"rpm"=w1247, 5:"rpm"=TRUE ("rpm"), "PrintTime"=TRUE, "Stop"=w1241, "Time to wait"=20.0, "Strin"=w1242, "String in"=w1246) -> ("Stopped"=w1237:bool)  [unwired: 3 in, 1 out]
              }
            }
          }
        }
        frame "Up/Down Blower Test" {
          n443 = control-ref of="Pannel User Message"() -> (w1279:refnum<vi>)
          n444 = Concatenate Strings(w1271, " in process..." ("Strin")) -> (w1250:string)
          n445 = property class="Str"(reference=w1279, error in=w1278, "Value"=w1250) -> (error out=w1277:errorcluster)  [unwired: 1 out]
          n446 = call "Table_ScrollaBarMarvin.vi"("error in"=w1277, "Line to focus"=w1271, "reference in"=w1265) -> ()  [unwired: 3 out]
          n447 = call "Reset old test Values (SubVI) Kinetics.vi"("Atr in"=w1265, "Test Paragraph"=w1271) -> ("error out"=w1272:errorcluster)  [unwired: 7 in, 2 out]
          n448 = call "Find_Number_LineMARVIN.vi"("Test Paragraph"=w1271, "error in"=w1272, "TableIn"=w1265) -> ("error out"=w1257:errorcluster, "Line number"=w1270:i32)  [unwired: 2 in, 2 out]
          n449 = control-ref of="Motor Speed RPM Serial"() -> (w1251:refnum<vi>)
          n450 = local read "DAQmx Device Name"() -> (w1258:tag)
          n451 = call "Operation (SubVI).vi"("error in (no error)"=w1257, "On/Off"=TRUE, "Operation"=T5."PowerSuply", "DAQmx Device Name"=w1258) -> ("error out"=w1249:errorcluster)  [unwired: 7 in]
          n452 = control-ref of="Pannel User Message"() -> (w1252:refnum<vi>)
          n453 = control-ref of="Stop Button"() -> (w1256:refnum<vi>)
          n454 = call "Write panel message Kinetics (SubVI).vi"(4:"rpm"=w1251, 5:"rpm"=FALSE ("rpm"), "PrintTime"=FALSE, "Stop"=w1256, "error in (no error)"=w1249, "Time to wait"=3.0, "Strin"=w1250, "String in"=w1252) -> ("error out"=w1248:errorcluster)  [unwired: 2 in, 1 out]
          n455 = Increment(x=w1270) -> (x+1=w1264:i32)
          n456 = call "Serial.vi"("error in (no error)"=w1248, "write buffer"="VM[1]\r\n", "VISA resource name"=w1268) -> ("error out"=w1267:errorcluster, "read buffer"=w1262:string)  [unwired: 7 in]
          n457 = call "InsertSingleData.vi"("String In"=w1262, "error in (no error)"=w1267, "Col"=2, "Row"=w1264, "Table in"=w1265) -> ("error out"=w1266:errorcluster)  [unwired: 6 in]
          n458 = while {
            shift-right: [w1291] -> _
            shift-left: T6."VC=1000" -> [w1294]
            tunnel: w1266 -> [w1293]
            tunnel: w1268 -> [w1292]
            tunnel: w1250 -> [w1290]
            shift-right: [w1287] -> _
            shift-left: bool[] [FALSE, FALSE] -> [w1288]
            tunnel: w1264 -> [w1286]
            tunnel: w1265 -> [w1285]
            shift-right: [w1283] -> _
            shift-left: dbl[] [0.0, 0.0] -> [w1284]
            tunnel: w1262 -> [w1282]
            tunnel: [w1280] -> w1261
            i -> [w1289]
            stop <- w1281 stop-if-true
            n459 = case shown="\"Wait\"" w1294 {
              tunnel: w1293 -> [_ w1315 _ w1375 _]
              tunnel: w1292 -> [_ w1314 w1331 w1378 _]
              tunnel: [T6."Exit" T6."Wait" w1328 T6."Wait" T6."ReadVC"] -> w1291
              tunnel: w1290 -> [_ _ _ _ w1385]
              tunnel: [TRUE FALSE FALSE FALSE w1380] -> w1281
              tunnel: w1289 -> [_ _ w1329 _ _]
              tunnel: w1288 -> [w1299 w1312 w1327 w1376 w1382]
              tunnel: [w1299 w1312 w1326 w1376 w1382] -> w1287
              tunnel: w1286 -> [w1300 _ _ _ _]
              tunnel: w1285 -> [w1301 _ _ _ _]
              tunnel: w1284 -> [w1298 w1310 w1324 w1370 w1381]
              tunnel: [w1298 w1310 w1323 w1370 w1381] -> w1283
              tunnel: w1282 -> [_ _ w1322 _ _]
              tunnel: [_ _ _ _ w1380] -> w1280
              frame "Exit", Default {
                n460 = for {
                  tunnel: w1301 -> [w1309]
                  tunnel: w1300 -> [w1308]
                  tunnel: w1299 -> [w1307] mode=indexing
                  tunnel: w1298 -> [w1304] mode=indexing
                  i -> [w1305]
                  n461 = Add(x=w1305, y=w1308) -> (x+y=w1306:i32)
                  n462 = call "PassOrFail (SubVI).vi"("index (row)"=w1306, "Data in"=w1304, "Pass?Fail"=w1307, "Table in"=w1309) -> ()  [unwired: 7 in, 1 out]
                }
                n463 = local read "DAQmx Device Name"() -> (w1297:tag)
                n464 = call "Operation (SubVI).vi"("On/Off"=FALSE, "Operation"=T5."Venable", "DAQmx Device Name"=w1297) -> ()  [unwired: 8 in, 1 out]
              }
              frame "VC=0" {
                n465 = disable-structure shown="Enabled" {
                  disable-tunnel: w1315 -> [w1318 _]
                  disable-tunnel: w1314 -> [w1316 _]
                  frame Disabled {
                    n466 = call "Serial.vi"("error in (no error)"=w1318, "write buffer"="EP=1\r\nVC=0\r\n", "VISA resource name"=w1316) -> ()  [unwired: 7 in, 2 out]
                  }
                  frame Enabled {
                    n467 = local read "DAQmx Device Name"() -> (w1321:tag)
                    n468 = call "Operation (SubVI).vi"("On/Off"=TRUE, "Operation"=T5."Down", "DAQmx Device Name"=w1321) -> ()  [unwired: 8 in, 1 out]
                  }
                }
              }
              frame "ReadVC" {
                n469 = call "Serial.vi"("write buffer"="VC\r\n", "VISA resource name"=w1331) -> ("read buffer"=w1330:string)  [unwired: 8 in, 1 out]
                n470 = case shown="5, Default" w1329 {
                  tunnel: w1330 -> [w1349 w1362]
                  tunnel: [T6."VC=0" T6."Exit"] -> w1328
                  tunnel: w1327 -> [w1347 w1361]
                  tunnel: [w1345 w1358] -> w1326
                  tunnel: w1324 -> [w1344 w1357]
                  tunnel: [w1342 w1354] -> w1323
                  tunnel: w1322 -> [w1336 _]
                  frame 2 {
                    w1337 = 100
                    n471 = Decimal String To Number(string=w1349) -> (number=w1338:i32)  [unwired: 2 in, 1 out]
                    n472 = Decimal String To Number(string=w1336) -> (number=w1333:i32)  [unwired: 2 in, 1 out]
                    n473 = Add(x=w1333, y=w1337) -> (x+y=w1335:i32)
                    n474 = Subtract(x=w1333, y=w1337) -> (x-y=w1334:i32)
                    n475 = In Range and Coerce(upper limit=w1335, x=w1338, lower limit=w1334) -> (In Range?=w1346:bool)  [unwired: 1 out]
                    n476 = Replace Array Subset(array=w1344, new element=w1338, index=0) -> (w1342:dbl[])
                    n477 = Replace Array Subset(array=w1347, new element=w1346, index=0) -> (w1345:bool[])
                    n478 = local read "DAQmx Device Name"() -> (w1341:tag)
                    n479 = call "Operation (SubVI).vi"("On/Off"=FALSE, "Operation"=T5."Up", "DAQmx Device Name"=w1341) -> ()  [unwired: 8 in, 1 out]
                  }
                  frame 5, Default {
                    n480 = Decimal String To Number(string=w1362) -> (number=w1355:i32)  [unwired: 2 in, 1 out]
                    n481 = In Range and Coerce(upper limit=100, x=w1355, lower limit=0) -> (In Range?=w1359:bool)  [unwired: 1 out]
                    n482 = Replace Array Subset(array=w1357, new element=w1355, index=1) -> (w1354:dbl[])
                    n483 = Replace Array Subset(array=w1361, new element=w1359, index=1) -> (w1358:bool[])
                    n484 = local read "DAQmx Device Name"() -> (w1353:tag)
                    n485 = call "Operation (SubVI).vi"("On/Off"=FALSE, "Operation"=T5."Down", "DAQmx Device Name"=w1353) -> ()  [unwired: 8 in, 1 out]
                  }
                }
              }
              frame "VC=1000" {
                n486 = local read "DAQmx Device Name"() -> (w1369:tag)
                n487 = call "Operation (SubVI).vi"("error in (no error)"=w1375, "On/Off"=TRUE, "Operation"=T5."Venable", "DAQmx Device Name"=w1369) -> ("error out"=w1374:errorcluster)  [unwired: 7 in]
                n488 = call "Serial.vi"("error in (no error)"=w1374, "write buffer"="EP=1\r\nVC=0\r\n", "VISA resource name"=w1378) -> ("error out"=w1366:errorcluster)  [unwired: 7 in, 1 out]
                n489 = call "Operation (SubVI).vi"("error in (no error)"=w1366, "On/Off"=TRUE, "Operation"=T5."Up", "DAQmx Device Name"=w1369) -> ()  [unwired: 7 in, 1 out]
              }
              frame "Wait" {
                n490 = control-ref of="Motor Speed RPM Serial"() -> (w1390:refnum<vi>)
                n491 = control-ref of="Pannel User Message"() -> (w1389:refnum<vi>)
                n492 = control-ref of="Stop Button"() -> (w1384:refnum<vi>)
                n493 = call "Write panel message Kinetics (SubVI).vi"(4:"rpm"=w1390, 5:"rpm"=TRUE ("rpm"), "PrintTime"=TRUE, "Stop"=w1384, "Time to wait"=30.0, "Strin"=w1385, "String in"=w1389) -> ("Stopped"=w1380:bool)  [unwired: 3 in, 1 out]
              }
            }
          }
        }
        frame "Resistance Merkava 4 Test" {
          w1399 = T12 [enum."0 ohm", enum."6 ohm", enum."15 ohm"] items=["Init", "0 ohm", "6 ohm", "13.2 ohm", "15 ohm", "25.9 ohm", "33 ohm", "Down", "Up", "Venable", "Firmware", "PowerSuply"]
          w1403 = T12 [enum."6 ohm", enum."15 ohm", enum."15 ohm"] items=["Init", "0 ohm", "6 ohm", "13.2 ohm", "15 ohm", "25.9 ohm", "33 ohm", "Down", "Up", "Venable", "Firmware", "PowerSuply"]
          w1408 = T12 [enum."PowerSuply", enum."Down"] items=["Init", "0 ohm", "6 ohm", "13.2 ohm", "15 ohm", "25.9 ohm", "33 ohm", "Down", "Up", "Venable", "Firmware", "PowerSuply"]
          w1409 = T12 [enum."PowerSuply", enum."Venable", enum."Down", enum."0 ohm", enum."PowerSuply"] items=["Init", "0 ohm", "6 ohm", "13.2 ohm", "15 ohm", "25.9 ohm", "33 ohm", "Down", "Up", "Venable", "Firmware", "PowerSuply"]
          w1416 = T12 [enum."0 ohm", enum."6 ohm", enum."15 ohm"] items=["Init", "0 ohm", "6 ohm", "13.2 ohm", "15 ohm", "25.9 ohm", "33 ohm", "Down", "Up", "Venable", "Firmware", "PowerSuply"]
          # "1.65"
          n494 = control-ref of="Pannel User Message"() -> (w1422:refnum<vi>)
          n495 = Concatenate Strings(w1418, " in process..." ("Strin")) -> (w1410:string)
          n496 = property class="Str"(reference=w1422, error in=w1417, "Value"=w1410) -> (error out=w1421:errorcluster)  [unwired: 1 out]
          n497 = call "Table_ScrollaBarMarvin.vi"("error in"=w1421, "Line to focus"=w1418, "reference in"=w1412) -> ()  [unwired: 3 out]
          n498 = call "Reset old test Values (SubVI) Kinetics.vi"("Atr in"=w1412, "Test Paragraph"=w1418) -> ("error out"=w1420:errorcluster)  [unwired: 7 in, 2 out]
          n499 = call "Find_Number_LineMARVIN.vi"("Test Paragraph"=w1418, "error in"=w1420, "TableIn"=w1412) -> ("error out"=w1393:errorcluster, "Line number"=w1414:i32)  [unwired: 2 in, 2 out]
          n500 = disable-structure shown="Enabled" {
            disable-tunnel: [w1425 "CF[0]=4.5"] -> w1395
            disable-tunnel: w1393 -> [w1424 w1427]
            disable-tunnel: [w1423 w1427] -> w1392
            frame Disabled {
              n501 = call "Cable Length Param.vi"("error constant"=w1424) -> ("error out"=w1423:errorcluster, "Cable Length Param"=w1425:string)  [unwired: 9 in]
            }
            frame Enabled {
            }
          }
          n502 = for {
            tunnel: w1409 -> [w1438] mode=indexing
            tunnel: [w1436] -> w1411
            tunnel: w1392 -> [w1437]
            tunnel: [w1433] -> w1391
            tunnel: bool[] [FALSE, TRUE, TRUE, TRUE, TRUE] -> [w1435] mode=indexing
            tunnel: dbl[] [5.0, 0.2, 0.2, 0.2, 3.0] -> [w1432] mode=indexing
            n503 = local read "DAQmx Device Name"() -> (w1436:tag)
            n504 = call "Operation (SubVI).vi"("error in (no error)"=w1437, "On/Off"=w1435, "Operation"=w1438, "DAQmx Device Name"=w1436) -> ("error out"=w1434:errorcluster)  [unwired: 7 in]
            n505 = call "Time Delay6"("error in (no error)"=w1434, "Delay Time (s)"=w1432) -> ("error out"=w1433:errorcluster)  [unwired: 9 in]
          }
          n506 = Concatenate Strings("EP=1\r\n" ("write buffer"), w1395, "\r\n" ("string")) -> (w1394:string)
          n507 = call "Serial.vi"("error in (no error)"=w1391, "write buffer"=w1394, "VISA resource name"=w1406) -> ("error out"=w1407:errorcluster)  [unwired: 7 in, 1 out]
          n508 = Increment(x=w1414) -> (x+1=w1413:i32)
          n509 = for {
            tunnel: w1416 -> [w1445] mode=indexing
            tunnel: i32[] [6850, 8300, 9200] -> [w1461] mode=indexing
            tunnel: w1413 -> [w1456]
            tunnel: w1412 -> [w1451]
            tunnel: w1407 -> [w1450]
            tunnel: w1411 -> [w1449]
            tunnel: w1410 -> [w1448]
            tunnel: bool[] [TRUE, TRUE, TRUE] -> [w1447] mode=indexing
            tunnel: w1403 -> [w1442] mode=indexing
            tunnel: [w1446] -> w1401
            tunnel: bool[] [TRUE, FALSE] -> [w1444]
            tunnel: w1399 -> [w1441] mode=indexing
            tunnel: [w1440] -> w1398
            i -> [w1457]
            stop <- w1446 stop-if-true
            w1460 = 100 ("x")
            n510 = Add(x=w1456, y=w1457) -> (x+y=w1455:i32)
            n511 = call "Operation (SubVI).vi"("error in (no error)"=w1450, "On/Off"=w1447, "Operation"=w1445, "DAQmx Device Name"=w1449) -> ("error out"=w1463:errorcluster)  [unwired: 7 in]
            n512 = control-ref of="Motor Speed RPM Serial"() -> (w1464:refnum<vi>)
            n513 = control-ref of="Pannel User Message"() -> (w1466:refnum<vi>)
            n514 = control-ref of="Stop Button"() -> (w1469:refnum<vi>)
            n515 = call "Write panel message Kinetics (SubVI).vi"(4:"rpm"=w1464, 5:"rpm"=TRUE ("rpm"), "PrintTime"=TRUE, "Stop"=w1469, "error in (no error)"=w1463, "Time to wait"=30.0, "Strin"=w1448, "String in"=w1466) -> ("error out"=w1462:errorcluster, "Stopped"=w1446:bool)  [unwired: 2 in]
            n516 = property on="Motor Speed RPM Serial" class="DigNum (strict)"(error in=w1462) -> (error out=w1454:errorcluster, "Value"=w1453:dbl)  [unwired: 1 in, 1 out]
            n517 = Subtract(x=w1461, y=w1460) -> (x-y=w1458:i32)
            n518 = Add(x=w1460, y=w1461) -> (x+y=w1459:i32)
            n519 = In Range and Coerce(upper limit=w1459, x=w1453, lower limit=w1458) -> (In Range?=w1452:bool)  [unwired: 1 out]
            n520 = call "PassOrFail (SubVI).vi"("index (row)"=w1455, "error in (no error)"=w1454, "Data in"=w1453, "Pass?Fail"=w1452, "Table in"=w1451) -> ("error out"=w1439:errorcluster)  [unwired: 6 in]
            n521 = Build Array(w1442, w1441) -> (w1443:T12)
            n522 = for {
              tunnel: w1449 -> [w1475]
              tunnel: w1444 -> [w1474] mode=indexing
              tunnel: w1443 -> [w1473] mode=indexing
              tunnel: [w1471] -> w1440
              tunnel: w1439 -> [w1470]
              n523 = call "Operation (SubVI).vi"("error in (no error)"=w1470, "On/Off"=w1474, "Operation"=w1473, "DAQmx Device Name"=w1475) -> ("error out"=w1472:errorcluster)  [unwired: 7 in]
              n524 = call "Time Delay5"("error in (no error)"=w1472) -> ("error out"=w1471:errorcluster)  [unwired: 10 in]
            }
          }
          n525 = for {
            tunnel: w1398 -> [w1429]
            tunnel: w1408 -> [w1428] mode=indexing
            n526 = local read "DAQmx Device Name"() -> (w1430:tag)
            n527 = call "Operation (SubVI).vi"("error in (no error)"=w1429, "On/Off"=FALSE, "Operation"=w1428, "DAQmx Device Name"=w1430) -> ()  [unwired: 7 in, 1 out]
          }
        }
        frame "Resistance Merkava 3 Test" {
          w1485 = T12 [enum."0 ohm", enum."13.2 ohm", enum."33 ohm"] items=["Init", "0 ohm", "6 ohm", "13.2 ohm", "15 ohm", "25.9 ohm", "33 ohm", "Down", "Up", "Venable", "Firmware", "PowerSuply"]
          w1489 = T12 [enum."13.2 ohm", enum."33 ohm", enum."33 ohm"] items=["Init", "0 ohm", "6 ohm", "13.2 ohm", "15 ohm", "25.9 ohm", "33 ohm", "Down", "Up", "Venable", "Firmware", "PowerSuply"]
          w1492 = T12 [enum."PowerSuply", enum."Venable", enum."Up", enum."0 ohm", enum."PowerSuply"] items=["Init", "0 ohm", "6 ohm", "13.2 ohm", "15 ohm", "25.9 ohm", "33 ohm", "Down", "Up", "Venable", "Firmware", "PowerSuply"]
          (unwired) "EP=1\r\nCF[0]=4.5\r\n" ("write buffer")
          w1495 = T12 [enum."PowerSuply", enum."Up"] items=["Init", "0 ohm", "6 ohm", "13.2 ohm", "15 ohm", "25.9 ohm", "33 ohm", "Down", "Up", "Venable", "Firmware", "PowerSuply"]
          w1501 = T12 [enum."0 ohm", enum."13.2 ohm", enum."33 ohm"] items=["Init", "0 ohm", "6 ohm", "13.2 ohm", "15 ohm", "25.9 ohm", "33 ohm", "Down", "Up", "Venable", "Firmware", "PowerSuply"]
          # "6.5"
          n528 = control-ref of="Pannel User Message"() -> (w1507:refnum<vi>)
          n529 = Concatenate Strings(w1503, " in process..." ("Strin")) -> (w1476:string)
          n530 = property class="Str"(reference=w1507, error in=w1502, "Value"=w1476) -> (error out=w1506:errorcluster)  [unwired: 1 out]
          n531 = call "Table_ScrollaBarMarvin.vi"("error in"=w1506, "Line to focus"=w1503, "reference in"=w1497) -> ()  [unwired: 3 out]
          n532 = call "Reset old test Values (SubVI) Kinetics.vi"("Atr in"=w1497, "Test Paragraph"=w1503) -> ("error out"=w1505:errorcluster)  [unwired: 7 in, 2 out]
          n533 = call "Find_Number_LineMARVIN.vi"("Test Paragraph"=w1503, "error in"=w1505, "TableIn"=w1497) -> ("error out"=w1478:errorcluster, "Line number"=w1499:i32)  [unwired: 2 in, 2 out]
          n534 = disable-structure shown="Enabled" {
            disable-tunnel: [w1510 "CF[0]=4.5"] -> w1482
            disable-tunnel: w1478 -> [w1509 w1512]
            disable-tunnel: [w1508 w1512] -> w1477
            frame Disabled {
              n535 = call "Cable Length Param.vi"("error constant"=w1509) -> ("error out"=w1508:errorcluster, "Cable Length Param"=w1510:string)  [unwired: 9 in]
            }
            frame Enabled {
            }
          }
          n536 = for {
            tunnel: [w1522] -> w1496
            tunnel: w1477 -> [w1523]
            tunnel: [w1518] -> w1479
            tunnel: w1492 -> [w1521] mode=indexing
            tunnel: bool[] [FALSE, TRUE, TRUE, TRUE, TRUE] -> [w1520] mode=indexing
            tunnel: dbl[] [10.0, 0.2, 0.2, 0.2, 3.0] -> [w1517] mode=indexing
            n537 = local read "DAQmx Device Name"() -> (w1522:tag)
            n538 = call "Operation (SubVI).vi"("error in (no error)"=w1523, "On/Off"=w1520, "Operation"=w1521, "DAQmx Device Name"=w1522) -> ("error out"=w1519:errorcluster)  [unwired: 7 in]
            n539 = call "Time Delay7"("error in (no error)"=w1519, "Delay Time (s)"=w1517) -> ("error out"=w1518:errorcluster)  [unwired: 9 in]
          }
          n540 = Concatenate Strings("EP=1\r\n" ("write buffer"), w1482, "\r\n" ("string")) -> (w1480:string)
          n541 = Increment(x=w1499) -> (x+1=w1498:i32)
          n542 = call "Serial.vi"("error in (no error)"=w1479, "write buffer"=w1480, "VISA resource name"=w1494) -> ("error out"=w1493:errorcluster)  [unwired: 7 in, 1 out]
          n543 = for {
            tunnel: w1501 -> [w1535] mode=indexing
            tunnel: i32[] [6850, 9000, 9980] -> [w1546] mode=indexing
            tunnel: w1498 -> [w1541]
            tunnel: w1497 -> [w1536]
            tunnel: w1493 -> [w1534]
            tunnel: w1496 -> [w1533]
            tunnel: w1476 -> [w1532]
            tunnel: bool[] [TRUE, TRUE, TRUE] -> [w1531] mode=indexing
            tunnel: w1489 -> [w1528] mode=indexing
            tunnel: [w1530] -> w1487
            tunnel: bool[] [TRUE, FALSE] -> [w1529]
            tunnel: w1485 -> [w1527] mode=indexing
            tunnel: [w1525] -> w1484
            i -> [w1542]
            stop <- w1530 stop-if-true
            w1545 = 100 ("x")
            n544 = Add(x=w1541, y=w1542) -> (x+y=w1540:i32)
            n545 = call "Operation (SubVI).vi"("error in (no error)"=w1534, "On/Off"=w1531, "Operation"=w1535, "DAQmx Device Name"=w1533) -> ("error out"=w1548:errorcluster)  [unwired: 7 in]
            n546 = control-ref of="Motor Speed RPM Serial"() -> (w1549:refnum<vi>)
            n547 = control-ref of="Pannel User Message"() -> (w1551:refnum<vi>)
            n548 = control-ref of="Stop Button"() -> (w1554:refnum<vi>)
            n549 = call "Write panel message Kinetics (SubVI).vi"(4:"rpm"=w1549, 5:"rpm"=TRUE ("rpm"), "PrintTime"=TRUE, "Stop"=w1554, "error in (no error)"=w1548, "Time to wait"=30.0, "Strin"=w1532, "String in"=w1551) -> ("error out"=w1547:errorcluster, "Stopped"=w1530:bool)  [unwired: 2 in]
            n550 = property on="Motor Speed RPM Serial" class="DigNum (strict)"(error in=w1547) -> (error out=w1539:errorcluster, "Value"=w1538:dbl)  [unwired: 1 in, 1 out]
            n551 = Subtract(x=w1546, y=w1545) -> (x-y=w1543:i32)
            n552 = Add(x=w1545, y=w1546) -> (x+y=w1544:i32)
            n553 = In Range and Coerce(upper limit=w1544, x=w1538, lower limit=w1543) -> (In Range?=w1537:bool)  [unwired: 1 out]
            n554 = Build Array(w1528, w1527) -> (w1526:T12)
            n555 = call "PassOrFail (SubVI).vi"("index (row)"=w1540, "error in (no error)"=w1539, "Data in"=w1538, "Pass?Fail"=w1537, "Table in"=w1536) -> ("error out"=w1524:errorcluster)  [unwired: 6 in]
            n556 = for {
              tunnel: w1533 -> [w1560]
              tunnel: w1529 -> [w1559] mode=indexing
              tunnel: w1526 -> [w1558] mode=indexing
              tunnel: [w1556] -> w1525
              tunnel: w1524 -> [w1555]
              n557 = call "Operation (SubVI).vi"("error in (no error)"=w1555, "On/Off"=w1559, "Operation"=w1558, "DAQmx Device Name"=w1560) -> ("error out"=w1557:errorcluster)  [unwired: 7 in]
              n558 = call "Time Delay2"("error in (no error)"=w1557) -> ("error out"=w1556:errorcluster)  [unwired: 10 in]
            }
          }
          n559 = for {
            tunnel: w1484 -> [w1514]
            tunnel: w1495 -> [w1513] mode=indexing
            n560 = local read "DAQmx Device Name"() -> (w1515:tag)
            n561 = call "Operation (SubVI).vi"("error in (no error)"=w1514, "On/Off"=FALSE, "Operation"=w1513, "DAQmx Device Name"=w1515) -> ()  [unwired: 7 in, 1 out]
          }
        }
        frame "Resistance Namer Test" {
          w1569 = T12 [enum."13.2 ohm", enum."25.9 ohm", enum."33 ohm"] items=["Init", "0 ohm", "6 ohm", "13.2 ohm", "15 ohm", "25.9 ohm", "33 ohm", "Down", "Up", "Venable", "Firmware", "PowerSuply"]
          w1570 = T12 [enum."25.9 ohm", enum."33 ohm", enum."33 ohm"] items=["Init", "0 ohm", "6 ohm", "13.2 ohm", "15 ohm", "25.9 ohm", "33 ohm", "Down", "Up", "Venable", "Firmware", "PowerSuply"]
          w1576 = T12 [enum."Init", enum."PowerSuply", enum."Venable", enum."Down", enum."Up", enum."13.2 ohm", enum."PowerSuply", enum."Down", enum."Up"] items=["Init", "0 ohm", "6 ohm", "13.2 ohm", "15 ohm", "25.9 ohm", "33 ohm", "Down", "Up", "Venable", "Firmware", "PowerSuply"]
          (unwired) "EP=1\r\nCF[0]=4.5\r\n" ("write buffer")
          w1579 = T12 [enum."Init", enum."Down", enum."Up"] items=["Init", "0 ohm", "6 ohm", "13.2 ohm", "15 ohm", "25.9 ohm", "33 ohm", "Down", "Up", "Venable", "Firmware", "PowerSuply"]
          w1585 = T12 [enum."13.2 ohm", enum."25.9 ohm", enum."33 ohm"] items=["Init", "0 ohm", "6 ohm", "13.2 ohm", "15 ohm", "25.9 ohm", "33 ohm", "Down", "Up", "Venable", "Firmware", "PowerSuply"]
          n562 = control-ref of="Pannel User Message"() -> (w1591:refnum<vi>)
          n563 = Concatenate Strings(w1587, " in process..." ("Strin")) -> (w1580:string)
          n564 = property class="Str"(reference=w1591, error in=w1586, "Value"=w1580) -> (error out=w1590:errorcluster)  [unwired: 1 out]
          n565 = call "Table_ScrollaBarMarvin.vi"("error in"=w1590, "Line to focus"=w1587, "reference in"=w1581) -> ()  [unwired: 3 out]
          n566 = call "Reset old test Values (SubVI) Kinetics.vi"("Atr in"=w1581, "Test Paragraph"=w1587) -> ("error out"=w1589:errorcluster)  [unwired: 7 in, 2 out]
          n567 = call "Find_Number_LineMARVIN.vi"("Test Paragraph"=w1587, "error in"=w1589, "TableIn"=w1581) -> ("error out"=w1562:errorcluster, "Line number"=w1583:i32)  [unwired: 2 in, 2 out]
          n568 = disable-structure shown="Enabled" {
            disable-tunnel: [w1594 "CF[0]=4.5"] -> w1567
            disable-tunnel: w1562 -> [w1593 w1596]
            disable-tunnel: [w1592 w1596] -> w1561
            frame Disabled {
              n569 = call "Cable Length Param.vi"("error constant"=w1593) -> ("error out"=w1592:errorcluster, "Cable Length Param"=w1594:string)  [unwired: 9 in]
            }
            frame Enabled {
            }
          }
          n570 = for {
            tunnel: [w1606] -> w1573
            tunnel: w1561 -> [w1607]
            tunnel: [w1603] -> w1563
            tunnel: w1576 -> [w1605] mode=indexing
            tunnel: dbl[] [1.0, 10.0, 0.2, 0.2, 0.2, 0.2, 5.0, 0.2, 0.2] -> [w1602] mode=indexing
            tunnel: bool[] [FALSE, FALSE, TRUE, TRUE, TRUE, TRUE, TRUE, TRUE, TRUE] -> [w1601] mode=indexing
            n571 = local read "DAQmx Device Name"() -> (w1606:tag)
            n572 = call "Operation (SubVI).vi"("error in (no error)"=w1607, "On/Off"=w1601, "Operation"=w1605, "DAQmx Device Name"=w1606) -> ("error out"=w1604:errorcluster)  [unwired: 7 in]
            n573 = call "Time Delay10"("error in (no error)"=w1604, "Delay Time (s)"=w1602) -> ("error out"=w1603:errorcluster)  [unwired: 9 in]
          }
          n574 = Concatenate Strings("EP=1\r\n" ("write buffer"), w1567, "\r\n" ("string")) -> (w1564:string)
          n575 = call "Serial.vi"("error in (no error)"=w1563, "write buffer"=w1564, "VISA resource name"=w1572) -> ("error out"=w1578:errorcluster)  [unwired: 7 in, 1 out]
          n576 = Increment(x=w1583) -> (x+1=w1582:i32)
          n577 = for {
            tunnel: w1585 -> [w1614] mode=indexing
            tunnel: i32[] [8350, 8900, 9450] -> [w1629] mode=indexing
            tunnel: w1582 -> [w1624]
            tunnel: w1581 -> [w1619]
            tunnel: w1578 -> [w1618]
            tunnel: w1573 -> [w1617]
            tunnel: w1580 -> [w1616]
            tunnel: [w1615] -> w1574
            tunnel: bool[] [TRUE, FALSE] -> [w1613]
            tunnel: w1570 -> [w1612] mode=indexing
            tunnel: w1569 -> [w1611] mode=indexing
            tunnel: [w1609] -> w1568
            i -> [w1625]
            stop <- w1615 stop-if-true
            w1628 = 100 ("x")
            n578 = Add(x=w1624, y=w1625) -> (x+y=w1623:i32)
            n579 = call "Operation (SubVI).vi"("error in (no error)"=w1618, "On/Off"=TRUE, "Operation"=w1614, "DAQmx Device Name"=w1617) -> ("error out"=w1631:errorcluster)  [unwired: 7 in]
            n580 = control-ref of="Motor Speed RPM Serial"() -> (w1632:refnum<vi>)
            n581 = control-ref of="Pannel User Message"() -> (w1634:refnum<vi>)
            n582 = control-ref of="Stop Button"() -> (w1637:refnum<vi>)
            n583 = call "Write panel message Kinetics (SubVI).vi"(4:"rpm"=w1632, 5:"rpm"=TRUE ("rpm"), "PrintTime"=TRUE, "Stop"=w1637, "error in (no error)"=w1631, "Time to wait"=30.0, "Strin"=w1616, "String in"=w1634) -> ("error out"=w1630:errorcluster, "Stopped"=w1615:bool)  [unwired: 2 in]
            n584 = property on="Motor Speed RPM Serial" class="DigNum (strict)"(error in=w1630) -> (error out=w1622:errorcluster, "Value"=w1621:dbl)  [unwired: 1 in, 1 out]
            n585 = Subtract(x=w1629, y=w1628) -> (x-y=w1626:i32)
            n586 = Add(x=w1628, y=w1629) -> (x+y=w1627:i32)
            n587 = In Range and Coerce(upper limit=w1627, x=w1621, lower limit=w1626) -> (In Range?=w1620:bool)  [unwired: 1 out]
            n588 = Build Array(w1612, w1611) -> (w1610:T12)
            n589 = call "PassOrFail (SubVI).vi"("index (row)"=w1623, "error in (no error)"=w1622, "Data in"=w1621, "Pass?Fail"=w1620, "Table in"=w1619) -> ("error out"=w1608:errorcluster)  [unwired: 6 in]
            n590 = for {
              tunnel: w1617 -> [w1644]
              tunnel: w1613 -> [w1643] mode=indexing
              tunnel: w1610 -> [w1642] mode=indexing
              tunnel: [w1640] -> w1609
              tunnel: w1608 -> [w1639]
              n591 = call "Operation (SubVI).vi"("error in (no error)"=w1639, "On/Off"=w1643, "Operation"=w1642, "DAQmx Device Name"=w1644) -> ("error out"=w1641:errorcluster)  [unwired: 7 in]
              n592 = call "Time Delay13"("error in (no error)"=w1641) -> ("error out"=w1640:errorcluster)  [unwired: 10 in]
            }
          }
          n593 = for {
            tunnel: w1568 -> [w1598]
            tunnel: w1579 -> [w1597] mode=indexing
            n594 = local read "DAQmx Device Name"() -> (w1599:tag)
            n595 = call "Operation (SubVI).vi"("error in (no error)"=w1598, "On/Off"=FALSE, "Operation"=w1597, "DAQmx Device Name"=w1599) -> ()  [unwired: 7 in, 1 out]
          }
        }
        frame "Analog Voltage Test" {
          w1652 = T12 [enum."Init", enum."PowerSuply"] items=["Init", "0 ohm", "6 ohm", "13.2 ohm", "15 ohm", "25.9 ohm", "33 ohm", "Down", "Up", "Venable", "Firmware", "PowerSuply"]
          w1676 = dbl[] [0.0, 1.0, 2.0, 3.0, 4.0, 4.5]
          n596 = control-ref of="Pannel User Message"() -> (w1684:refnum<vi>)
          n597 = Concatenate Strings(w1678, " in process..." ("string")) -> (w1658:string)
          n598 = property class="Str"(reference=w1684, error in=w1680, "Value"=w1658) -> (error out=w1683:errorcluster)  [unwired: 1 out]
          n599 = call "Table_ScrollaBarMarvin.vi"("error in"=w1683, "Line to focus"=w1678, "reference in"=w1679) -> ("error out"=w1682:errorcluster)  [unwired: 2 out]
          n600 = local read "DAQmx Device Name"() -> (w1650:tag)
          n601 = call "Find_Number_LineMARVIN.vi"("Test Paragraph"=w1678, "error in"=w1682, "TableIn"=w1679) -> ("error out"=w1686:errorcluster, "Line number"=w1685:i32)  [unwired: 2 in, 2 out]
          n602 = call <vilib>:"Clear Errors.vi"("error in (no error)"=w1686) -> ("error out"=w1677:errorcluster)  [unwired: 5 in, 1 out]
          n603 = call "Reset old test Values (SubVI) Kinetics.vi"("error in"=w1677, "Atr in"=w1679, "Test Paragraph"=w1678) -> ("error out"=w1666:errorcluster)  [unwired: 6 in, 2 out]
          n604 = for {
            tunnel: w1650 -> [w1691]
            tunnel: w1652 -> [w1690] mode=indexing
            tunnel: bool[] [FALSE, TRUE] -> [w1689] mode=indexing
            shift-right: [w1688] -> w1663
            shift-left: w1666 -> [w1692]
            n605 = call "Operation (SubVI).vi"("error in (no error)"=w1692, "On/Off"=w1689, "Operation"=w1690, "DAQmx Device Name"=w1691) -> ("error out"=w1688:errorcluster)  [unwired: 7 in]
          }
          n606 = control-ref of="Pannel User Message"() -> (w1665:refnum<vi>)
          n607 = control-ref of="Motor Speed RPM Serial"() -> (w1661:refnum<vi>)
          n608 = control-ref of="Stop Button"() -> (w1659:refnum<vi>)
          n609 = call "Write panel message Kinetics (SubVI).vi"(4:"rpm"=w1661, 5:"rpm"=FALSE ("rpm"), "PrintTime"=FALSE, "Stop"=w1659, "error in (no error)"=w1663, "Time to wait"=5.0, "Strin"=w1658, "String in"=w1665) -> ("error out"=w1657:errorcluster)  [unwired: 2 in, 1 out]
          n610 = local read "DAQmx Device Name"() -> (w1669:tag)
          n611 = call "Serial.vi"("error in (no error)"=w1657, "write buffer"="EP=1\r\nVC=0\r\n", "VISA resource name"=w1656) -> ("error out"=w1654:errorcluster)  [unwired: 7 in, 1 out]
          n612 = while {
            tunnel: [w1695] -> w1651
            tunnel: [TRUE] -> w1655
            tunnel: w1654 -> [w1693]
            stop <- w1697 stop-if-true
            n613 = control-ref of="Motor Speed RPM Serial"() -> (w1699:refnum<vi>)
            n614 = property class="DigNum (strict)"(reference=w1699, error in=w1693) -> (error out=w1695:errorcluster, "Value"=w1698:dbl)  [unwired: 1 out]
            n615 = Less Or Equal?(x=w1698, y=50.0) -> (x <= y?=w1697:bool)
          }
          "Analogtest" <- w1655
          n616 = call "Operation (SubVI).vi"("error in (no error)"=w1651, "On/Off"=FALSE, "Operation"=T5."PowerSuply", "DAQmx Device Name"=w1650) -> ("error out"=w1647:errorcluster)  [unwired: 7 in]
          n617 = call "Time Delay14"("error in (no error)"=w1647, "Delay Time (s)"=20.0) -> ("error out"=w1646:errorcluster)  [unwired: 9 in]
          n618 = for {
            tunnel: w1676 -> [w1710] mode=indexing
            tunnel: w1656 -> [w1709]
            tunnel: w1679 -> [w1708]
            tunnel: w1646 -> [w1703]
            tunnel: w1685 -> [w1707]
            tunnel: w1676 -> [w1706]
            tunnel: w1658 -> [w1705]
            tunnel: [w1703] -> w1675
            shift-right: [w1702] -> _
            shift-left: T10."Init" -> [w1711]
            tunnel: [w1701] -> w1670
            tunnel: w1669 -> [w1700]
            i -> [w1704]
            n619 = while {
              shift-right: [w1717] -> w1702
              shift-left: w1711 -> [w1723]
              tunnel: w1710 -> [w1722]
              tunnel: w1709 -> [w1721]
              tunnel: w1708 -> [w1720]
              tunnel: w1707 -> [w1719]
              tunnel: w1706 -> [w1718]
              tunnel: w1705 -> [w1716]
              tunnel: w1704 -> [w1715]
              tunnel: [w1713] -> w1701
              tunnel: w1700 -> [w1712]
              stop <- w1714 stop-if-true
              n620 = case shown="\"AI0/3\"" w1723 {
                tunnel: w1722 -> [_ w1728 w1763 w1769 _ _]
                tunnel: w1721 -> [_ _ _ _ _ w1790]
                tunnel: w1720 -> [_ w1735 _ _ _ w1812]
                tunnel: w1719 -> [_ w1734 _ _ _ w1811]
                tunnel: w1718 -> [_ _ _ _ _ w1810]
                tunnel: [T10."AO0" T10."Exit" T10."Wait" T10."AI0/3" T10."Read" w1794] -> w1717
                tunnel: [TRUE _ _ w1765 TRUE _] -> w1714
                tunnel: w1716 -> [_ _ _ w1773 _ _]
                tunnel: w1715 -> [_ w1729 _ _ _ _]
                tunnel: [_ _ _ w1765 _ _] -> w1713
                tunnel: w1712 -> [_ w1727 w1762 _ _ w1797]
                frame "Exit", Default {
                }
                frame "AI0/3" {
                  n621 = Increment(x=w1734) -> (x+1=w1733:i32)
                  n622 = property on="Motor Speed RPM Serial" class="DigNum (strict)"() -> ("Value"=w1737:dbl)  [unwired: 2 in, 2 out]
                  n623 = Multiply(x=w1729, y=2) -> (x*y=w1731:i32)
                  n624 = call "Aquire AI0"("device name"=w1727) -> ("data"=w1738:dynamicdata)  [unwired: 16 in, 2 out]
                  n625 = Add(x=w1733, y=w1731) -> (x+y=w1732:i32)
                  n626 = property on="Offset" class="DigNum (strict)" props=["Value"]() -> ()  [unwired: 2 in, 3 out]
                  n627 = To Double Precision Float(number=w1738) -> (double precision float=w1726:dbl)
                  n628 = Build Array(w1726, w1737) -> (w1736:dbl[])
                  n629 = for {
                    tunnel: w1736 -> [w1740] mode=indexing
                    tunnel: w1735 -> [w1745]
                    tunnel: w1732 -> [w1747]
                    tunnel: w1729 -> [w1743]
                    tunnel: w1728 -> [w1741]
                    i -> [w1744]
                    n630 = case shown="0, Default" w1744 {
                      tunnel: w1743 -> [_ w1755]
                      tunnel: [w1749 w1758] -> w1742
                      tunnel: w1741 -> [w1751 _]
                      tunnel: w1740 -> [w1748 w1757]
                      frame 0, Default {
                        w1750 = 0.2 ("y")
                        n631 = Add(x=w1750, y=w1751) -> (x+y=w1752:dbl)
                        n632 = Subtract(x=w1751, y=w1750) -> (x-y=w1753:dbl)
                        n633 = In Range and Coerce(upper limit=w1752, x=w1748, lower limit=w1753) -> (In Range?=w1749:bool)  [unwired: 1 out]
                      }
                      frame 1 {
                        w1759 = 200.0 ("y")
                        n634 = property on="SpeedLimit" class="Arr (strict)"() -> ("Value"=w1756:dbl[])  [unwired: 2 in, 2 out]
                        n635 = Index Array(array=w1756, index=w1755) -> (element=w1754:dbl)
                        n636 = Add(x=w1759, y=w1754) -> (x+y=w1760:dbl)
                        n637 = Subtract(x=w1754, y=w1759) -> (x-y=w1761:dbl)
                        n638 = In Range and Coerce(upper limit=w1760, x=w1757, lower limit=w1761) -> (In Range?=w1758:bool)  [unwired: 1 out]
                      }
                    }
                    n639 = Add(x=w1747, y=w1744) -> (x+y=w1746:i32)
                    n640 = call "PassOrFail (SubVI).vi"("index (row)"=w1746, "Data in"=w1740, "Pass?Fail"=w1742, "Table in"=w1745) -> ()  [unwired: 7 in, 1 out]
                  }
                }
                frame "AO0" {
                  n641 = call "Generate AO0"("data"=w1763, "device name"=w1762) -> ()  [unwired: 16 in, 2 out]
                }
                frame "Wait" {
                  n642 = Number To Fractional String(number=w1769, precision (6)=i16 1) -> (F-format string=w1767:string)  [unwired: 2 in]
                  n643 = Concatenate Strings(w1773, "\r\n", "Analog Output: ", w1767, "V." ("string")) -> (w1766:string)
                  n644 = control-ref of="Pannel User Message"() -> (w1775:refnum<vi>)
                  n645 = control-ref of="Motor Speed RPM Serial"() -> (w1774:refnum<vi>)
                  n646 = control-ref of="Stop Button"() -> (w1779:refnum<vi>)
                  n647 = call "Write panel message Kinetics (SubVI).vi"(4:"rpm"=w1774, 5:"rpm"=TRUE ("rpm"), "PrintTime"=TRUE, "Stop"=w1779, "Time to wait"=20.0, "Strin"=w1766, "String in"=w1775) -> ("Stopped"=w1765:bool)  [unwired: 3 in, 1 out]
                }
                frame "Read" {
                  n648 = One Button Dialog(message="No connection.") -> ()  [unwired: 1 in, 1 out]
                }
                frame "Init" {
                  w1804 = T12 [enum."PowerSuply", enum."Venable"] items=["Init", "0 ohm", "6 ohm", "13.2 ohm", "15 ohm", "25.9 ohm", "33 ohm", "Down", "Up", "Venable", "Firmware", "PowerSuply"]
                  n649 = for {
                    tunnel: w1804 -> [w1819] mode=indexing
                    tunnel: bool[] [TRUE, TRUE] -> [w1818] mode=indexing
                    tunnel: [w1817] -> w1784
                    tunnel: dbl[] [10.0, 2.0] -> [w1815] mode=indexing
                    tunnel: w1797 -> [w1814]
                    n650 = call "Operation (SubVI).vi"("On/Off"=w1818, "Operation"=w1819, "DAQmx Device Name"=w1814) -> ("error out"=w1816:errorcluster)  [unwired: 8 in]
                    n651 = call "Time Delay11"("error in (no error)"=w1816, "Delay Time (s)"=w1815) -> ("error out"=w1817:errorcluster)  [unwired: 9 in]
                  }
                  n652 = call "Aquire AI4"("error in"=w1784, "device name"=w1797) -> ("data"=w1798:dynamicdata, "error out"=w1786:errorcluster)  [unwired: 15 in, 1 out]
                  n653 = call "Serial.vi"("error in (no error)"=w1786, "write buffer"="AG[1]\r\n", "VISA resource name"=w1790) -> ("error out"=w1785:errorcluster, "read buffer"=w1789:string)  [unwired: 7 in]
                  n654 = Fract/Exp String To Number(string=w1789, default (0 dbl)=0.0 ("default (0 DBL)")) -> (number=w1787:dbl)  [unwired: 2 in, 1 out]
                  n655 = Equal To 0?(x=w1787) -> (x = 0?=w1796:bool)
                  n656 = for {
                    tunnel: w1790 -> [w1824]
                    tunnel: [w1820] -> w1806
                    tunnel: string[] ["EP=1\r\n", "VC=0\r\n", "CS[0]=0\r\n", "AG[1]\r\n"] -> [w1823] mode=indexing
                    tunnel: w1785 -> [w1821]
                    n657 = call "Time Delay3"("error in (no error)"=w1821) -> ("error out"=w1822:errorcluster)  [unwired: 10 in]
                    n658 = call "Serial.vi"("error in (no error)"=w1822, "write buffer"=w1823, "VISA resource name"=w1824) -> ("read buffer"=w1820:string)  [unwired: 7 in, 1 out]
                  }
                  n659 = Select(t=T10."Read", s=w1796, f=T10."AO0") -> (s? t:f=w1794:T10)
                  n660 = Fract/Exp String To Number(string=w1806, default (0 dbl)=sgl 0.0 ("default (0 DBL)")) -> (number=w1792:sgl)  [unwired: 2 in, 1 out]
                  n661 = To Double Precision Float(number=w1798) -> (double precision float=→"Offset":dbl)
                  n662 = Add(x=w1811, y=2) -> (x+y=w1809:i32)
                  n663 = for {
                    tunnel: w1812 -> [w1836]
                    tunnel: w1809 -> [w1835]
                    tunnel: w1810 -> [w1831] mode=indexing
                    tunnel: w1792 -> [w1832]
                    tunnel: [w1829] -> w1801
                    tunnel: [w1825] -> w1807 mode=indexing
                    i -> [w1827]
                    n664 = Multiply(x=w1827, y=2) -> (x*y=w1828:i32)
                    n665 = Multiply(x=w1832, y=w1831) -> (x*y=w1825:dbl)
                    n666 = Add(x=w1835, y=w1828) -> (x+y=w1834:i32)
                    n667 = Number To Fractional String(number=w1825, precision (6)=i16 1) -> (F-format string=w1830:string)  [unwired: 2 in]
                    n668 = call "InsertSingleData.vi"("String In"=w1830, "Col"=2, "Row"=w1834, "Table in"=w1836) -> ("error out"=w1829:errorcluster)  [unwired: 7 in]
                  }
                  "SpeedLimit" <- w1807
                  n669 = property on="Analogtest" class="Bool (strict)"(error in=w1801, "Value"=FALSE ("Analogtest")) -> ()  [unwired: 1 in, 2 out]
                }
              }
            }
          }
          n670 = local read "DAQmx Device Name"() -> (w1668:tag)
          n671 = call "Generate AO"("data"=0.0, "error in"=w1675, "device name"=w1668) -> ("error out"=w1671:errorcluster)  [unwired: 15 in, 1 out]
          n672 = call "Operation (SubVI).vi"("error in (no error)"=w1671, "On/Off"=FALSE, "Operation"=T5."Venable", "DAQmx Device Name"=w1668) -> ()  [unwired: 7 in, 1 out]
        }
        frame "Motor Run Test" {
          n673 = control-ref of="Pannel User Message"() -> (w1857:refnum<vi>)
          n674 = Concatenate Strings(w1839, " in process..." ("Strin")) -> (w1844:string)
          n675 = property class="Str"(reference=w1857, error in=w1854, "Value"=w1844) -> (error out=w1856:errorcluster)  [unwired: 1 out]
          n676 = call "Table_ScrollaBarMarvin.vi"("error in"=w1856, "Line to focus"=w1839, "reference in"=w1847) -> ()  [unwired: 3 out]
          n677 = call "Reset old test Values (SubVI) Kinetics.vi"("Atr in"=w1847, "Test Paragraph"=w1839) -> ("error out"=w1855:errorcluster)  [unwired: 7 in, 2 out]
          n678 = call "Find_Number_LineMARVIN.vi"("Test Paragraph"=w1839, "error in"=w1855, "TableIn"=w1847) -> ("error out"=w1852:errorcluster, "Line number"=w1846:i32)  [unwired: 2 in, 2 out]
          n679 = Increment(x=w1846) -> (x+1=w1845:i32)
          n680 = while {
            tunnel: w1852 -> [w1860]
            tunnel: w1840 -> [w1867]
            shift-right: [w1865] -> _
            shift-left: T11."Init" -> [w1866]
            tunnel: w1847 -> [w1864]
            tunnel: w1845 -> [w1863]
            tunnel: w1844 -> [w1861]
            tunnel: [w1860] -> w1841
            tunnel: [w1858] -> w1838
            i -> [w1862]
            stop <- w1859 stop-if-true
            n681 = case shown="\"ReadCurrent\"" w1866 {
              tunnel: w1860 -> [_ w1873 w1894 w1931 w1940]
              tunnel: w1867 -> [_ _ _ w1932 w1950]
              tunnel: [T11."Exit" T11."ReadTemp" w1891 T11."ReadCurrent" T11."ReadTemp"] -> w1865
              tunnel: w1864 -> [_ _ w1905 w1926 _]
              tunnel: w1863 -> [_ _ w1907 w1928 _]
              tunnel: w1862 -> [_ _ w1908 w1929 _]
              tunnel: w1861 -> [_ w1874 w1893 _ _]
              tunnel: [TRUE ("Stopped") w1871 w1887 _ _] -> w1859
              tunnel: [_ w1871 _ _ _] -> w1858
              frame "Exit", Default {
              }
              frame "Wait" {
                n682 = control-ref of="Motor Speed RPM Serial"() -> (w1879:refnum<vi>)
                n683 = control-ref of="Pannel User Message"() -> (w1878:refnum<vi>)
                n684 = control-ref of="Stop Button"() -> (w1877:refnum<vi>)
                n685 = call "Write panel message Kinetics (SubVI).vi"(4:"rpm"=w1879, 5:"rpm"=TRUE ("rpm"), "PrintTime"=TRUE, "Stop"=w1877, "error in (no error)"=w1873, "Time to wait"=1140.0, "Strin"=w1874, "String in"=w1878) -> ("Stopped"=w1871:bool)  [unwired: 2 in, 1 out]
              }
              frame "ReadCurrent" {
                w1903 = 3.0 ("x")
                n686 = control-ref of="Motor Speed RPM Serial"() -> (w1900:refnum<vi>)
                n687 = control-ref of="Pannel User Message"() -> (w1899:refnum<vi>)
                n688 = control-ref of="Stop Button"() -> (w1898:refnum<vi>)
                n689 = call "Write panel message Kinetics (SubVI).vi"(4:"rpm"=w1900, 5:"rpm"=TRUE ("rpm"), "PrintTime"=TRUE, "Stop"=w1898, "error in (no error)"=w1894, "Time to wait"=59.0, "Strin"=w1893, "String in"=w1899) -> ("error out"=w1890:errorcluster, "Stopped"=w1892:bool)  [unwired: 2 in]
                n690 = property on="UUT" class="Str"() -> ("Value"=w1889:string)  [unwired: 2 in, 2 out]
                n691 = case shown="\"True\", Default" w1889 {
                  tunnel: [w1909 w1911] -> w1888
                  tunnel: w1890 -> [_ _]
                  frame "Condenser India", "Condenser Merkava" {
                    n692 = call "Current prob"() -> ("Current"=w1909:dbl)  [unwired: 17 in, 2 out]
                  }
                  frame "True", Default {
                    n693 = local read "CurrentOut"() -> (w1910:dbl)
                    n694 = To Double Precision Float(number=w1910) -> (double precision float=w1911:dbl)
                  }
                }
                n695 = case shown="2, Default" w1908 {
                  tunnel: w1907 -> [w1914 w1917]
                  tunnel: [w1913 w1918] -> w1906
                  tunnel: [T11."Wait" T11."Exit"] -> w1891
                  frame 2, Default {
                    n696 = Increment(x=w1914) -> (x+1=w1913:i32)
                  }
                  frame 5 {
                    n697 = Add(x=w1917, y=3) -> (x+y=w1918:i32)
                  }
                }
                n698 = call "ValFromATR(SubVI).vi"("Row"=w1906, "Table in"=w1905) -> ("Val"=w1904:dbl)  [unwired: 8 in, 1 out]
                n699 = Add(x=w1903, y=w1904) -> (x+y=w1902:dbl)
                n700 = Subtract(x=w1904, y=w1903) -> (x-y=w1901:dbl)
                n701 = local read "DAQmx Device Name"() -> (w1884:tag)
                n702 = In Range and Coerce(upper limit=w1902, x=w1888, lower limit=w1901) -> (In Range?=w1882:bool)  [unwired: 1 out]
                n703 = Not(x=w1882) -> (.not. x?=w1886:bool)
                n704 = Compound Arithmetic op=OR(w1892, w1886) -> (w1887:bool)
                n705 = Not(x=w1882) -> (.not. x?=w1885:bool)
                n706 = call "PassOrFail (SubVI).vi"("index (row)"=w1906, "Data in"=w1888, "Pass?Fail"=w1882, "Table in"=w1905) -> ("error out"=w1880:errorcluster)  [unwired: 7 in]
                n707 = call "Operation (SubVI).vi"("error in (no error)"=w1880, "On/Off"=w1882, "Operation"=T5."PowerSuply", "DAQmx Device Name"=w1884) -> ("error out"=w1881:errorcluster)  [unwired: 7 in]
                n708 = call "Display Message to User7"("error in (no error)"=w1881, "Enable"=w1885) -> ()  [unwired: 8 in, 2 out]
              }
              frame "ReadTemp" {
                w1924 = 15.0 ("x")
                n709 = case shown="4" w1929 {
                  tunnel: w1928 -> [w1934 w1936]
                  tunnel: [w1934 w1937] -> w1927
                  frame 1, Default {
                  }
                  frame 4 {
                    n710 = Add(x=w1936, y=2) -> (x+y=w1937:i32)
                  }
                }
                n711 = call "Serial.vi"("error in (no error)"=w1931, "write buffer"="TA[1]\r\n", "VISA resource name"=w1932) -> ("read buffer"=w1930:string)  [unwired: 7 in, 1 out]
                n712 = call "ValFromATR(SubVI).vi"("Row"=w1927, "Table in"=w1926) -> ("Val"=w1925:dbl)  [unwired: 8 in, 1 out]
                n713 = Fract/Exp String To Number(string=w1930) -> (number=w1920:dbl)  [unwired: 3 in, 1 out]
                n714 = Add(x=w1924, y=w1925) -> (x+y=w1923:dbl)
                n715 = Subtract(x=w1925, y=w1924) -> (x-y=w1922:dbl)
                n716 = In Range and Coerce(upper limit=w1923, x=w1920, lower limit=w1922) -> (In Range?=w1921:bool)  [unwired: 1 out]
                n717 = call "PassOrFail (SubVI).vi"("index (row)"=w1927, "Data in"=w1920, "Pass?Fail"=w1921, "Table in"=w1926) -> ()  [unwired: 7 in, 1 out]
              }
              frame "Init" {
                n718 = local read "DAQmx Device Name"() -> (w1941:tag)
                n719 = call "Operation (SubVI).vi"("error in (no error)"=w1940, "On/Off"=TRUE, "Operation"=T5."PowerSuply", "DAQmx Device Name"=w1941) -> ("error out"=w1939:errorcluster)  [unwired: 7 in]
                n720 = call "Time Delay15"("error in (no error)"=w1939) -> ("error out"=w1938:errorcluster)  [unwired: 10 in]
                n721 = property on="UUT" class="Str"(error in=w1938) -> (error out=w1949:errorcluster, "Value"=w1952:string)  [unwired: 1 in, 1 out]
                n722 = case shown="\"BLDC 60A\"" w1952 {
                  tunnel: ["EP=1\r\nVC=3700\r\n" ("write buffer") "EP=1\r\nVC=9980\r\n" ("write buffer") "EP=1\r\nCL[0]=55\r\nVC=11300\r\n" ("write buffer") "EP=1\r\n" ("write buffer")] -> w1951
                  frame "BLDC 30A", Default {
                  }
                  frame "BLDC 60A" {
                  }
                  frame "Warrior 60A" {
                  }
                  frame "Condenser India", "Condenser Merkava" {
                  }
                }
                n723 = call "Serial.vi"("error in (no error)"=w1949, "write buffer"=w1951, "VISA resource name"=w1950) -> ("error out"=w1944:errorcluster)  [unwired: 7 in, 1 out]
                n724 = local read "DAQmx Device Name"() -> (w1947:tag)
                n725 = call "Operation (SubVI).vi"("error in (no error)"=w1944, "On/Off"=TRUE, "Operation"=T5."Venable", "DAQmx Device Name"=w1947) -> ()  [unwired: 7 in, 1 out]
              }
            }
          }
          n726 = call "Serial.vi"("error in (no error)"=w1841, "write buffer"="EP=1\r\nVC=0\r\n", "VISA resource name"=w1840) -> ("error out"=w1842:errorcluster)  [unwired: 7 in, 1 out]
          n727 = local read "DAQmx Device Name"() -> (w1848:tag)
          n728 = call "Operation (SubVI).vi"("error in (no error)"=w1842, "On/Off"=FALSE, "Operation"=T5."Venable", "DAQmx Device Name"=w1848) -> ()  [unwired: 7 in, 1 out]
        }
        frame "Set Production Parameters" {
          n729 = control-ref of="Pannel User Message"() -> (w1976:refnum<vi>)
          n730 = Concatenate Strings(w1969, " in process..." ("Strin")) -> (w1973:string)
          n731 = property class="Str"(reference=w1976, error in=w1971, "Value"=w1973) -> (error out=w1975:errorcluster)  [unwired: 1 out]
          n732 = call "Table_ScrollaBarMarvin.vi"("error in"=w1975, "Line to focus"=w1969, "reference in"=w1967) -> ("error out"=w1970:errorcluster)  [unwired: 2 out]
          n733 = call "Reset old test Values (SubVI) Kinetics.vi"("error in"=w1970, "Atr in"=w1967, "Test Paragraph"=w1969) -> ("error out"=w1974:errorcluster)  [unwired: 6 in, 2 out]
          n734 = call "Find_Number_LineMARVIN.vi"("Test Paragraph"=w1969, "error in"=w1974, "TableIn"=w1967) -> ("error out"=w1959:errorcluster, "Line number"=w1965:i32)  [unwired: 2 in, 2 out]
          n735 = local read "DAQmx Device Name"() -> (w1962:tag)
          n736 = call "Operation (SubVI).vi"("error in (no error)"=w1959, "On/Off"=TRUE, "Operation"=T5."PowerSuply", "DAQmx Device Name"=w1962) -> ("error out"=w1961:errorcluster)  [unwired: 7 in]
          n737 = call "Time Delay16"("error in (no error)"=w1961) -> ("error out"=w1957:errorcluster)  [unwired: 10 in]
          n738 = Increment(x=w1965) -> (x+1=w1964:i32)
          n739 = for {
            tunnel: w1968 -> [w1985]
            tunnel: w1967 -> [w1984]
            tunnel: w1957 -> [w1983]
            tunnel: string[] ["SN\r\n", "PN\r\n"] -> [w1981] mode=indexing
            tunnel: w1964 -> [w1978]
            i -> [w1979]
            n740 = call "Serial.vi"("error in (no error)"=w1983, "write buffer"=w1981, "VISA resource name"=w1985) -> ("error out"=w1982:errorcluster, "read buffer"=w1980:string)  [unwired: 7 in]
            n741 = Add(x=w1978, y=w1979) -> (x+y=w1977:i32)
            n742 = case shown="0, Default" w1979 {
              tunnel: w1984 -> [w1994 w2001]
              tunnel: w1982 -> [w1993 w2000]
              tunnel: w1980 -> [w1986 w1996]
              tunnel: w1977 -> [w1987 w1995]
              frame 0, Default {
                n743 = property on="Next SN" class="DigNum (strict)"() -> ("Value"=w1991:i32)  [unwired: 2 in, 2 out]
                n744 = Decrement(x=w1991) -> (x-1=w1992:i32)
                n745 = Number To Decimal String(number=w1992) -> (decimal integer string=w1990:string)  [unwired: 1 in]
                n746 = Equal?(x=w1986, y=w1990) -> (x = y?=w1989:bool)
                n747 = call "PassOrFail (SubVI).vi"("String Res"=w1986, "index (row)"=w1987, "error in (no error)"=w1993, "Data in"=-3.0, "Pass?Fail"=w1989, "Table in"=w1994) -> ()  [unwired: 5 in, 1 out]
              }
              frame 1 {
                n748 = property on="PN" class="Str"() -> ("Value"=w1999:string)  [unwired: 2 in, 2 out]
                n749 = Equal?(x=w1999, y=w1996) -> (x = y?=w1998:bool)
                n750 = call "PassOrFail (SubVI).vi"("String Res"=w1996, "index (row)"=w1995, "error in (no error)"=w2000, "Data in"=-3.0, "Pass?Fail"=w1998, "Table in"=w2001) -> ()  [unwired: 5 in, 1 out]
              }
            }
          }
        }
      }
      "TestinExecution" <- w235
    }
    n751 = flat-sequence {
      tunnel: w219 -> [_]
      frame #0 {
        w229 = T13."Enabled" ("Disabled")
        w230 = FALSE ("Start")
        n752 = local read "DAQmx Device Name"() -> (w228:tag)
        n753 = property on="Start" class="Bool (strict)"("Value"=w230, "DisabledEnum"=w229) -> ()  [unwired: 2 in, 2 out]
        n754 = property on="Report" class="Bool (strict)"("Value"=w230, "DisabledEnum"=w229) -> ()  [unwired: 2 in, 2 out]
        n755 = call "Operation (SubVI).vi"("On/Off"=FALSE, "Operation"=T5."PowerSuply", "DAQmx Device Name"=w228) -> ()  [unwired: 8 in, 1 out]
      }
    }
  }
  n756 = while {
    shift-right: [w2006] -> _
    shift-left: T3."Initialize" -> [w2025]
    shift-right: [w2022] -> _
    shift-left: _ -> [w2021]
    shift-right: [w2020] -> _
    shift-left: w28 -> [w2018]
    shift-right: [w2019] -> _
    shift-left: refnum<vi> refnum ("Config_CANAT") -> [w2017]
    shift-right: [w2015] -> _
    shift-left: w25 -> [w2016]
    tunnel: "ATR" -> [_]
    tunnel: w19 -> [w2014]
    tunnel: w18 -> [w2013]
    shift-right: [w2011] -> _
    shift-left: w2 -> [w2012]
    tunnel: w9 -> [w2010]
    tunnel: w3 -> [w2009]
    tunnel: w17 -> [_]
    tunnel: w26 -> [w2024]
    tunnel: [w2023] -> _
    tunnel: w10 -> [_]
    tunnel: w7 -> [w2007]
    shift-right: [w2004] -> _
    shift-left: w2 -> [w2005]
    shift-right: [w2002] -> _
    shift-left: w2 -> [w2003]
    stop <- w2008 stop-if-true
    n757 = case shown="\"Initialize\"" w2025 {
      tunnel: [T3."MainProgram" w2206 w2269 w2796] -> w2006
      tunnel: [FALSE w2194 FALSE FALSE] -> w2008
      tunnel: [w2065 w2199 w2263 w2789] -> w2023
      tunnel: w2024 -> [_ w2171 w2267 _]
      tunnel: [w2029 refnum<visa-resource-name> refnum ("VISA resource name") w2264 w2794] -> w2022
      tunnel: w2021 -> [_ w2218 w2265 _]
      tunnel: [w2083 w2188 w2259 w2815] -> w2020
      tunnel: [w2068 refnum<vi> refnum ("Config_CANAT") w2260 w2805] -> w2019
      tunnel: w2018 -> [w2083 w2220 w2262 w2815]
      tunnel: w2017 -> [_ w2209 w2261 w2805]
      tunnel: w2016 -> [w2082 w2213 w2258 w2814]
      tunnel: [w2082 w2187 w2257 w2814] -> w2015
      tunnel: w2014 -> [_ _ w2256 _]
      tunnel: w2013 -> [_ _ w2255 _]
      tunnel: w2012 -> [w2080 w2211 w2254 w2812]
      tunnel: [w2080 w2211 w2253 w2812] -> w2011
      tunnel: w2010 -> [w2079 _ w2252 _]
      tunnel: w2009 -> [_ _ w2251 _]
      tunnel: w2007 -> [_ _ w2250 _]
      tunnel: w2005 -> [_ _ w2249 _]
      tunnel: [w2076 w2186 w2248 w2807] -> w2004
      tunnel: w2003 -> [_ _ w2247 _]
      tunnel: [w2076 w2186 w2246 w2807] -> w2002
      frame "Erase ATR Table", Default {
        w2067 = refnum<visa-resource-name> "COMx" ("VISA Kinetics")
        w2076 = 0
        w2078 = T13."Enabled" ("Disabled")
        w2085 = FALSE ("Visible")
        n758 = property on="Serial Com" class="Bool"(error in=errorcluster {"status"=FALSE, "code"=0, "source"=""} ("error out"), "Visible"=FALSE) -> (error out=w2081:errorcluster)  [unwired: 1 in, 1 out]
        n759 = property on="VISA Kinetics" class="VISAName"(error in=w2081, "Visible"=w2085, "Value"=w2067) -> (error out=w2087:errorcluster)  [unwired: 1 in, 1 out]
        n760 = property on="Serial Status" class="Bool (strict)"(error in=w2087, "Value"=w2085) -> (error out=w2074:errorcluster)  [unwired: 1 in, 1 out]
        n761 = property on="Pannel User Message" class="Str"(error in=w2074, "Value"="Select a UUT from list bellow:") -> (error out=w2073:errorcluster)  [unwired: 1 in, 1 out]
        n762 = call "UUT select.vi"("error constant"=w2073) -> ("error constant 2"=w2053:errorcluster, 2:"UUT Out"=w2028:string, 3:"UUT Out"=w2072:u16)  [unwired: 8 in]
        "UUT" <- w2028
        n763 = property on="Pannel User Message" class="Str"(error in=w2053, "Value"="Tester initialization in process..." ("Pannel User Message")) -> (error out=w2052:errorcluster)  [unwired: 1 in, 1 out]
        n764 = call "ATRBuild.vi"("error constant"=w2052, "UUT In"=w2072) -> ("error constant 2"=w2071:errorcluster, "TestArray"=→"TestArray":string[], "TestArray Out"=w2070:string[][])  [unwired: 7 in]
        n765 = for {
          tunnel: w2070 -> [w2154] mode=indexing
          tunnel: w2071 -> [w2152]
          tunnel: [w2151] -> w2077
          tunnel: w2070 -> [w2150]
          i -> [w2153]
          n766 = for {
            tunnel: w2154 -> [_] mode=indexing
            tunnel: w2153 -> [w2160]
            tunnel: w2152 -> [w2157]
            tunnel: [w2156] -> w2151
            tunnel: w2150 -> [w2155]
            i -> [w2161]
            n767 = Bundle By Name(cluster=T14 {"Row"=0, "Column"=0} ("Active Cell:Active Cell"), "Row"=w2160, "Column"=w2161) -> (w2159:T14)
            n768 = control-ref of="ATR"() -> (w2158:refnum<vi>)
            n769 = property class="Tbl (strict)"(reference=w2158, error in=w2157, "Active Cell"=w2159, "Cell BG Color"=u32 16777226, "Value"=w2155) -> (error out=w2156:errorcluster)  [unwired: 1 out]
          }
        }
        n770 = call "DataFrom_ini (SubVI).vi"("error in (no error)"=w2077, "UUT"=w2028, "appended path"=w2079) -> ("error out"=w2034:errorcluster, "FileName"=w2062:string, "Next SN"=w2044:i32, "UUT SoftwareVer"=w2043:string, "ParamVersion"=→"ParamVersion":string, "PN"=w2041:string)  [unwired: 3 in]
        "UUT SoftwareVer" <- w2043
        "Next SN" <- w2044
        "FileName" <- w2062
        "PN" <- w2041
        n771 = Decrement(x=w2044) -> (x-1=w2045:i32)
        n772 = Number To Decimal String(number=w2045) -> (decimal integer string=w2042:string)  [unwired: 1 in]
        n773 = control-ref of="ATR"() -> (w2058:refnum<vi>)
        n774 = Build Array(w2043, w2043, w2042, w2041) -> (w2040:string[])
        n775 = call "Boards S/N"("error in (no error)"=w2034) -> ("POWER Board S/N"=→"POWER Board S/N":string, "DSP Board S/N"=→"DSP Board S/N":string, "error out"=w2033:errorcluster)  [unwired: 15 in, 1 out]
        n776 = for {
          tunnel: w2033 -> [w2102]
          tunnel: w2058 -> [w2100]
          tunnel: string[] ["RS232 Comm. + Version", "CAN Comm.", "Unit Serial number", "Unit Part number"] -> [w2099] mode=indexing
          tunnel: [w2098] -> w2060
          tunnel: [w2097] -> w2039 mode=indexing
          tunnel: w2040 -> [w2096] mode=indexing
          n777 = call "Find_Number_LineMARVIN.vi"("Test Paragraph"=w2099, "error in"=w2102, "TableIn"=w2100) -> ("error out"=w2101:errorcluster, "Line number"=w2097:i32)  [unwired: 2 in, 2 out]
          n778 = call "InsertSingleData.vi"("String In"=w2096, "error in (no error)"=w2101, "Col"=2, "Row"=w2097, "Table in"=w2100) -> ("error out"=w2098:errorcluster)  [unwired: 6 in]
        }
        n779 = control-ref of="This VI"() -> (w2056:refnum<vi>)
        n780 = Index Array(array=w2039, index=1) -> (element=w2037:i32)
        n781 = call "COM UUT Board.vi"("error in (no error)"=w2060, "VI reference (current VI)"=w2056, "VISA resource name 2"=w2067) -> ("error out"=w2064:errorcluster, ".not. x?"=w2050:bool, "VISA resource name out"=w2063:refnum<visa-resource-name>)  [unwired: 6 in]
        "Serial Status" <- w2050
        n782 = case shown="True" w2050 {
          tunnel: w2064 -> [w2104 w2127]
          tunnel: w2063 -> [w2105 w2126]
          tunnel: [w2105 w2117] -> w2029
          tunnel: [w2104 w2111] -> w2031
          tunnel: w2062 -> [_ w2110]
          tunnel: w2043 -> [_ w2106]
          frame False {
          }
          frame True {
            n783 = VISA Flush I/O Buffer(VISA resource name=w2126, error in (no error)=w2127) -> (VISA resource name out=w2117:refnum<visa-resource-name>, error out=w2125:errorcluster)  [unwired: 1 in]
            n784 = call "Display Message to User2"("error in (no error)"=w2125) -> ("error out"=w2124:errorcluster, "Yes"=w2123:bool)  [unwired: 9 in]
            n785 = case shown="True" w2123 {
              tunnel: w2124 -> [w2128 w2149]
              tunnel: [w2128 w2129] -> w2122
              tunnel: w2117 -> [_ w2147]
              tunnel: w2110 -> [_ w2140]
              frame False {
              }
              frame True {
                w2133 = u16 11 items=["Init", "0 ohm", "6 ohm", "13.2 ohm", "15 ohm", "25.9 ohm", "33 ohm", "Down", "Up", "Venable", "Firmware", "PowerSuply"] ("Operation")
                w2138 = u16 11 items=["Init", "0 ohm", "6 ohm", "13.2 ohm", "15 ohm", "25.9 ohm", "33 ohm", "Down", "Up", "Venable", "Firmware", "PowerSuply"] ("Operation")
                n786 = local read "DAQmx Device Name"() -> (w2131:tag)
                n787 = call "SetParam.vi"("RS"=TRUE, "error in (no error)"=w2149, "Visa"=w2147, "Filein"=w2140) -> ("error out"=w2136:errorcluster)  [unwired: 7 in]
                n788 = call "Operation (SubVI).vi"("error in (no error)"=w2136, "On/Off"=FALSE, "Operation"=w2138, "DAQmx Device Name"=w2131) -> ("error out"=w2135:errorcluster)  [unwired: 7 in]
                n789 = control-ref of="Pannel User Message"() -> (w2146:refnum<vi>)
                n790 = control-ref of="Motor Speed RPM Serial"() -> (w2144:refnum<vi>)
                n791 = control-ref of="Stop Button"() -> (w2145:refnum<vi>)
                n792 = call "Write panel message Kinetics (SubVI).vi"(4:"rpm"=w2144, 5:"rpm"=FALSE ("rpm"), "PrintTime"=TRUE, "Stop"=w2145, "error in (no error)"=w2135, "Time to wait"=20.0, "Strin"="Restart the UUT\nPlease wait...", "String in"=w2146) -> ("error out"=w2132:errorcluster)  [unwired: 2 in, 1 out]
                n793 = call "Operation (SubVI).vi"("error in (no error)"=w2132, "On/Off"=TRUE, "Operation"=w2133, "DAQmx Device Name"=w2131) -> ("error out"=w2130:errorcluster)  [unwired: 7 in]
                n794 = call "Time Delay12"("error in (no error)"=w2130) -> ("error out"=w2129:errorcluster)  [unwired: 10 in]
              }
            }
            n795 = call "Serial.vi"("error in (no error)"=w2122, "write buffer"="SN\r\n", "VISA resource name"=w2117) -> ("error out"=w2118:errorcluster, "read buffer"=w2112:string)  [unwired: 7 in]
            n796 = property on="UUT SN Report" class="Str"("Value"=w2112) -> ()  [unwired: 2 in, 2 out]
            n797 = Decimal String To Number(string=w2112) -> (number=→"Current SN":i32)  [unwired: 2 in, 1 out]
            n798 = call "Serial.vi"("error in (no error)"=w2118, "write buffer"="VR\r\n", "VISA resource name"=w2117) -> ("error out"=w2113:errorcluster, "read buffer"=w2107:string)  [unwired: 7 in]
            n799 = control-ref of="ATR"() -> (w2114:refnum<vi>)
            n800 = call "Find_Number_LineMARVIN.vi"("Test Paragraph"="RS232 Comm. + Version", "TableIn"=w2114) -> ("Line number"=w2115:i32)  [unwired: 3 in, 3 out]
            n801 = Equal?(x=w2107, y=w2106) -> (x = y?=w2108:bool)
            n802 = call "PassOrFail (SubVI).vi"("String Res"=w2107, "index (row)"=w2115, "error in (no error)"=w2113, "Data in"=-3.0, "Pass?Fail"=w2108, "Table in"=w2114) -> ("error out"=w2111:errorcluster)  [unwired: 5 in]
          }
        }
        n803 = case shown="\"Condenser India\", \"Condenser Merkava\"" w2028 {
          tunnel: w2031 -> [w2091 w2094]
          tunnel: [w2091 w2093] -> w2030
          tunnel: w2029 -> [_ w2092]
          frame "False", Default {
          }
          frame "Condenser India", "Condenser Merkava" {
            n804 = call "Serial.vi"("error in (no error)"=w2094, "write buffer"="EP=1\r\nVC=1000\r\n", "VISA resource name"=w2092) -> ("error out"=w2093:errorcluster)  [unwired: 7 in, 1 out]
          }
        }
        n805 = call "KineticsCan.vi"("error in"=w2030) -> ("error out"=w2059:errorcluster, "Version"=w2054:string, "Res_Pass_T"=w2027:bool, "Config_CANAT_out"=w2068:refnum<vi>)  [unwired: 7 in]
        n806 = case shown="\"Condenser India\", \"Condenser Merkava\"" w2028 {
          tunnel: w2027 -> [w2089 _]
          tunnel: [w2089 TRUE ("Res_Pass_T")] -> w2026
          frame "False", Default {
          }
          frame "Condenser India", "Condenser Merkava" {
          }
        }
        "CAN Status" <- w2026
        n807 = Equal?(x=w2054, y=w2043) -> (x = y?=w2055:bool)
        n808 = call "PassOrFail (SubVI).vi"("String Res"=w2054, "index (row)"=w2037, "error in (no error)"=w2059, "Data in"=-3.0, "Pass?Fail"=w2055, "Table in"=w2058) -> ("error out"=w2049:errorcluster)  [unwired: 5 in]
        n809 = property on="Pannel User Message" class="Str"(error in=w2049, "Value"="You can press start to execute(s) test(s)." ("Pannel User Message")) -> (error out=w2048:errorcluster)  [unwired: 1 in, 1 out]
        n810 = property on="Start" class="Bool (strict)"(error in=w2048, "DisabledEnum"=w2078) -> (error out=w2066:errorcluster)  [unwired: 1 in, 1 out]
        n811 = property on="Report" class="Bool (strict)"(error in=w2066, "DisabledEnum"=w2078) -> (error out=w2065:errorcluster)  [unwired: 1 in, 1 out]
      }
      frame "Stop" {
        w2186 = 0
        n812 = control-ref of="ATR"() -> (w2185:refnum<vi>)
        n813 = call "PassFailUUT (SubVI).vi"("error in (no error)"=w2171, "Table in"=w2185) -> ("PassFaileUUTresult"=w2178:bool)  [unwired: 7 in, 2 out]
        n814 = property on="Test Failed" class="Bool (strict)"("Value"=w2178) -> ()  [unwired: 2 in, 2 out]
        n815 = flat-sequence {
          tunnel: w2171 -> [w2243]
          tunnel: [w2242] -> w2210
          frame #0 {
            n816 = control-ref of="Pannel User Message"() -> (w2245:refnum<vi>)
            n817 = property class="Str"(reference=w2245, error in=w2243, "Value"="Program Stopped...\r\nPlease turn OFF All Power sinks") -> (error out=w2242:errorcluster)  [unwired: 1 out]
          }
        }
        n818 = Select(t="PASS" ("name or relative path"), s=w2178, f="FAIL" ("name or relative path")) -> (s? t:f=w2177:string)
        n819 = call <vilib>:"Application Directory.vi"() -> ("Application Directory"=w2181:path)
        n820 = Build Path(base path=w2181, name or relative path="data\\TestResult.ini") -> (appended path=w2184:path)
        n821 = call <vilib>:"Open Config Data.vi"("configuration file path"=w2184) -> ("error out"=w2182:errorcluster, "refnum"=w2183:T4)  [unwired: 2 in, 7 out]
        n822 = call-poly <vilib>:"Write Key.vi"("section"="Kinetics", "error in (no error)"=w2182, "value"=w2177, "key"="Result", "refnum"=w2183) -> ("error out"=w2180:errorcluster, "refnum out"=w2179:T4)  [unwired: 4 in, 1 out]
        n823 = call <vilib>:"Close Config Data.vi"("error in (no error)"=w2180, "refnum"=w2179) -> ()  [unwired: 8 in, 2 out]
        n824 = property on="VISA Current" class="VISAName"() -> ("Value"=w2166:refnum<visa-resource-name>)  [unwired: 2 in, 2 out]
        n825 = local read "DAQmx Device Name"() -> (w2170:tag)
        n826 = call "Clear CAN Buffer.vi"("error in (no error)"=w2210, "Cluster in"=w2209) -> ("error out"=w2164:errorcluster)  [unwired: 8 in, 1 out]
        n827 = call "Close CAN Device.vi"("error in (no error)"=w2164, "Cluster in"=w2209) -> ("error out"=w2198:errorcluster)  [unwired: 8 in, 1 out]
        n828 = VISA Close(VISA resource name=w2218, error in (no error)=w2210) -> (error out=w2212:errorcluster)
        n829 = VISA Close(VISA resource name=w2166) -> (error out=w2165:errorcluster)  [unwired: 1 in]
        n830 = property on="Stop Button" class="Bool (strict)"() -> ("Value"=w2190:bool)  [unwired: 2 in, 2 out]
        n831 = call "Operation (SubVI).vi"("On/Off"=FALSE, "Operation"=T5."Init", "DAQmx Device Name"=w2170) -> ("error out"=w2167:errorcluster)  [unwired: 8 in]
        n832 = property on="ClosePanel" class="Bool (strict)"() -> ("Value"=w2191:bool)  [unwired: 2 in, 2 out]
        n833 = Or(x=w2191, y=w2190) -> (x .or. y?=w2189:bool)
        n834 = Flush Queue(queue=w2213, error in (no error)=w2212) -> (queue out=w2215:refnum<queue>, error out=w2214:errorcluster)  [unwired: 1 out]
        n835 = Flush Queue(queue=w2220, error in (no error)=w2212) -> (queue out=w2219:refnum<queue>, error out=w2221:errorcluster)  [unwired: 1 out]
        n836 = case shown="False" w2189 {
          tunnel: w2221 -> [w2223 w2231]
          tunnel: w2219 -> [w2225 w2227]
          tunnel: w2215 -> [w2224 w2226]
          tunnel: w2214 -> [w2222 w2230]
          tunnel: [w2223 w2229] -> w2205
          tunnel: [w2222 w2228] -> w2204
          tunnel: [w2225 w2227] -> w2188
          tunnel: [w2224 w2226] -> w2187
          frame False {
          }
          frame True {
            n837 = Release Queue(queue=w2226, error in (no error)=w2230) -> (error out=w2228:errorcluster)  [unwired: 1 in, 2 out]
            n838 = Release Queue(queue=w2227, error in (no error)=w2231) -> (error out=w2229:errorcluster)  [unwired: 1 in, 2 out]
          }
        }
        n839 = Merge Errors(w2205, w2204, w2198, w2167, w2165) -> (w2203:errorcluster)
        n840 = property on="Refresh Button" class="Bool (strict)"() -> ("Value"=w2192:bool)  [unwired: 2 in, 2 out]
        n841 = call <vilib>:"Clear Errors.vi"("error in (no error)"=w2203) -> ("error out"=w2202:errorcluster)  [unwired: 5 in, 1 out]
        n842 = property on="Stop Button" class="Bool (strict)"() -> ("Value"=w2196:bool)  [unwired: 2 in, 2 out]
        n843 = property on="ClosePanel" class="Bool (strict)"(error in=w2202) -> (error out=w2200:errorcluster, "Value"=w2201:bool)  [unwired: 1 in, 1 out]
        n844 = Not(x=w2192) -> (.not. x?=w2193:bool)
        n845 = Select(t=T3."Initialize", s=w2192, f=T3."Stop") -> (s? t:f=w2206:T3)
        n846 = Not(x=w2196) -> (.not. x?=w2195:bool)
        n847 = Compound Arithmetic op=AND(w2201, w2195, w2193) -> (w2197:bool)
        n848 = case shown="False" w2197 {
          tunnel: w2200 -> [w2234 w2238]
          tunnel: [w2234 w2238] -> w2199
          tunnel: [w2233 w2237] -> w2194
          tunnel: w2192 -> [w2232 _]
          frame False {
            n849 = case shown="False" w2232 {
              tunnel: [TRUE FALSE] -> w2233
              frame False {
              }
              frame True {
              }
            }
          }
          frame True {
            n850 = flat-sequence {
              tunnel: [TRUE] -> w2237
              frame #0 {
              }
              frame #1 {
                n851 = control-ref of="This VI"() -> (w2241:refnum<vi>)
                n852 = property class="VI"(reference=w2241, "FP.State"=T15."Closed" ("Front Panel Window:State")) -> ()  [unwired: 1 in, 2 out]
              }
            }
          }
        }
      }
      frame "MainProgram" {
        n853 = event shown="[7] \"Report\", \"Stop Button\": Value Change" {
          selector: w2256 -> [_ _ _ _ _ _ _ _ _ _ _ _ _]
          dyn-events: _ -> [_ _ _ _ _ _ _ _ _ _ _ _ _]
          timeout: "EventTimeout" -> [_ _ _ _ _ _ _ _ _ _ _ _ _]
          tunnel: [T3."MainProgram" T3."MainProgram" T3."MainProgram" T3."MainProgram" T3."MainProgram" T3."Stop" T3."MainProgram" w2632 T3."MainProgram" T3."MainProgram" T3."MainProgram" T3."Stop" T3."MainProgram"] -> w2269
          tunnel: [w2278 w2393 w2461 w2470 w2481 w2501 w2518 w2678 w2741 w2756 _ w2778 w2779] -> w2263
          tunnel: w2267 -> [w2284 w2393 w2460 w2472 w2481 w2501 _ w2678 w2742 w2755 w2763 w2778 w2779]
          tunnel: [w2275 w2387 w2462 w2471 w2482 w2499 w2510 w2637 w2739 w2753 _ w2776 w2783] -> w2264
          tunnel: w2265 -> [w2275 w2387 w2462 w2471 w2482 w2499 w2510 w2637 w2739 w2753 _ w2776 w2783]
          tunnel: w2262 -> [w2286 w2399 w2456 w2467 w2478 w2498 w2520 w2662 w2738 w2752 w2767 w2775 w2786]
          tunnel: w2261 -> [w2282 w2398 w2457 w2468 w2479 w2497 w2514 w2661 w2737 w2751 w2766 w2774 w2782]
          tunnel: [w2283 w2398 w2457 w2468 w2479 w2497 w2514 w2661 w2737 w2751 w2766 w2774 w2782] -> w2260
          tunnel: [w2285 w2399 w2456 w2467 w2478 w2498 w2520 w2662 w2738 w2752 w2767 w2775 w2786] -> w2259
          tunnel: w2258 -> [w2280 w2397 w2455 w2466 w2477 w2496 w2519 w2660 w2736 w2750 w2765 w2773 w2785]
          tunnel: [w2280 w2397 w2455 w2466 w2477 w2496 w2517 w2660 w2736 w2750 w2765 w2773 w2785] -> w2257
          tunnel: w2255 -> [_ _ _ _ _ _ _ w2615 _ _ _ _ _]
          tunnel: w2254 -> [w2281 w2396 w2454 w2465 w2476 w2494 w2515 w2641 w2735 w2749 w2764 w2772 w2784]
          tunnel: [w2281 w2396 w2454 w2465 w2476 w2494 w2515 w2640 w2735 w2749 w2764 w2772 w2784] -> w2253
          tunnel: w2252 -> [_ w2394 _ _ _ _ _ w2639 _ _ _ _ _]
          tunnel: w2251 -> [_ w2386 _ _ _ _ _ _ _ _ _ _ _]
          tunnel: w2250 -> [_ _ _ _ _ _ _ _ w2734 _ _ _ _]
          tunnel: w2249 -> [_ w2375 w2453 w2464 w2475 w2491 w2513 w2616 w2732 w2748 w2761 w2771 w2781]
          tunnel: [_ w2375 w2453 w2464 w2475 w2491 w2513 w2616 w2732 w2748 w2761 w2771 w2781] -> w2248
          tunnel: w2247 -> [w2277 w2374 w2452 w2463 w2474 w2490 w2512 w2608 w2731 w2747 w2760 w2770 w2780]
          tunnel: [w2276 w2374 w2452 w2463 w2474 w2490 w2512 w2608 w2731 w2747 w2760 w2770 w2780] -> w2246
          event Timeout {
            n854 = event-data() -> ()  [unwired: 1 in, 3 out]
            n855 = disable-structure shown="Enabled" {
              disable-tunnel: w2286 -> [w2303 w2363]
              disable-tunnel: [w2302 w2363] -> w2285
              disable-tunnel: w2284 -> [w2301 w2362]
              disable-tunnel: [w2300 w2360] -> w2283
              disable-tunnel: w2282 -> [w2299 w2360]
              disable-tunnel: [w2296 w2362] -> w2278
              disable-tunnel: w2277 -> [w2294 w2361]
              disable-tunnel: [w2293 w2361] -> w2276
              frame Disabled {
                n856 = property class="Clust (strict)"(reference=w2299, error in=w2301) -> (reference out=w2300:refnum<vi>, error out=w2295:errorcluster, "Value"=w2306:T24)
                n857 = Unbundle By Name(w2306) -> ("DevType"=w2307:T18, "CanIndex"=w2305:T19)
                n858 = call "VCI_Receive.vi"("CANIndex"=w2305, "DevIndex"=u32 0, "DevType"=w2307) -> ("Recieve"=w2304:T25[])  [unwired: 3 in, 5 out]
                n859 = Empty Array?(array=w2304) -> (empty?=w2298:bool)
                n860 = case shown="False" w2298 {
                  tunnel: w2305 -> [w2321 _]
                  tunnel: w2300 -> [w2319 _]
                  tunnel: w2303 -> [w2318 w2351]
                  tunnel: w2295 -> [w2317 w2350]
                  tunnel: w2304 -> [w2322 _]
                  tunnel: [w2312 w2350] -> w2296
                  tunnel: [w2311 w2351] -> w2302
                  tunnel: [TRUE w2345] -> w2297
                  tunnel: w2294 -> [_ w2349]
                  tunnel: [0 w2348] -> w2293
                  frame False {
                    n861 = call "Demo_MakeDispBuff.vi"("Channel"=w2321, "Type"=enum16{"接收", "发送"}."接收", "OBJs"=w2322) -> ("Buffer"=w2320:T26)
                    n862 = for {
                      N: 3 -> [_]
                      tunnel: w2320 -> [w2336]
                      tunnel: w2319 -> [w2335]
                      tunnel: w2318 -> [w2326]
                      tunnel: w2317 -> [w2325]
                      tunnel: [w2328] -> w2315 mode=indexing
                      tunnel: [w2326] -> w2314
                      tunnel: [w2325] -> w2313
                      i -> [w2324]
                      n863 = property class="Clust (strict)"(reference=w2335) -> ("Value"=w2333:T24)  [unwired: 1 in, 2 out]
                      n864 = Index Array(array=w2336, index=w2324) -> (element=w2329:T27)
                      n865 = Unbundle By Name(w2329) -> ("Channel"=w2331:T19, "VCI_CAN_OBJ"=w2334:T25)  [unwired: 2 out]
                      n866 = Unbundle By Name(w2333) -> ("CanIndex"=w2332:T19)
                      n867 = Equal?(x=w2332, y=w2331) -> (x = y?=w2330:bool)
                      n868 = case shown="True" w2330 {
                        tunnel: w2334 -> [_ w2344]
                        tunnel: [w2337 w2340] -> w2328
                        tunnel: T16 {"ID"=0, "MSGTYPE"=0, "LEN"=0, "aDATA"=[]} ("Msg") -> [w2337 w2339]
                        frame False {
                        }
                        frame True {
                          n869 = Unbundle By Name(w2344) -> ("ID"=w2338:u32, "DataLen"=w2343:u8, "Data"=w2341:u8[])
                          n870 = Bundle By Name(cluster=w2339, "ID"=w2338, "MSGTYPE"=u8 0, "LEN"=w2343, "aDATA"=w2341) -> (w2340:T16)
                        }
                      }
                    }
                    n871 = Enqueue Element(queue=w2314, element=w2315, error in (no error)=w2313) -> (queue out=w2311:refnum<queue>, error out=w2312:errorcluster)  [unwired: 2 out]
                  }
                  frame True {
                    n872 = Increment(x=w2349) -> (x+1=w2348:i32)
                    n873 = Greater Or Equal?(x=w2348, y=7) -> (x >= y?=w2346:bool)
                    n874 = Not(x=w2346) -> (.not. x?=w2345:bool)
                  }
                }
                n875 = property on="CAN Status" class="Bool (strict)"("Value"=w2297) -> ()  [unwired: 2 in, 2 out]
              }
              frame Enabled {
                n876 = property on="VISA Current" class="VISAName"() -> ("Value"=w2354:refnum<visa-resource-name>)  [unwired: 2 in, 2 out]
                n877 = Not Equal?(x=w2354, y=refnum<visa-resource-name> "COMx") -> (x != y?=w2355:bool)
                n878 = case shown="True" w2355 {
                  tunnel: w2354 -> [_ w2368]
                  frame False {
                  }
                  frame True {
                    n879 = call "ReadCurrent.vi"("LoopFromMain"=TRUE, "VISA resource name"=w2368) -> ("CurrentSens"=→"CurrentSens":bool, "CurrentOut"=w2366:string)  [unwired: 7 in, 1 out]
                    "Current" <- w2366
                    n880 = Fract/Exp String To Number(string=w2366) -> (number=→"CurrentOut":dbl)  [unwired: 3 in, 1 out]
                  }
                }
                n881 = control-ref of="ATR"() -> (w2352:refnum<vi>)
                n882 = call "PassFailUUT (SubVI).vi"("Table in"=w2352) -> ("PassFaileUUTresult"=w2353:bool)  [unwired: 8 in, 2 out]
                n883 = property on="Test Failed" class="Bool (strict)"("Value"=w2353) -> ()  [unwired: 2 in, 2 out]
                n884 = property on="Automation" class="Bool (strict)"() -> ("Value"=w2359:bool)  [unwired: 2 in, 2 out]
                n885 = property on="Start" class="Bool (strict)"() -> ("Value"=w2357:bool)  [unwired: 2 in, 2 out]
                n886 = Or(x=w2359, y=w2357) -> (x .or. y?=w2358:bool)
                n887 = case shown="False" w2358 {
                  frame False {
                    n888 = property on="Pannel User Message" class="Str"("Value"="You can press start to execute(s) test(s).") -> ()  [unwired: 2 in, 2 out]
                  }
                  frame True {
                  }
                }
              }
            }
            n889 = property on="ClosePanel" class="Bool (strict)"("Value"=FALSE ("ClosePanel")) -> ()  [unwired: 2 in, 2 out]
            n890 = Not Equal?(x=w2275, y=refnum<visa-resource-name> "COMx") -> (x != y?=w2273:bool)
            n891 = property on="Analogtest" class="Bool (strict)"() -> ("Value"=w2271:bool)  [unwired: 2 in, 2 out]
            n892 = Not(x=w2271) -> (.not. x?=w2270:bool)
            n893 = And(x=w2270, y=w2273) -> (x .and. y?=w2272:bool)
            n894 = case shown="True" w2272 {
              tunnel: w2275 -> [_ w2292]
              frame False {
              }
              frame True {
                n895 = call "Serial.vi"("Clear Log"=FALSE, "write buffer"="VC\r\n", "VISA resource name"=w2292) -> ("read buffer"=w2288:string)  [unwired: 7 in, 1 out]
                n896 = Fract/Exp String To Number(string=w2288) -> (number=→"Motor Speed RPM Serial":dbl)  [unwired: 3 in, 1 out]
              }
            }
          }
          event "SetSN": Value Change {
            n897 = event-data() -> ()  [unwired: 1 in, 6 out]
            n898 = property on="UUT" class="Str"() -> ("Value"=w2373:string)  [unwired: 2 in, 2 out]
            n899 = case shown="\"BLDC 30A\", Default" w2373 {
              tunnel: [26 26 26 26 35] -> w2371
              frame "BLDC 30A", Default {
              }
              frame "Warrior 60A" {
              }
              frame "Condenser Merkava" {
              }
              frame "Condenser India" {
              }
              frame "BLDC 60A" {
              }
            }
            n900 = control-ref of="ATR"() -> (w2378:refnum<vi>)
            n901 = property on="Current SN" class="DigNum (strict)"(error in=w2393) -> (error out=w2377:errorcluster, "Value"=w2392:i32)  [unwired: 1 in, 1 out]
            n902 = call "PassFailUUT (SubVI).vi"("error in (no error)"=w2377, "Table in"=w2378) -> ("Total Pass"=w2372:u8)  [unwired: 7 in, 2 out]
            n903 = Equal To 0?(x=w2392) -> (x = 0?=w2389:bool)
            n904 = Equal?(x=w2392, y=-1) -> (x = y?=w2390:bool)
            n905 = Equal?(x=w2372, y=w2371) -> (x = y?=w2370:bool)
            n906 = Or(x=w2390, y=w2389) -> (x .or. y?=w2388:bool)
            n907 = property on="CAN Status" class="Bool (strict)"() -> ("Value"=w2379:bool)  [unwired: 2 in, 2 out]
            n908 = property on="Serial Status" class="Bool (strict)"() -> ("Value"=w2384:bool)  [unwired: 2 in, 2 out]
            n909 = And(x=w2384, y=w2379) -> (x .and. y?=w2380:bool)
            n910 = case shown="True" w2380 {
              tunnel: w2394 -> [_ w2418]
              tunnel: w2388 -> [_ w2407]
              tunnel: w2387 -> [_ w2417]
              tunnel: w2386 -> [_ w2416]
              tunnel: [errorcluster {"status"=FALSE, "code"=0, "source"=""} ("error out") w2415] -> w2383
              tunnel: [w2405 w2414] -> w2385
              tunnel: w2370 -> [_ w2408]
              frame False {
                w2405 = FALSE ("Value")
                n911 = property on="SetSN" class="Bool (strict)"("Value"=w2405) -> ()  [unwired: 2 in, 2 out]
                n912 = call "Display Message to User10"() -> ()  [unwired: 10 in, 2 out]
              }
              frame True {
                n913 = property on="Test Failed" class="Bool (strict)"() -> ("Value"=w2412:bool)  [unwired: 2 in, 2 out]
                n914 = property on="Automation" class="Bool (strict)"() -> ("Value"=w2414:bool)  [unwired: 2 in, 2 out]
                n915 = Not(x=w2412) -> (.not. x?=w2413:bool)
                n916 = Select(t=w2413, s=w2414, f=w2416) -> (s? t:f=w2410:bool)
                n917 = Or(x=w2408, y=w2410) -> (x .or. y?=w2409:bool)
                n918 = And(x=w2407, y=w2409) -> (x .and. y?=w2411:bool)
                n919 = case shown="True" w2411 {
                  tunnel: w2418 -> [_ w2449]
                  tunnel: w2417 -> [_ w2442]
                  tunnel: [w2420 w2434] -> w2415
                  tunnel: w2407 -> [w2419 _]
                  frame False {
                    n920 = case shown="True" w2419 {
                      tunnel: [w2422 w2423] -> w2420
                      frame False {
                        n921 = call "Display Message to User9"() -> ("error out"=w2422:errorcluster)  [unwired: 10 in, 1 out]
                      }
                      frame True {
                        n922 = call "Display Message to User3"() -> ("error out"=w2423:errorcluster)  [unwired: 10 in, 1 out]
                      }
                    }
                    n923 = property on="Automation" class="Bool (strict)"(error in=w2420, "Value"=FALSE ("Automation")) -> ()  [unwired: 1 in, 2 out]
                  }
                  frame True {
                    w2441 = FALSE ("SetSN")
                    n924 = local read "DAQmx Device Name"() -> (w2427:tag)
                    n925 = property on="Next SN" class="DigNum (strict)"() -> ("Value"=w2429:i32)  [unwired: 2 in, 2 out]
                    n926 = call "Operation (SubVI).vi"("On/Off"=FALSE, "Operation"=T5."Venable", "DAQmx Device Name"=w2427) -> ("error out"=w2431:errorcluster)  [unwired: 8 in]
                    n927 = call <vilib>:"Clear Errors.vi"("error in (no error)"=w2431) -> ("error out"=w2432:errorcluster)  [unwired: 5 in, 1 out]
                    n928 = Number To Decimal String(number=w2429) -> (decimal integer string=w2430:string)  [unwired: 1 in]
                    "UUT SN Report" <- w2430
                    n929 = Search and Replace String(input string="EP=1\r\nSN=0\r\n" ("write buffer"), search string="0", replace string=w2430) -> (result string=w2444:string)  [unwired: 5 in, 3 out]
                    n930 = call "Serial.vi"("error in (no error)"=w2432, "Clear Log"=FALSE, "write buffer"=w2444, "VISA resource name"=w2442) -> ("error out"=w2426:errorcluster)  [unwired: 6 in, 1 out]
                    n931 = property on="UUT" class="Str"(error in=w2426) -> ("Value"=w2425:string)  [unwired: 1 in, 2 out]
                    n932 = call <vilib>:"Open Config Data.vi"("create file if necessary (T)"=FALSE, "configuration file path"=w2449) -> ("error out"=w2447:errorcluster, "refnum"=w2448:T4)  [unwired: 1 in, 7 out]
                    n933 = call-poly <vilib>:"Write Key.vi"("section"=w2425, "error in (no error)"=w2447, "value"=w2430, "key"="SN", "refnum"=w2448) -> ("error out"=w2437:errorcluster, "refnum out"=w2436:T4)  [unwired: 4 in, 1 out]
                    n934 = call <vilib>:"Close Config Data.vi"("error in (no error)"=w2437, "refnum"=w2436) -> ("error out"=w2435:errorcluster)  [unwired: 8 in, 1 out]
                    n935 = property on="Current SN" class="DigNum (strict)"("Value"=w2429) -> ()  [unwired: 2 in, 2 out]
                    n936 = property on="SetSN" class="Bool (strict)"(error in=w2435, "Value"=w2441) -> (error out=w2440:errorcluster)  [unwired: 1 in, 1 out]
                    n937 = property on="Automation" class="Bool (strict)"(error in=w2440, "Value"=w2441) -> (error out=w2439:errorcluster)  [unwired: 1 in, 1 out]
                    n938 = Increment(x=w2429) -> (x+1=w2438:i32)
                    n939 = property on="Next SN" class="DigNum (strict)"(error in=w2439, "Value"=w2438) -> (error out=w2434:errorcluster)  [unwired: 1 in, 1 out]
                  }
                }
              }
            }
            n940 = call <vilib>:"Clear Errors.vi"("error in (no error)"=w2383) -> ("error out"=w2376:errorcluster)  [unwired: 5 in, 1 out]
            n941 = property on="SetSN" class="Bool (strict)"(error in=w2376, "Value"=FALSE ("SetSN")) -> (error out=w2382:errorcluster)  [unwired: 1 in, 1 out]
            n942 = case shown="True" w2385 {
              tunnel: w2382 -> [_ _]
              frame False {
              }
              frame True {
                w2451 = TRUE ("Value (Signaling)")
                n943 = property on="Report" class="Bool (strict)"("Val(Sgnl)"=w2451, "Value"=w2451) -> ()  [unwired: 2 in, 2 out]
              }
            }
          }
          event "ATR": Mouse Enter {
            n944 = event-data() -> ()  [unwired: 1 in, 4 out]
            n945 = call-poly <vilib>:"Set Cursor.vi"("error in (no error)"=w2460, "icon"=u16 1) -> ("error out"=w2461:errorcluster)  [unwired: 8 in, 1 out]
          }
          event "ATR": Mouse Leave {
            n946 = event-data() -> ()  [unwired: 1 in, 4 out]
            n947 = call-poly <vilib>:"Set Cursor.vi"("error in (no error)"=w2472, "icon"=u16 0) -> ("error out"=w2470:errorcluster)  [unwired: 8 in, 1 out]
          }
          event "ATR": Mouse Down? {
            n948 = event-data() -> ("Coords"=w2489:T28)  [unwired: 1 in, 4 out]
            n949 = invoke on="ATR" class="Tbl (strict)" method="Point To Row Column"("Point"=w2489) -> ("InBounds"=w2485:bool, "CellPosition"=w2484:T14)  [unwired: 5 in, 4 out]
            n950 = Greater Than 0?(x=w2484) -> (x > 0?=w2488:cluster{"Row":bool, "Column":bool})
            n951 = Cluster To Array(cluster=w2488) -> (array=w2487:bool[])
            n952 = Or Array Elements(Boolean array=w2487) -> (logical OR=w2486:bool)
            n953 = Or(x=w2485, y=w2486) -> (x .or. y?=w2483:bool)
            n954 = event-data("Discard?"=w2483) -> ()  [unwired: 1 in, 1 out]
          }
          event Panel Close? {
            n955 = event-data() -> ("VIRef"=w2495:refnum<vi>)  [unwired: 1 in, 3 out]
            n956 = Close Reference(reference=w2495) -> ()  [unwired: 1 in, 1 out]
            n957 = disable-structure shown="Disabled" {
              frame Disabled {
                n958 = property on="Stop Button" class="Bool (strict)"("Val(Sgnl)"=TRUE ("Stop Button"), "Value"=FALSE ("Stop Button")) -> ()  [unwired: 2 in, 2 out]
              }
              frame Enabled {
              }
            }
            n959 = event-data("Discard?"=TRUE) -> ()  [unwired: 1 in, 1 out]
            "ClosePanel" <- TRUE ("ClosePanel")
          }
          event "Start": Value Change {
            w2508 = string[] []  # TestArray
            n960 = event-data() -> ()  [unwired: 1 in, 2 out]
            n961 = while {
              tunnel: [w2534] -> w2507
              tunnel: [w2533] -> w2505
              shift-right: [w2531] -> _
              shift-left: enum16{"Stop", "Tests", "Bit test", "Start"}."Start" -> [w2532]
              tunnel: w2508 -> [w2530]
              stop <- w2529 stop-if-true
              n962 = case shown="\"Start\"" w2532 {
                tunnel: [w2539 w2544 w2554 w2566] -> w2534
                tunnel: [errorcluster {"status"=FALSE, "code"=0, "source"=""} ("error out") w2543 errorcluster {"status"=FALSE, "code"=0, "source"=""} ("error out") w2564] -> w2533
                tunnel: [w2538 w2550 enum16{"Stop", "Tests", "Bit test", "Start"}."Stop" w2560] -> w2531
                tunnel: w2530 -> [w2539 _ w2554 w2566]
                tunnel: [w2537 w2549 FALSE FALSE] -> w2529
                frame "Stop", Default {
                  n963 = flat-sequence {
                    tunnel: [enum16{"Stop", "Tests", "Bit test", "Start"}."Stop"] -> w2538
                    tunnel: [TRUE] -> w2537
                    frame #0 {
                    }
                  }
                  n964 = property on="Start" class="Bool (strict)"("Value"=FALSE ("Start")) -> ()  [unwired: 2 in, 2 out]
                }
                frame "Tests" {
                  w2548 = T13."Disabled and Grayed Out" ("Disabled")
                  n965 = property on="TestArray" class="Arr (strict)"() -> (error out=w2543:errorcluster, "Value"=w2545:string[])  [unwired: 2 in, 1 out]
                  n966 = call "Start Test Selection (SubVI).vi"("TestArrayIn"=w2545) -> ("AutoOut"=w2542:bool, "TestArrayOut"=w2544:string[])  [unwired: 9 in]
                  "Automation" <- w2542
                  n967 = property on="Start" class="Bool (strict)"("DisabledEnum"=w2548) -> ()  [unwired: 2 in, 2 out]
                  n968 = property on="Report" class="Bool (strict)"("DisabledEnum"=w2548) -> ()  [unwired: 2 in, 2 out]
                  n969 = control-ref of="ATR"() -> (w2546:refnum<vi>)
                  n970 = property on="Stop Button" class="Bool (strict)"("Value"=FALSE ("Stop Burn-in")) -> ()  [unwired: 2 in, 2 out]
                  n971 = case shown="True" w2542 {
                    tunnel: w2546 -> [_ w2551]
                    frame False {
                    }
                    frame True {
                      n972 = call "ResetTable Result (SubVI).vi"("Table in"=w2551) -> ()  [unwired: 11 in]
                    }
                  }
                  n973 = flat-sequence {
                    tunnel: [enum16{"Stop", "Tests", "Bit test", "Start"}."Tests"] -> w2550
                    tunnel: [TRUE] -> w2549
                    frame #0 {
                    }
                  }
                }
                frame "Bit test" {
                }
                frame "Start" {
                  n974 = property on="CAN Status" class="Bool (strict)"() -> (error out=w2563:errorcluster, "Value"=w2562:bool)  [unwired: 2 in, 1 out]
                  n975 = property on="CurrentSens" class="Bool (strict)"() -> ("Value"=w2558:bool)  [unwired: 2 in, 2 out]
                  n976 = property on="Serial Status" class="Bool (strict)"(error in=w2563) -> ("Value"=w2561:bool)  [unwired: 1 in, 2 out]
                  n977 = And(x=w2562, y=w2561) -> (x .and. y?=w2559:bool)
                  n978 = case shown="True" w2559 {
                    tunnel: [w2568 w2571] -> w2564
                    tunnel: [enum16{"Stop", "Tests", "Bit test", "Start"}."Stop" w2570] -> w2560
                    tunnel: w2558 -> [_ w2569]
                    frame False {
                      n979 = call "Display Message to User5"() -> ("error out"=w2568:errorcluster)  [unwired: 10 in, 1 out]
                    }
                    frame True {
                      n980 = case shown="True" w2569 {
                        tunnel: [w2572 w2578] -> w2571
                        tunnel: [enum16{"Stop", "Tests", "Bit test", "Start"}."Stop" enum16{"Stop", "Tests", "Bit test", "Start"}."Tests"] -> w2570
                        frame False {
                          n981 = call "Display Message to User"() -> ("error out"=w2572:errorcluster)  [unwired: 10 in, 1 out]
                        }
                        frame True {
                          n982 = control-ref of="Motor Speed RPM Serial"() -> (w2575:refnum<vi>)
                          n983 = control-ref of="Stop Button"() -> (w2576:refnum<vi>)
                          n984 = control-ref of="Pannel User Message"() -> (w2577:refnum<vi>)
                          n985 = call "Write panel message Kinetics (SubVI).vi"(4:"rpm"=w2575, 5:"rpm"=FALSE ("rpm"), "PrintTime"=FALSE, "Stop"=w2576, "Time to wait"=0.0, "Strin"="TESTER BIT TEST OPERATION IN PROCESS\nPlease wait...", "String in"=w2577) -> ("error out"=w2578:errorcluster)  [unwired: 3 in, 1 out]
                        }
                      }
                    }
                  }
                }
              }
            }
            n986 = Array Size(array=w2507) -> (size(s)=w2506:i32)
            n987 = case shown="1, Default" w2506 {
              tunnel: w2505 -> [w2522 w2524]
              tunnel: [w2522 w2523] -> w2504
              frame 0 {
              }
              frame 1, Default {
                n988 = local read "DAQmx Device Name"() -> (w2528:tag)
                n989 = call "Operation (SubVI).vi"("error in (no error)"=w2524, "On/Off"=TRUE, "Operation"=T5."PowerSuply", "DAQmx Device Name"=w2528) -> ("error out"=w2525:errorcluster)  [unwired: 7 in]
                n990 = call "Time Delay"("error in (no error)"=w2525) -> ("error out"=w2523:errorcluster)  [unwired: 10 in]
              }
            }
            n991 = Bundle By Name(cluster=T1 {"VISA"="COM1", "TestArray"=[]}, "VISA"=w2510, "TestArray"=w2507) -> (w2511:T1)
            n992 = Enqueue Element(queue=w2519, element=w2511, error in (no error)=w2504) -> (queue out=w2517:refnum<queue>, error out=w2518:errorcluster)  [unwired: 2 out]
          }
          event "Report", "Stop Button": Value Change {
            w2618 = T29 1 items=["User Home"=0, "User Desktop"=1, "User Documents"=2, "User Application Data"=3, "User Preferences"=4, "User Temporary"=5, "Public Documents"=6, "Public Application Data"=7, "Public Preferences"=8, "Public Cache"=13, "System Core Libraries"=9, "System Installed Libraries"=10, "Application Files"=11, "Boot Volume Root"=12] ("system directory type")
            w2586 = FALSE ("Report")
            n993 = event-data() -> ("CtlRef"=w2636:refnum<vi>)  [unwired: 1 in]
            n994 = local read "UUT"() -> (w2583:string)
            n995 = call <vilib>:"Get System Directory.vi"("create directory if not found? (F)"=TRUE, "system directory type"=w2618) -> ("system directory"=w2617:path)  [unwired: 9 in]
            n996 = Build Path(base path=w2617, name or relative path="KineticsReports") -> (appended path=w2671:path)
            n997 = property on="CAN Status" class="Bool (strict)"() -> ("Value"=w2621:bool)  [unwired: 2 in, 2 out]
            n998 = property on="Serial Status" class="Bool (strict)"() -> ("Value"=w2622:bool)  [unwired: 2 in, 2 out]
            n999 = call <vilib>:"Check if File or Folder Exists.vi"("path"=w2671) -> ("error out"=w2669:errorcluster, "file or folder exists?"=w2672:bool, "dup path"=w2670:path)  [unwired: 8 in]
            n1000 = To Upper Case(1:w2583) -> (0:w2584:string)
            n1001 = And(x=w2622, y=w2621) -> (x .and. y?=w2623:bool)
            n1002 = case shown="False" w2672 {
              tunnel: w2669 -> [w2728 w2729]
              tunnel: w2670 -> [w2727 w2730]
              tunnel: [w2726 w2730] -> w2620
              tunnel: [w2725 w2729] -> w2674
              frame False {
                n1003 = Create Folder(path (use dialog)=w2727, error in=w2728) -> (created path=w2726:path, error out=w2725:errorcluster)  [unwired: 1 in, 1 out]
              }
              frame True {
              }
            }
            n1004 = case shown="True" w2623 {
              tunnel: [w2679 "" ("read buffer")] -> w2658
              tunnel: [w2679 w2681] -> w2611
              tunnel: w2637 -> [_ w2689]
              tunnel: [w2679 w2698] -> w2614
              tunnel: [w2679 w2682] -> w2612
              tunnel: [w2679 "" ("read buffer")] -> w2630
              frame False {
                w2679 = "N_A" ("read buffer")
              }
              frame True {
                n1005 = call "Serial.vi"("write buffer"="SN\r\n", "VISA resource name"=w2689) -> ("error out"=w2694:errorcluster, "read buffer"=w2696:string)  [unwired: 8 in]
                n1006 = Decimal String To Number(string=w2696) -> (number=w2695:i32)  [unwired: 2 in, 1 out]
                n1007 = Number To Decimal String(number=w2695, width (-)=i16 4) -> (decimal integer string=w2698:string)
                n1008 = call "Serial.vi"("error in (no error)"=w2694, "write buffer"="VR\r\n", "VISA resource name"=w2689) -> ("error out"=w2690:errorcluster, "read buffer"=w2682:string)  [unwired: 7 in]
                n1009 = call "Serial.vi"("error in (no error)"=w2690, "write buffer"="PN\r\n", "VISA resource name"=w2689) -> ("read buffer"=w2680:string)  [unwired: 7 in, 1 out]
                n1010 = String Length(string=w2680) -> (length=w2687:i32)
                n1011 = Subtract(x=6, y=w2687) -> (x-y=w2686:i32)
                n1012 = for {
                  N: w2686 -> [_]
                  shift-right: [w2703] -> w2683
                  shift-left: "" -> [w2702]
                  n1013 = Concatenate Strings(w2702, "0" ("string")) -> (w2703:string)
                }
                n1014 = Concatenate Strings("RD" ("string"), w2683, w2680) -> (w2681:string)
              }
            }
            n1015 = Get Date/Time String(want seconds? (F)=TRUE) -> (date string=w2673:string)  [unwired: 2 in, 1 out]
            n1016 = call <vilib>:"Open Config Data.vi"("create file if necessary (T)"=FALSE, "configuration file path"=w2639) -> ("refnum"=w2649:T4)  [unwired: 1 in, 8 out]
            n1017 = property on="Logger Path" class="Path"(error in=w2674, "Value"=w2620, "StartPath"=w2620) -> (error out=w2652:errorcluster)  [unwired: 1 in, 1 out]
            n1018 = Search and Replace String(replace all?=TRUE ("replace all? (F)"), input string=w2673, search string="/") -> (result string=w2655:string)  [unwired: 5 in, 3 out]
            n1019 = call-poly <vilib>:"Read Key.vi"("section"=w2583, "key"="version", "refnum"=w2649) -> ("error out"=w2644:errorcluster, "value"=w2647:string, "refnum out"=w2646:T4)  [unwired: 5 in, 1 out]
            n1020 = call-poly <vilib>:"Read Key.vi"("section"="Kinetics", "error in (no error)"=w2644, "key"="Tester Software Ver", "refnum"=w2646) -> ("error out"=w2642:errorcluster, "value"=w2613:string, "refnum out"=w2645:T4)  [unwired: 4 in, 1 out]
            n1021 = property on="POWER Board S/N" class="Str"() -> ("Value"=w2591:string)  [unwired: 2 in, 2 out]
            n1022 = Concatenate Strings("ATR" ("string"), w2658, w2614, "_", w2655, ".docx" ("string")) -> (w2653:string)
            n1023 = call <vilib>:"Close Config Data.vi"("error in (no error)"=w2642, "refnum"=w2645) -> ()  [unwired: 8 in, 2 out]
            n1024 = Build Path(base path=w2620, name or relative path=w2653) -> (appended path=w2654:path)
            n1025 = property on="DSP Board S/N" class="Str"() -> ("Value"=w2590:string)  [unwired: 2 in, 2 out]
            n1026 = Concatenate Strings("  Rev-" ("string"), w2647) -> (w2638:string)
            n1027 = while {
              tunnel: w2653 -> [w2710]
              tunnel: w2620 -> [w2707]
              shift-right: [w2709] -> w2651
              shift-left: w2654 -> [w2708]
              shift-right: [w2705] -> w2640
              shift-left: w2641 -> [w2706]
              tunnel: w2652 -> [w2711]
              tunnel: [w2712] -> w2619
              stop <- w2704 continue-if-true
              n1028 = call <vilib>:"Check if File or Folder Exists.vi"("error in (no error)"=w2711, "path"=w2708) -> ("error out"=w2712:errorcluster, "file or folder exists?"=w2704:bool)  [unwired: 7 in, 1 out]
              n1029 = case shown="True" w2704 {
                tunnel: w2710 -> [_ w2724]
                tunnel: w2706 -> [_ w2716]
                tunnel: [w2714 w2721] -> w2709
                tunnel: w2708 -> [w2714 _]
                tunnel: w2707 -> [_ w2722]
                tunnel: [1 w2715] -> w2705
                frame False {
                }
                frame True {
                  w2717 = ".docx" ("search string")
                  n1030 = Search and Replace String(input string=w2724, search string=w2717) -> (result string=w2723:string)  [unwired: 6 in, 3 out]
                  n1031 = Number To Decimal String(number=w2716) -> (decimal integer string=w2719:string)  [unwired: 1 in]
                  n1032 = call <vilib>:"Space Constant.vi"() -> ("String"=w2718:string)
                  n1033 = Concatenate Strings(w2723, w2718, w2719, w2717) -> (w2720:string)
                  n1034 = Build Path(base path=w2722, name or relative path=w2720) -> (appended path=w2721:path)
                  n1035 = Increment(x=w2716) -> (x+1=w2715:i32)
                }
              }
            }
            n1036 = property on="ParamVersion" class="Str"() -> ("Value"=w2589:string)  [unwired: 2 in, 2 out]
            n1037 = call "HeaderBis.vi"("UUTHeader"=w2584, "POWER SN"=w2591, "Revision Param"=w2589, "P/N UUT"=w2611, "DSP SN"=w2590, "Driver S/N"=w2614, "VR"=w2612, "Oper."=w2615, "Tester Software Ver"=w2613) -> ("table header"=w2610:string, "Array"=w2609:string[][])  [unwired: 4 in, 1 out]
            n1038 = Open/Create/Replace File(file path (use dialog)=w2651, error in=w2619, operation (0:open)=T17."create") -> (error out=w2664:errorcluster)  [unwired: 3 in, 2 out]
            n1039 = control-ref of="ATR"() -> (w2676:refnum<vi>)
            n1040 = property class="Tbl (strict)"(reference=w2676, error in=w2664) -> ("Value"=w2677:string[][])  [unwired: 2 out]
            n1041 = control-ref of="ATR"() -> (w2602:refnum<vi>)
            n1042 = call "PassFailUUT (SubVI).vi"("Table in"=w2602) -> ("PassFaileUUTresult"=w2595:bool)  [unwired: 8 in, 2 out]
            n1043 = property on="Test Failed" class="Bool (strict)"("Value"=w2595) -> ()  [unwired: 2 in, 2 out]
            n1044 = property on="PN" class="Str"() -> ("Value"=w2585:string)  [unwired: 2 in, 2 out]
            n1045 = call "MarvinReport.vi"("HEADER1"=w2610, "ATR Or"=w2676, "Steps   pfull"=w2677, "Footer UUT"=w2630, "pageNum"=3, "InputHeaderArray"=w2609, "FILE NAME"=w2653, "Report Folder"=w2651, "PN"=w2585, "REV"=w2638, "Test-Conductor"=w2615) -> ("error out"=w2625:errorcluster)  [unwired: 3 in, 1 out]
            n1046 = Select(t="PASS" ("name or relative path"), s=w2595, f="FAIL" ("name or relative path")) -> (s? t:f=w2594:string)
            n1047 = call <vilib>:"Clear Errors.vi"("error in (no error)"=w2625) -> ("error out"=w2624:errorcluster)  [unwired: 5 in, 1 out]
            n1048 = property class="Bool (strict)"(reference=w2636, error in=w2624) -> ("BoolText.Text"=w2635:string)  [unwired: 2 out]
            n1049 = Equal?(x=w2635, y="Report") -> (x = y?=w2629:bool)
            n1050 = Select(t=T3."MainProgram", s=w2629, f=T3."MainProgram") -> (s? t:f=w2632:T3)
            n1051 = call <vilib>:"Application Directory.vi"() -> ("Application Directory"=w2598:path)
            n1052 = Build Path(base path=w2598, name or relative path="data\\TestResult.ini") -> (appended path=w2601:path)
            n1053 = Select(t="Save Report...", s=w2629, f="Program Stopped...\r\nPlease turn OFF All Power sinks") -> (s? t:f=w2627:string)
            n1054 = property on="Report" class="Bool (strict)"(error in=w2624, "Value"=w2586) -> (error out=w2587:errorcluster)  [unwired: 1 in, 1 out]
            n1055 = call <vilib>:"Open Config Data.vi"("configuration file path"=w2601) -> ("error out"=w2599:errorcluster, "refnum"=w2600:T4)  [unwired: 2 in, 7 out]
            n1056 = property on="Stop Button" class="Bool (strict)"(error in=w2587, "Value"=w2586) -> ()  [unwired: 1 in, 2 out]
            n1057 = property on="Pannel User Message" class="Str"("Value"=w2627) -> ()  [unwired: 2 in, 2 out]
            n1058 = call-poly <vilib>:"Write Key.vi"("section"="Kinetics", "error in (no error)"=w2599, "value"=w2594, "key"="Result", "refnum"=w2600) -> ("error out"=w2597:errorcluster, "refnum out"=w2596:T4)  [unwired: 4 in, 1 out]
            n1059 = call <vilib>:"Close Config Data.vi"("error in (no error)"=w2597, "refnum"=w2596) -> ()  [unwired: 8 in, 2 out]
          }
          event "Help Button": Value Change {
            n1060 = event-data() -> ()  [unwired: 1 in, 6 out]
            n1061 = vi-ref "Help.vi"() -> (w2744:refnum<vi>)
            n1062 = invoke class="VI" method="FP.Open"(reference=w2744, error in=w2742, "Activate"=TRUE ("Activate?"), "State"=T15."Standard") -> (error out=w2743:errorcluster)  [unwired: 1 in, 4 out]
            n1063 = call "Help.vi"("error in"=w2743, "TesterSWVersion"=w2734) -> ("error out"=w2741:errorcluster)  [unwired: 6 in]
            n1064 = property on="Help Button" class="Bool (strict)"("Value"=FALSE ("Help Button")) -> ()  [unwired: 2 in, 2 out]
          }
          event "Serial Com": Value Change {
            n1065 = event-data() -> ()  [unwired: 1 in, 6 out]
            n1066 = property on="Serial Com" class="Bool"(error in=w2755, "Visible"=FALSE) -> (error out=w2759:errorcluster)  [unwired: 1 in, 1 out]
            n1067 = property on="VISA Kinetics" class="VISAName"(error in=w2759, "Visible"=TRUE) -> (error out=w2756:errorcluster)  [unwired: 1 in, 1 out]
          }
          event "VISA Kinetics": Value Change {
            n1068 = event-data() -> ()  [unwired: 1 in, 6 out]
            n1069 = property on="Serial Com" class="Bool"(error in=w2763, "Visible"=FALSE) -> ()  [unwired: 1 in, 2 out]
            n1070 = property on="Pannel User Message" class="Str"(error in=w2763, "Value"="Serial connection in process" ("Pannel User Message")) -> ()  [unwired: 1 in, 2 out]
          }
          event "Refresh Button": Value Change {
            n1071 = event-data() -> ()  [unwired: 1 in, 6 out]
          }
          event "Settings": Value Change {
            n1072 = event-data() -> ()  [unwired: 1 in, 6 out]
          }
        }
      }
      frame "Initialize" {
        w2807 = 0
        w2809 = FALSE ("Visible")
        w2811 = FALSE ("Visible")
        w2794 = refnum<visa-resource-name> "COMx" ("VISA resource name")
        w2798 = FALSE ("Serial Status")
        n1073 = property on="EventTimeout" class="DigNum (strict)"(error in=errorcluster {"status"=FALSE, "code"=0, "source"=""} ("error out"), "Value"=100 ("EventTimeout")) -> (error out=w2801:errorcluster)  [unwired: 1 in, 1 out]
        n1074 = property on="ComTestResult" class="Bool (strict)"("Value"=w2811) -> ()  [unwired: 2 in, 2 out]
        n1075 = property on="VenableResult" class="Bool (strict)"("Value"=w2811) -> ()  [unwired: 2 in, 2 out]
        n1076 = property on="VenableDirectionResult" class="Bool (strict)"("Value"=w2811) -> ()  [unwired: 2 in, 2 out]
        n1077 = property on="Serial Com" class="Bool"(error in=w2801, "Visible"=FALSE) -> (error out=w2817:errorcluster)  [unwired: 1 in, 1 out]
        n1078 = property on="VisualInspectionResult" class="Bool (strict)"("Value"=FALSE ("Visible")) -> ()  [unwired: 2 in, 2 out]
        n1079 = property on="VISA Kinetics" class="VISAName"(error in=w2817, "Visible"=FALSE, "Value"=w2794) -> (error out=w2803:errorcluster)  [unwired: 1 in, 1 out]
        n1080 = property on="Analogtest" class="Bool (strict)"("Value"=w2798) -> ()  [unwired: 2 in, 2 out]
        n1081 = property on="Serial Status" class="Bool (strict)"("Value"=w2798) -> ()  [unwired: 2 in, 2 out]
        n1082 = property on="Refresh Button" class="Bool (strict)"(error in=w2803, "Value"=FALSE ("Refresh Button")) -> (error out=w2804:errorcluster)  [unwired: 1 in, 1 out]
        n1083 = property on="MotorTempResult" class="Bool (strict)"("Value"=w2809) -> ()  [unwired: 2 in, 2 out]
        n1084 = property on="Automation" class="Bool (strict)"("Value"=w2809) -> ()  [unwired: 2 in, 2 out]
        n1085 = call "Find DAQ Devices.vi"("Error In"=w2804) -> ("Error Out"=w2806:errorcluster, "Stop?"=w2797:bool, "DAQmx Device Name"=w2802:tag)  [unwired: 8 in]
        n1086 = case shown="False" w2797 {
          selector: w2797 -> [_ w2837]
          tunnel: w2806 -> [w2829 w2839]
          tunnel: [w2821 w2839] -> w2795
          tunnel: w2802 -> [w2820 _]
          tunnel: [T3."Erase ATR Table" T3."Stop"] -> w2796
          frame False {
            n1087 = call <vilib>:"Clear Errors.vi"("error in (no error)"=w2829) -> ("error out"=w2828:errorcluster)  [unwired: 5 in, 1 out]
            n1088 = Not Equal?(x=w2820, y=tag "") -> (x != y?=w2830:bool)
            n1089 = case shown="True" w2830 {
              tunnel: w2820 -> [_ w2836]
              tunnel: w2828 -> [w2832 w2835]
              tunnel: [w2832 w2834] -> w2827
              frame False {
              }
              frame True {
                n1090 = call "Operation (SubVI).vi"("error in (no error)"=w2835, "Operation"=T5."Init", "DAQmx Device Name"=w2836) -> ("error out"=w2834:errorcluster)  [unwired: 8 in]
              }
            }
            n1091 = call "Operation (SubVI).vi"("error in (no error)"=w2827, "On/Off"=TRUE, "Operation"=T5."0 ohm", "DAQmx Device Name"=w2820) -> ("error out"=w2822:errorcluster)  [unwired: 7 in]
            n1092 = call "Operation (SubVI).vi"("error in (no error)"=w2822, "On/Off"=TRUE, "Operation"=T5."PowerSuply", "DAQmx Device Name"=w2820) -> ("error out"=w2821:errorcluster)  [unwired: 7 in]
            "DAQmx Device Name" <- w2820
          }
          frame True {
            n1093 = Stop(stop? (T)=w2837) -> ()
          }
        }
        n1094 = call "COM Curent Read.vi"("error in (no error)"=w2795, "VISA resource name 2"=w2794) -> ("error out"=w2792:errorcluster, "VISA Current"=w2791:refnum<visa-resource-name>)  [unwired: 7 in, 1 out]
        "VISA Current" <- w2791
        n1095 = call "ReadCurrent.vi"("error in (no error)"=w2792, "LoopFromMain"=TRUE, "VISA resource name"=w2791) -> ("error out"=w2789:errorcluster, "CurrentSens"=w2790:bool, "CurrentOut"=w2788:string)  [unwired: 6 in]
        n1096 = property on="CurrentSens" class="Bool (strict)"("Value"=w2790) -> ()  [unwired: 2 in, 2 out]
        n1097 = property on="Current" class="Str"("Value"=w2788) -> ()  [unwired: 2 in, 2 out]
        "Test Failed" <- w2798
      }
    }
  }
  n1098 = call "ATRBuild.vi"() -> ()  [unwired: 9 in, 3 out]
  n1099 = disable-structure shown="Disabled" {
    frame Disabled {
      n1100 = case shown="\"BLDC 30A\", Default" {
        selector: _ -> [_ _ _ _ _]
        tunnel: [26 26 26 26 35] -> _
        frame "BLDC 30A", Default {
        }
        frame "Warrior 60A" {
        }
        frame "Condenser Merkava" {
        }
        frame "Condenser India" {
        }
        frame "BLDC 60A" {
        }
      }
    }
    frame Enabled {
    }
  }
  n1101 = disable-structure shown="Disabled" {
    frame Disabled {
      n1102 = control-ref of="Stop Button"() -> ()  [unwired: 1 out]
      n1103 = control-ref of="UUT"() -> ()  [unwired: 1 out]
      n1104 = property on="UUT" class="Str" props=["Value"]() -> ()  [unwired: 2 in, 3 out]
      n1105 = control-ref of="UUT"() -> ()  [unwired: 1 out]
      n1106 = property on="UUT" class="DigNum (strict)" props=["Value"]() -> ()  [unwired: 2 in, 3 out]
      n1107 = control-ref of="Motor Speed RPM Serial"() -> ()  [unwired: 1 out]
      n1108 = call "Find_Number_LineMARVIN.vi"() -> ()  [unwired: 5 in, 4 out]
      n1109 = control-ref of="Pannel User Message"() -> ()  [unwired: 1 out]
      n1110 = call "Write panel message Kinetics (SubVI).vi"() -> ()  [unwired: 10 in, 2 out]
      n1111 = local read "DAQmx Device Name"() -> (w2846:tag)
      n1112 = control-ref of="ATR"() -> ()  [unwired: 1 out]
      n1113 = call "PassOrFail (SubVI).vi"() -> ()  [unwired: 11 in, 1 out]
      n1114 = call "Serial.vi"("write buffer"="EP=1\r\nVC=1000\r\n") -> ()  [unwired: 9 in, 2 out]
      n1115 = call "Operation (SubVI).vi"("DAQmx Device Name"=w2846) -> ()  [unwired: 10 in, 1 out]
      n1116 = property on="UUT" class="Str" props=["Value"]() -> ()  [unwired: 2 in, 3 out]
    }
    frame Enabled {
    }
  }
  n1117 = disable-structure shown="Disabled" {
    frame Disabled {
      w2847 = T13."Disabled and Grayed Out" ("Disabled")
      w2848 = FALSE ("Start")
      n1118 = property on="Current SN" class="DigNum (strict)" props=["Value"]() -> ()  [unwired: 2 in, 3 out]
      n1119 = property on="UUT" class="DigNum (strict)" props=["Value"]() -> ()  [unwired: 2 in, 3 out]
      n1120 = property on="Serial Status" class="Bool (strict)" props=["Value"]() -> ()  [unwired: 2 in, 3 out]
      n1121 = property on="UUT SoftwareVer" class="Str" props=["Value"]() -> ()  [unwired: 2 in, 3 out]
      n1122 = call "Operation (SubVI).vi"() -> ()  [unwired: 11 in, 1 out]
      n1123 = property on="Next SN" class="DigNum (strict)" props=["Value"]() -> ()  [unwired: 3 in, 2 out]
      n1124 = property on="Start" class="Bool (strict)"("Value"=w2848, "DisabledEnum"=w2847) -> ()  [unwired: 2 in, 2 out]
      n1125 = property on="Report" class="Bool (strict)"("Value"=w2848, "DisabledEnum"=w2847) -> ()  [unwired: 2 in, 2 out]
    }
    frame Enabled {
    }
  }
  "Pannel User Message" <- w17
